vi "Hardware-DI-A-Host.vi"() -> ()   [LabVIEW 2016]
uses:
  <vilib>/Powertrain Controls/Device Drivers/DCM/Rev0/UI/Bank A.ctl
  Shared/Typedefs/DI-Phase-Array-2D.ctl
  <vilib>/Powertrain Controls/Device Drivers/DCM/DI/RT/Phase.ctl
  <vilib>/Powertrain Controls/Device Drivers/DCM/Rev0/FPGA/DI - Drive State.ctl
  <vilib>/Powertrain Controls/Device Drivers/DCM/DI/FPGA/Phase Step.ctl
  <vilib>/Powertrain Controls/Device Drivers/DCM/DI/FPGA/Control.ctl
  <vilib>/Powertrain Controls/Device Drivers/DCM/Rev0/RT/Configuration.ctl
  <vilib>/Powertrain Controls/Device Drivers/DCM/Rev0/FPGA/DI - Bank Configuration.ctl
  Host SubVIs/DI Command Element.ctl
  <vilib>/Powertrain Controls/Device Drivers/DCM/Rev0/FPGA/Digital Channel.ctl
  Shared/Typedefs/DI-Command-Array.ctl
  <vilib>/Powertrain Controls/Device Drivers/DCM/DI/RT/Command.ctl
  <vilib>/Powertrain Controls/Device Drivers/DCM/DI/FPGA/Mode.ctl
  <vilib>/Powertrain Controls/Device Drivers/DCM/DI/RT/Command Sequence.ctl
  <vilib>/Powertrain Controls/Device Drivers/DCM/DI/RT/Angle Control.ctl
  Shared/Typedefs/DI-Phase-Array-1D.ctl
  <vilib>/addons/Software Calibration Management/XControls/SubHost.xctl
  <vilib>/Powertrain Controls/Device Drivers/DCM/Rev0/FPGA/DI - Faults.ctl
  Host SubVIs/Pump Command Element.ctl
  <vilib>/Powertrain Controls/Device Drivers/DCM/Rev0/FPGA/DI - ADC Signals.ctl
  <vilib>/Powertrain Controls/Device Drivers/DCM/DI/FPGA/Capture Event.ctl
  <vilib>/Powertrain Controls/Device Drivers/DCM/Rev0/RT/System State.ctl
  <vilib>/Powertrain Controls/Device Drivers/DCM/Rev0/RT/System ADC.ctl
  <vilib>/Powertrain Controls/Device Drivers/DCM/Rev0/RT/Internal Fault.ctl
  <vilib>/Powertrain Controls/Device Drivers/DCM/Rev0/RT/Run State.ctl
  <vilib>/Powertrain Controls/Device Drivers/DCM/Rev0/UI/Configuration.ctl
  <vilib>/Powertrain Controls/Device Drivers/DCM/Rev0/UI/System Configuration.ctl
  <vilib>/Powertrain Controls/Device Drivers/DCM/Rev0/UI/Injector Configuration.ctl
  <vilib>/Powertrain Controls/Device Drivers/DCM/Rev0/UI/Test Comparators.vi
  <vilib>/Powertrain Controls/Device Drivers/DCM/Rev0/UI/DAC Delay.vi
  <vilib>/Powertrain Controls/Device Drivers/DCM/DI/RT/Phase Convert.vi
  <vilib>/Powertrain Controls/Device Drivers/DCM/DI/RT/Skew.vi
  <vilib>/Powertrain Controls/Device Drivers/DCM/Rev0/UI/Calibrations.vi
  <vilib>/Powertrain Controls/Device Drivers/DCM/Rev0/UI/One Injection Command.vi
  <vilib>/Powertrain Controls/Device Drivers/DCM/DI/FPGA/Simulate Phase Array.vi
  <vilib>/Powertrain Controls/Device Drivers/DCM/Rev0/FPGA/DI - Setpoints.vi
  <vilib>/Powertrain Controls/Device Drivers/DCM/Rev0/UI/Phase State Control.vi
  <vilib>/Powertrain Controls/Device Drivers/DCM/Rev0/UI/Circuit Model Step.vi
  <vilib>/Powertrain Controls/Device Drivers/DCM/Rev0/UI/FET Movie Data.vi
  <vilib>/Powertrain Controls/Device Drivers/DCM/DI/FPGA/DCM - FPGA - DI.lvlib
  <vilib>/Powertrain Controls/Device Drivers/DCM/Rev0/UI/DCM - UI.lvlib
  <vilib>/Powertrain Controls/Device Drivers/DCM/Rev0/FPGA/DCM - FPGA.lvlib
  <vilib>/Powertrain Controls/Device Drivers/DCM/DI/RT/DCM - RT - DI.lvlib
  <vilib>/Powertrain Controls/Device Drivers/DCM/Rev0/RT/DCM - RT.lvclass
  Shared/DSI-Shared.lvlib
panel:
  out "RunState":T1
  out "_BoostSlider":cluster{dbl, dbl, dbl, dbl}(slide)={0.0, 166.94117647058823, 117.76470588235294, 190.23529411764707} scale=0.0..220.0
  out "_Bank A Status":T2 caption="Injector and Pump Simulation Settings" {"Boost Clamp [V]" format="%#_3p"; "Ext HV [V]" format="%#_3p"; "DRVP [V]" format="%#_3p"; "Pump Zener [V]" format="%#_3p"; "DI Zener [V]" format="%#_3p"; "Secondary 3-4 [V]" format="%#_3p"; "Secondary 1-2 [V]" format="%#_3p"; "Primary 3-4 [V]" format="%#_3p"; "Primary 1-2 [V]" format="%#_3p"}
  in  "_DI Bank_Configuration":T3 caption="DI Bank A_Configuration" {"Pump Zener Voltage [V]" min=0 max=240 format="%#_13g"; "DI Zener Voltage [V]" min=0 max=100 format="%#_13g"; "Boost Clamp [V]" min=0 max=220 format="%#_13g"; "Boost Voltage [V]" min=0 max=220 format="%#_13g"}
  in  "DI Scope":T5(xcontrol)
  in  "UserOS":bool
  in  "UserOSTime":sgl caption="[s]" format="%#.3p"
  in  "_Hidden Items":enum32{"DI-A Configurations Items"}(tab)
  out "dt":sgl=13.7
  out "_Bank A?":bool
  in  "_Redraw Slider":bool
  out "SYS|Exec|CalLoading":bool
  in  "_Refresh All":bool
  in  "_Redraw Pump Command":bool
  in  "_Redraw DI Command":bool
  in  "InjCmd":T6=[{"Mode"=enum."Off", "Digital Input"=enum."Unused", "Default Profile Index"=0, "Cal Freq [Hz]"=0.0, "Cal Duration [s]"=0.0, "Cal Increment [s]"=0.0, "Cal Pulses"=0, "TMP Command Sequence"=[{"Duration [s]"=0.0, "Level"=FALSE, "Run/Stop"=FALSE, "Profile Index"=0}, {"Duration [s]"=0.0, "Level"=FALSE, "Run/Stop"=FALSE, "Profile Index"=0}, {"Duration [s]"=0.0, "Level"=FALSE, "Run/Stop"=FALSE, "Profile Index"=0}, {"Duration [s]"=0.0, "Level"=FALSE, "Run/Stop"=FALSE, "Profile Index"=0}, {"Duration [s]"=0.0, "Level"=FALSE, "Run/Stop"=FALSE, "Profile Index"=0}, {"Duration [s]"=0.0, "Level"=FALSE, "Run/Stop"=FALSE, "Profile Index"=0}, {"Duration [s]"=0.0, "Level"=FALSE, "Run/Stop"=FALSE, "Profile Index"=0}, {"Duration [s]"=0.0, "Level"=FALSE, "Run/Stop"=FALSE, "Profile Index"=0}], "EPT TDC Offset [CAD]"=0.0, "EPT Window Start [DBTDC]"=0.0, "EPT Window End [DBTDC]"=0.0, "EPT Angles"=[{"Enable"=FALSE, "Timing [DBTDC]"=0.0, "Duration [s]"=0.0, "Profile Index"=0}, {"Enable"=FALSE, "Timing [DBTDC]"=0.0, "Duration [s]"=0.0, "Profile Index"=0}, {"Enable"=FALSE, "Timing [DBTDC]"=0.0, "Duration [s]"=0.0, "Profile Index"=0}, {"Enable"=FALSE, "Timing [DBTDC]"=0.0, "Duration [s]"=0.0, "Profile Index"=0}], "EPT Skip Fire"=FALSE, "EPT Skip Index"=0, "EPT Precharge Duration [s]"=0.0, "EPT Precharge Profile Index"=0}, {"Mode"=enum."Off", "Digital Input"=enum."Unused", "Default Profile Index"=0, "Cal Freq [Hz]"=0.0, "Cal Duration [s]"=0.0, "Cal Increment [s]"=0.0, "Cal Pulses"=0, "TMP Command Sequence"=[{"Duration [s]"=0.0, "Level"=FALSE, "Run/Stop"=FALSE, "Profile Index"=0}, {"Duration [s]"=0.0, "Level"=FALSE, "Run/Stop"=FALSE, "Profile Index"=0}, {"Duration [s]"=0.0, "Level"=FALSE, "Run/Stop"=FALSE, "Profile Index"=0}, {"Duration [s]"=0.0, "Level"=FALSE, "Run/Stop"=FALSE, "Profile Index"=0}, {"Duration [s]"=0.0, "Level"=FALSE, "Run/Stop"=FALSE, "Profile Index"=0}, {"Duration [s]"=0.0, "Level"=FALSE, "Run/Stop"=FALSE, "Profile Index"=0}, {"Duration [s]"=0.0, "Level"=FALSE, "Run/Stop"=FALSE, "Profile Index"=0}, {"Duration [s]"=0.0, "Level"=FALSE, "Run/Stop"=FALSE, "Profile Index"=0}], "EPT TDC Offset [CAD]"=0.0, "EPT Window Start [DBTDC]"=0.0, "EPT Window End [DBTDC]"=0.0, "EPT Angles"=[{"Enable"=FALSE, "Timing [DBTDC]"=0.0, "Duration [s]"=0.0, "Profile Index"=0}, {"Enable"=FALSE, "Timing [DBTDC]"=0.0, "Duration [s]"=0.0, "Profile Index"=0}, {"Enable"=FALSE, "Timing [DBTDC]"=0.0, "Duration [s]"=0.0, "Profile Index"=0}, {"Enable"=FALSE, "Timing [DBTDC]"=0.0, "Duration [s]"=0.0, "Profile Index"=0}], "EPT Skip Fire"=FALSE, "EPT Skip Index"=0, "EPT Precharge Duration [s]"=0.0, "EPT Precharge Profile Index"=0}, {"Mode"=enum."Off", "Digital Input"=enum."Unused", "Default Profile Index"=0, "Cal Freq [Hz]"=0.0, "Cal Duration [s]"=0.0, "Cal Increment [s]"=0.0, "Cal Pulses"=0, "TMP Command Sequence"=[{"Duration [s]"=0.0, "Level"=FALSE, "Run/Stop"=FALSE, "Profile Index"=0}, {"Duration [s]"=0.0, "Level"=FALSE, "Run/Stop"=FALSE, "Profile Index"=0}, {"Duration [s]"=0.0, "Level"=FALSE, "Run/Stop"=FALSE, "Profile Index"=0}, {"Duration [s]"=0.0, "Level"=FALSE, "Run/Stop"=FALSE, "Profile Index"=0}, {"Duration [s]"=0.0, "Level"=FALSE, "Run/Stop"=FALSE, "Profile Index"=0}, {"Duration [s]"=0.0, "Level"=FALSE, "Run/Stop"=FALSE, "Profile Index"=0}, {"Duration [s]"=0.0, "Level"=FALSE, "Run/Stop"=FALSE, "Profile Index"=0}, {"Duration [s]"=0.0, "Level"=FALSE, "Run/Stop"=FALSE, "Profile Index"=0}], "EPT TDC Offset [CAD]"=0.0, "EPT Window Start [DBTDC]"=0.0, "EPT Window End [DBTDC]"=0.0, "EPT Angles"=[{"Enable"=FALSE, "Timing [DBTDC]"=0.0, "Duration [s]"=0.0, "Profile Index"=0}, {"Enable"=FALSE, "Timing [DBTDC]"=0.0, "Duration [s]"=0.0, "Profile Index"=0}, {"Enable"=FALSE, "Timing [DBTDC]"=0.0, "Duration [s]"=0.0, "Profile Index"=0}, {"Enable"=FALSE, "Timing [DBTDC]"=0.0, "Duration [s]"=0.0, "Profile Index"=0}], "EPT Skip Fire"=FALSE, "EPT Skip Index"=0, "EPT Precharge Duration [s]"=0.0, "EPT Precharge Profile Index"=0}, {"Mode"=enum."Off", "Digital Input"=enum."Unused", "Default Profile Index"=0, "Cal Freq [Hz]"=0.0, "Cal Duration [s]"=0.0, "Cal Increment [s]"=0.0, "Cal Pulses"=0, "TMP Command Sequence"=[{"Duration [s]"=0.0, "Level"=FALSE, "Run/Stop"=FALSE, "Profile Index"=0}, {"Duration [s]"=0.0, "Level"=FALSE, "Run/Stop"=FALSE, "Profile Index"=0}, {"Duration [s]"=0.0, "Level"=FALSE, "Run/Stop"=FALSE, "Profile Index"=0}, {"Duration [s]"=0.0, "Level"=FALSE, "Run/Stop"=FALSE, "Profile Index"=0}, {"Duration [s]"=0.0, "Level"=FALSE, "Run/Stop"=FALSE, "Profile Index"=0}, {"Duration [s]"=0.0, "Level"=FALSE, "Run/Stop"=FALSE, "Profile Index"=0}, {"Duration [s]"=0.0, "Level"=FALSE, "Run/Stop"=FALSE, "Profile Index"=0}, {"Duration [s]"=0.0, "Level"=FALSE, "Run/Stop"=FALSE, "Profile Index"=0}], "EPT TDC Offset [CAD]"=0.0, "EPT Window Start [DBTDC]"=0.0, "EPT Window End [DBTDC]"=0.0, "EPT Angles"=[{"Enable"=FALSE, "Timing [DBTDC]"=0.0, "Duration [s]"=0.0, "Profile Index"=0}, {"Enable"=FALSE, "Timing [DBTDC]"=0.0, "Duration [s]"=0.0, "Profile Index"=0}, {"Enable"=FALSE, "Timing [DBTDC]"=0.0, "Duration [s]"=0.0, "Profile Index"=0}, {"Enable"=FALSE, "Timing [DBTDC]"=0.0, "Duration [s]"=0.0, "Profile Index"=0}], "EPT Skip Fire"=FALSE, "EPT Skip Index"=0, "EPT Precharge Duration [s]"=0.0, "EPT Precharge Profile Index"=0}, {"Mode"=enum."Off", "Digital Input"=enum."Unused", "Default Profile Index"=0, "Cal Freq [Hz]"=0.0, "Cal Duration [s]"=0.0, "Cal Increment [s]"=0.0, "Cal Pulses"=0, "TMP Command Sequence"=[{"Duration [s]"=0.0, "Level"=FALSE, "Run/Stop"=FALSE, "Profile Index"=0}, {"Duration [s]"=0.0, "Level"=FALSE, "Run/Stop"=FALSE, "Profile Index"=0}, {"Duration [s]"=0.0, "Level"=FALSE, "Run/Stop"=FALSE, "Profile Index"=0}, {"Duration [s]"=0.0, "Level"=FALSE, "Run/Stop"=FALSE, "Profile Index"=0}, {"Duration [s]"=0.0, "Level"=FALSE, "Run/Stop"=FALSE, "Profile Index"=0}, {"Duration [s]"=0.0, "Level"=FALSE, "Run/Stop"=FALSE, "Profile Index"=0}, {"Duration [s]"=0.0, "Level"=FALSE, "Run/Stop"=FALSE, "Profile Index"=0}, {"Duration [s]"=0.0, "Level"=FALSE, "Run/Stop"=FALSE, "Profile Index"=0}], "EPT TDC Offset [CAD]"=0.0, "EPT Window Start [DBTDC]"=0.0, "EPT Window End [DBTDC]"=0.0, "EPT Angles"=[{"Enable"=FALSE, "Timing [DBTDC]"=0.0, "Duration [s]"=0.0, "Profile Index"=0}, {"Enable"=FALSE, "Timing [DBTDC]"=0.0, "Duration [s]"=0.0, "Profile Index"=0}, {"Enable"=FALSE, "Timing [DBTDC]"=0.0, "Duration [s]"=0.0, "Profile Index"=0}, {"Enable"=FALSE, "Timing [DBTDC]"=0.0, "Duration [s]"=0.0, "Profile Index"=0}], "EPT Skip Fire"=FALSE, "EPT Skip Index"=0, "EPT Precharge Duration [s]"=0.0, "EPT Precharge Profile Index"=0}, {"Mode"=enum."Off", "Digital Input"=enum."Unused", "Default Profile Index"=0, "Cal Freq [Hz]"=0.0, "Cal Duration [s]"=0.0, "Cal Increment [s]"=0.0, "Cal Pulses"=0, "TMP Command Sequence"=[{"Duration [s]"=0.0, "Level"=FALSE, "Run/Stop"=FALSE, "Profile Index"=0}, {"Duration [s]"=0.0, "Level"=FALSE, "Run/Stop"=FALSE, "Profile Index"=0}, {"Duration [s]"=0.0, "Level"=FALSE, "Run/Stop"=FALSE, "Profile Index"=0}, {"Duration [s]"=0.0, "Level"=FALSE, "Run/Stop"=FALSE, "Profile Index"=0}, {"Duration [s]"=0.0, "Level"=FALSE, "Run/Stop"=FALSE, "Profile Index"=0}, {"Duration [s]"=0.0, "Level"=FALSE, "Run/Stop"=FALSE, "Profile Index"=0}, {"Duration [s]"=0.0, "Level"=FALSE, "Run/Stop"=FALSE, "Profile Index"=0}, {"Duration [s]"=0.0, "Level"=FALSE, "Run/Stop"=FALSE, "Profile Index"=0}], "EPT TDC Offset [CAD]"=0.0, "EPT Window Start [DBTDC]"=0.0, "EPT Window End [DBTDC]"=0.0, "EPT Angles"=[{"Enable"=FALSE, "Timing [DBTDC]"=0.0, "Duration [s]"=0.0, "Profile Index"=0}, {"Enable"=FALSE, "Timing [DBTDC]"=0.0, "Duration [s]"=0.0, "Profile Index"=0}, {"Enable"=FALSE, "Timing [DBTDC]"=0.0, "Duration [s]"=0.0, "Profile Index"=0}, {"Enable"=FALSE, "Timing [DBTDC]"=0.0, "Duration [s]"=0.0, "Profile Index"=0}], "EPT Skip Fire"=FALSE, "EPT Skip Index"=0, "EPT Precharge Duration [s]"=0.0, "EPT Precharge Profile Index"=0}, {"Mode"=enum."Off", "Digital Input"=enum."Unused", "Default Profile Index"=0, "Cal Freq [Hz]"=0.0, "Cal Duration [s]"=0.0, "Cal Increment [s]"=0.0, "Cal Pulses"=0, "TMP Command Sequence"=[{"Duration [s]"=0.0, "Level"=FALSE, "Run/Stop"=FALSE, "Profile Index"=0}, {"Duration [s]"=0.0, "Level"=FALSE, "Run/Stop"=FALSE, "Profile Index"=0}, {"Duration [s]"=0.0, "Level"=FALSE, "Run/Stop"=FALSE, "Profile Index"=0}, {"Duration [s]"=0.0, "Level"=FALSE, "Run/Stop"=FALSE, "Profile Index"=0}, {"Duration [s]"=0.0, "Level"=FALSE, "Run/Stop"=FALSE, "Profile Index"=0}, {"Duration [s]"=0.0, "Level"=FALSE, "Run/Stop"=FALSE, "Profile Index"=0}, {"Duration [s]"=0.0, "Level"=FALSE, "Run/Stop"=FALSE, "Profile Index"=0}, {"Duration [s]"=0.0, "Level"=FALSE, "Run/Stop"=FALSE, "Profile Index"=0}], "EPT TDC Offset [CAD]"=0.0, "EPT Window Start [DBTDC]"=0.0, "EPT Window End [DBTDC]"=0.0, "EPT Angles"=[{"Enable"=FALSE, "Timing [DBTDC]"=0.0, "Duration [s]"=0.0, "Profile Index"=0}, {"Enable"=FALSE, "Timing [DBTDC]"=0.0, "Duration [s]"=0.0, "Profile Index"=0}, {"Enable"=FALSE, "Timing [DBTDC]"=0.0, "Duration [s]"=0.0, "Profile Index"=0}, {"Enable"=FALSE, "Timing [DBTDC]"=0.0, "Duration [s]"=0.0, "Profile Index"=0}], "EPT Skip Fire"=FALSE, "EPT Skip Index"=0, "EPT Precharge Duration [s]"=0.0, "EPT Precharge Profile Index"=0}, {"Mode"=enum."Off", "Digital Input"=enum."Unused", "Default Profile Index"=0, "Cal Freq [Hz]"=0.0, "Cal Duration [s]"=0.0, "Cal Increment [s]"=0.0, "Cal Pulses"=0, "TMP Command Sequence"=[{"Duration [s]"=0.0, "Level"=FALSE, "Run/Stop"=FALSE, "Profile Index"=0}, {"Duration [s]"=0.0, "Level"=FALSE, "Run/Stop"=FALSE, "Profile Index"=0}, {"Duration [s]"=0.0, "Level"=FALSE, "Run/Stop"=FALSE, "Profile Index"=0}, {"Duration [s]"=0.0, "Level"=FALSE, "Run/Stop"=FALSE, "Profile Index"=0}, {"Duration [s]"=0.0, "Level"=FALSE, "Run/Stop"=FALSE, "Profile Index"=0}, {"Duration [s]"=0.0, "Level"=FALSE, "Run/Stop"=FALSE, "Profile Index"=0}, {"Duration [s]"=0.0, "Level"=FALSE, "Run/Stop"=FALSE, "Profile Index"=0}, {"Duration [s]"=0.0, "Level"=FALSE, "Run/Stop"=FALSE, "Profile Index"=0}], "EPT TDC Offset [CAD]"=0.0, "EPT Window Start [DBTDC]"=0.0, "EPT Window End [DBTDC]"=0.0, "EPT Angles"=[{"Enable"=FALSE, "Timing [DBTDC]"=0.0, "Duration [s]"=0.0, "Profile Index"=0}, {"Enable"=FALSE, "Timing [DBTDC]"=0.0, "Duration [s]"=0.0, "Profile Index"=0}, {"Enable"=FALSE, "Timing [DBTDC]"=0.0, "Duration [s]"=0.0, "Profile Index"=0}, {"Enable"=FALSE, "Timing [DBTDC]"=0.0, "Duration [s]"=0.0, "Profile Index"=0}], "EPT Skip Fire"=FALSE, "EPT Skip Index"=0, "EPT Precharge Duration [s]"=0.0, "EPT Precharge Profile Index"=0}] {"EPT Precharge Profile Index" max=15; "EPT Precharge Duration [s]" min=0 format="%#_4p"; "Default Profile Index" max=15; "Cal Increment [s]" format="%#_3p"; "TMP Command Sequence"."Profile Index" max=7; "TMP Command Sequence"."Duration [s]" min=0 max=100 format="%#_3p"; "Cal Pulses" max=511; "EPT Skip Index" max=7; "EPT Angles"."Profile Index" max=7; "EPT Angles"."Duration [s]" min=0 max=100 format="%#_3p"; "Cal Duration [s]" format="%#_3p"; "Cal Freq [Hz]" format="%#_3p"}
  in  "ChanSelect4":u8(ring) items=["I LS A1/A5", "I LS A2/A6", "I LS A3/A7", "I LS A4", "I LS A8/PumpA", "V PZ A1", "V PZ A2", "V PZ A3", "V PZ A4", "V S A1", "V S A2", "V S A3", "V S A4", "V S A5", "V S A6", "V S A7", "V S A8", "V Pump A", "V Secondary A1A2", "V Secondary A3A4", "V Ext HV A", "------------------------ ", "I LS B1/B5", "I LS B2/B6", "I LS B3/B7", "I LS B4", "I LS B8/PumpB", "V PZ B1", "V PZ B2", "V PZ B3", "V PZ B4", "V S B1", "V S B2", "V S B3", "V S B4", "V S B5", "V S B6", "V S B7", "V S B8", "V Pump B", "V Secondary B1B2", "V Secondary B3B4", "V Ext HV B", "-------------------------  ", "AI 1", "AI 2", "AI 3", "AI 4", "AI 5", "AI 6", "AI 7", "AI 8", "AI 9", "AI 10", "AI 11", "AI 12", "-------------------------   ", "V DRVP"]
  in  "ChanSelect3":u8(ring) items=["I LS A1/A5", "I LS A2/A6", "I LS A3/A7", "I LS A4", "I LS A8/PumpA", "V PZ A1", "V PZ A2", "V PZ A3", "V PZ A4", "V S A1", "V S A2", "V S A3", "V S A4", "V S A5", "V S A6", "V S A7", "V S A8", "V Pump A", "V Secondary A1A2", "V Secondary A3A4", "V Ext HV A", "------------------------ ", "I LS B1/B5", "I LS B2/B6", "I LS B3/B7", "I LS B4", "I LS B8/PumpB", "V PZ B1", "V PZ B2", "V PZ B3", "V PZ B4", "V S B1", "V S B2", "V S B3", "V S B4", "V S B5", "V S B6", "V S B7", "V S B8", "V Pump B", "V Secondary B1B2", "V Secondary B3B4", "V Ext HV B", "-------------------------  ", "AI 1", "AI 2", "AI 3", "AI 4", "AI 5", "AI 6", "AI 7", "AI 8", "AI 9", "AI 10", "AI 11", "AI 12", "-------------------------   ", "V DRVP"]
  in  "_Redraw Profiles Usage Tracker":bool
  in  "_Redraw Pump Timing Plot":bool
  in  "InjectEnable":bool
  in  "PSEnable":bool
  in  "Configuration":u8
  in  "BoostV":sgl format="%#_13g"
  in  "ZenerV":sgl format="%#_13g"
  in  "ZenerEnable":bool
  in  "PumpZenerV":sgl format="%#_13g"
  in  "BoostClampV":sgl format="%#_13g"
  in  "_Redraw Phase":bool
  in  "_Redraw Phase Plot":bool
  in  "_Redraw Phase Lists":bool
  in  "_Redraw Pump Phase Plot":bool
  in  "_Redraw Pump Phase List":bool
  in  "FaultClear":u8
  in  "ChanSelect2":u8(ring) items=["I LS A1/A5", "I LS A2/A6", "I LS A3/A7", "I LS A4", "I LS A8/PumpA", "V PZ A1", "V PZ A2", "V PZ A3", "V PZ A4", "V S A1", "V S A2", "V S A3", "V S A4", "V S A5", "V S A6", "V S A7", "V S A8", "V Pump A", "V Secondary A1A2", "V Secondary A3A4", "V Ext HV A", "------------------------ ", "I LS B1/B5", "I LS B2/B6", "I LS B3/B7", "I LS B4", "I LS B8/PumpB", "V PZ B1", "V PZ B2", "V PZ B3", "V PZ B4", "V S B1", "V S B2", "V S B3", "V S B4", "V S B5", "V S B6", "V S B7", "V S B8", "V Pump B", "V Secondary B1B2", "V Secondary B3B4", "V Ext HV B", "-------------------------  ", "AI 1", "AI 2", "AI 3", "AI 4", "AI 5", "AI 6", "AI 7", "AI 8", "AI 9", "AI 10", "AI 11", "AI 12", "-------------------------   ", "V DRVP"]
  in  "ChanSelect1":u8(ring) items=["I LS A1/A5", "I LS A2/A6", "I LS A3/A7", "I LS A4", "I LS A8/PumpA", "V PZ A1", "V PZ A2", "V PZ A3", "V PZ A4", "V S A1", "V S A2", "V S A3", "V S A4", "V S A5", "V S A6", "V S A7", "V S A8", "V Pump A", "V Secondary A1A2", "V Secondary A3A4", "V Ext HV A", "------------------------ ", "I LS B1/B5", "I LS B2/B6", "I LS B3/B7", "I LS B4", "I LS B8/PumpB", "V PZ B1", "V PZ B2", "V PZ B3", "V PZ B4", "V S B1", "V S B2", "V S B3", "V S B4", "V S B5", "V S B6", "V S B7", "V S B8", "V Pump B", "V Secondary B1B2", "V Secondary B3B4", "V Ext HV B", "-------------------------  ", "AI 1", "AI 2", "AI 3", "AI 4", "AI 5", "AI 6", "AI 7", "AI 8", "AI 9", "AI 10", "AI 11", "AI 12", "-------------------------   ", "V DRVP"]
  in  "ScopeEnable":bool
  in  "ScopeEvent":u8(ring) items=["Unused", "Injector A1", "Injector A2", "Injector A3", "Injector A4", "Injector A5", "Injector A6", "Injector A7", "Injector A8/PumpA", "Injector B1", "Injector B2", "Injector B3", "Injector B4", "Injector B5", "Injector B6", "Injector B7", "Injector B8/PumpB", "Diff IO 1", "Diff IO 2", "Diff IO 3", "Diff IO 4", "Diff IO 5", "Diff IO 6", "Diff IO 7", "Diff IO 8", "Aux 1", "Aux 2", "Aux 3", "Aux 4", "Aux 5", "Aux 6", "Aux 7", "Aux 8", "User OS"]
  out "Data":sgl[][](array[numeric])
  out "_Ref Pump Profiles":cluster{"Array":dbl[], "Array":dbl[]}[](array[cluster])
  out "_Ref Inj Profiles":cluster{"Array":dbl[], "Array":dbl[]}[](array[cluster])
  out "_SimuXY":cluster{"Array":dbl[], "Array":dbl[]}[](array[cluster])
  in  "PumpPhase":T12=[{"Drive"=enum."Idle", "Direction"=FALSE, "Phase Step"=enum."Duration", "Duration [s]"=0.0, "Current High [A]"=0.0, "Current Low [A]"=0.0, "Voltage High [V]"=0.0, "Voltage Low [V]"=0.0, "Change"=FALSE, "Current Control"=enum."Closed Loop", "Period [s]"=0.0, "Pulse Width [s]"=0.0, "Profile"=0, "Voltage Control"=FALSE}, {"Drive"=enum."Idle", "Direction"=FALSE, "Phase Step"=enum."Duration", "Duration [s]"=0.0, "Current High [A]"=0.0, "Current Low [A]"=0.0, "Voltage High [V]"=0.0, "Voltage Low [V]"=0.0, "Change"=FALSE, "Current Control"=enum."Closed Loop", "Period [s]"=0.0, "Pulse Width [s]"=0.0, "Profile"=0, "Voltage Control"=FALSE}, {"Drive"=enum."Idle", "Direction"=FALSE, "Phase Step"=enum."Duration", "Duration [s]"=0.0, "Current High [A]"=0.0, "Current Low [A]"=0.0, "Voltage High [V]"=0.0, "Voltage Low [V]"=0.0, "Change"=FALSE, "Current Control"=enum."Closed Loop", "Period [s]"=0.0, "Pulse Width [s]"=0.0, "Profile"=0, "Voltage Control"=FALSE}, {"Drive"=enum."Idle", "Direction"=FALSE, "Phase Step"=enum."Duration", "Duration [s]"=0.0, "Current High [A]"=0.0, "Current Low [A]"=0.0, "Voltage High [V]"=0.0, "Voltage Low [V]"=0.0, "Change"=FALSE, "Current Control"=enum."Closed Loop", "Period [s]"=0.0, "Pulse Width [s]"=0.0, "Profile"=0, "Voltage Control"=FALSE}, {"Drive"=enum."Idle", "Direction"=FALSE, "Phase Step"=enum."Duration", "Duration [s]"=0.0, "Current High [A]"=0.0, "Current Low [A]"=0.0, "Voltage High [V]"=0.0, "Voltage Low [V]"=0.0, "Change"=FALSE, "Current Control"=enum."Closed Loop", "Period [s]"=0.0, "Pulse Width [s]"=0.0, "Profile"=0, "Voltage Control"=FALSE}, {"Drive"=enum."Idle", "Direction"=FALSE, "Phase Step"=enum."Duration", "Duration [s]"=0.0, "Current High [A]"=0.0, "Current Low [A]"=0.0, "Voltage High [V]"=0.0, "Voltage Low [V]"=0.0, "Change"=FALSE, "Current Control"=enum."Closed Loop", "Period [s]"=0.0, "Pulse Width [s]"=0.0, "Profile"=0, "Voltage Control"=FALSE}, {"Drive"=enum."Idle", "Direction"=FALSE, "Phase Step"=enum."Duration", "Duration [s]"=0.0, "Current High [A]"=0.0, "Current Low [A]"=0.0, "Voltage High [V]"=0.0, "Voltage Low [V]"=0.0, "Change"=FALSE, "Current Control"=enum."Closed Loop", "Period [s]"=0.0, "Pulse Width [s]"=0.0, "Profile"=0, "Voltage Control"=FALSE}, {"Drive"=enum."Idle", "Direction"=FALSE, "Phase Step"=enum."Duration", "Duration [s]"=0.0, "Current High [A]"=0.0, "Current Low [A]"=0.0, "Voltage High [V]"=0.0, "Voltage Low [V]"=0.0, "Change"=FALSE, "Current Control"=enum."Closed Loop", "Period [s]"=0.0, "Pulse Width [s]"=0.0, "Profile"=0, "Voltage Control"=FALSE}, {"Drive"=enum."Idle", "Direction"=FALSE, "Phase Step"=enum."Duration", "Duration [s]"=0.0, "Current High [A]"=0.0, "Current Low [A]"=0.0, "Voltage High [V]"=0.0, "Voltage Low [V]"=0.0, "Change"=FALSE, "Current Control"=enum."Closed Loop", "Period [s]"=0.0, "Pulse Width [s]"=0.0, "Profile"=0, "Voltage Control"=FALSE}, {"Drive"=enum."Idle", "Direction"=FALSE, "Phase Step"=enum."Duration", "Duration [s]"=0.0, "Current High [A]"=0.0, "Current Low [A]"=0.0, "Voltage High [V]"=0.0, "Voltage Low [V]"=0.0, "Change"=FALSE, "Current Control"=enum."Closed Loop", "Period [s]"=0.0, "Pulse Width [s]"=0.0, "Profile"=0, "Voltage Control"=FALSE}, {"Drive"=enum."Idle", "Direction"=FALSE, "Phase Step"=enum."Duration", "Duration [s]"=0.0, "Current High [A]"=0.0, "Current Low [A]"=0.0, "Voltage High [V]"=0.0, "Voltage Low [V]"=0.0, "Change"=FALSE, "Current Control"=enum."Closed Loop", "Period [s]"=0.0, "Pulse Width [s]"=0.0, "Profile"=0, "Voltage Control"=FALSE}, {"Drive"=enum."Idle", "Direction"=FALSE, "Phase Step"=enum."Duration", "Duration [s]"=0.0, "Current High [A]"=0.0, "Current Low [A]"=0.0, "Voltage High [V]"=0.0, "Voltage Low [V]"=0.0, "Change"=FALSE, "Current Control"=enum."Closed Loop", "Period [s]"=0.0, "Pulse Width [s]"=0.0, "Profile"=0, "Voltage Control"=FALSE}, {"Drive"=enum."Idle", "Direction"=FALSE, "Phase Step"=enum."Duration", "Duration [s]"=0.0, "Current High [A]"=0.0, "Current Low [A]"=0.0, "Voltage High [V]"=0.0, "Voltage Low [V]"=0.0, "Change"=FALSE, "Current Control"=enum."Closed Loop", "Period [s]"=0.0, "Pulse Width [s]"=0.0, "Profile"=0, "Voltage Control"=FALSE}, {"Drive"=enum."Idle", "Direction"=FALSE, "Phase Step"=enum."Duration", "Duration [s]"=0.0, "Current High [A]"=0.0, "Current Low [A]"=0.0, "Voltage High [V]"=0.0, "Voltage Low [V]"=0.0, "Change"=FALSE, "Current Control"=enum."Closed Loop", "Period [s]"=0.0, "Pulse Width [s]"=0.0, "Profile"=0, "Voltage Control"=FALSE}, {"Drive"=enum."Idle", "Direction"=FALSE, "Phase Step"=enum."Duration", "Duration [s]"=0.0, "Current High [A]"=0.0, "Current Low [A]"=0.0, "Voltage High [V]"=0.0, "Voltage Low [V]"=0.0, "Change"=FALSE, "Current Control"=enum."Closed Loop", "Period [s]"=0.0, "Pulse Width [s]"=0.0, "Profile"=0, "Voltage Control"=FALSE}, {"Drive"=enum."Idle", "Direction"=FALSE, "Phase Step"=enum."Duration", "Duration [s]"=0.0, "Current High [A]"=0.0, "Current Low [A]"=0.0, "Voltage High [V]"=0.0, "Voltage Low [V]"=0.0, "Change"=FALSE, "Current Control"=enum."Closed Loop", "Period [s]"=0.0, "Pulse Width [s]"=0.0, "Profile"=0, "Voltage Control"=FALSE}] caption="Pump A Phase Arrays" {"Profile" max=15; "Period [s]" min=4e-06 max=0.000102 format="%#_3p"; "Pulse Width [s]" min=0 max=0.000102 format="%#_3p"; "Voltage Low [V]" min=-220 max=220 format="%#_3p"; "Voltage High [V]" min=-220 max=220 format="%#_3p"; "Current Low [A]" min=-40 max=40 format="%#_3p"; "Current High [A]" min=-40 max=40 format="%#_3p"; "Duration [s]" min=0 max=1.67772 format="%#_3p"}
  in  "_Redraw Timing Plot":bool
  in  "_Redraw Injection List":bool
  in  "InjAdaptMode":u32
  in  "InjPhasePlotColors":sgl[](array[numeric])
  in  "RefInjTimeAxisMultiplier":sgl
  in  "RefInjTimeAxisOffset":sgl
  in  "RefInjCurrentMultiplier":sgl
  in  "RefInjCurrentOffset":sgl
  in  "RefInjVoltageMultiplier":sgl
  in  "RefInjVoltageOffset":sgl
  in  "RefPumpTimeAxisMultiplier":sgl
  in  "RefPumpTimeAxisOffset":sgl
  in  "RefPumpCurrentMultiplier":sgl
  in  "RefPumpCurrentOffset":sgl
  in  "RefPumpVoltageMultiplier":sgl
  in  "RefPumpVoltageOffset":sgl
  in  "InjPhasePlotLineWidths":sgl[](array[numeric])
  in  "InjPhasePlotLineTypes":sgl[](array[numeric])
  in  "InjCmdPlotColors":sgl[](array[numeric])
  in  "InjCmdPlotLineWidths":sgl[](array[numeric])
  in  "InjCmdPlotLineTypes":sgl[](array[numeric])
  in  "PumpPhasePlotColors":sgl[](array[numeric])
  in  "PumpPhasePlotLineWidths":sgl[](array[numeric])
  in  "PumpPhasePlotLineTypes":sgl[](array[numeric])
  in  "PumpCmdPlotColors":sgl[](array[numeric])
  in  "PumpCmdPlotLineWidths":sgl[](array[numeric])
  in  "PumpCmdPlotLineTypes":sgl[](array[numeric])
  in  "PumpCapacitance":sgl=5e-06 format="%#_6p"
  in  "PumpInductance":sgl=0.0001 format="%#_6p"
  in  "PumpResistance":sgl=1.0 format="%#_6p"
  in  "SimSpeed":sgl=5e-06 format="%#_6p"
  in  "SimRotations":u8
  in  "InjCapacitance":sgl=5e-06 format="%#_6p"
  in  "InjInductance":sgl=0.0001 format="%#_6p"
  in  "InjResistance":sgl=1.0 format="%#_6p"
  in  "SimBatt":sgl=13.7 min=6 max=32
  in  "_Redraw Pump Phase":bool
  in  "InjPhase":T17=[[{"Drive"=enum."Idle", "Direction"=FALSE, "Phase Step"=enum."Duration", "Duration [s]"=0.0, "Current High [A]"=0.0, "Current Low [A]"=0.0, "Voltage High [V]"=0.0, "Voltage Low [V]"=0.0, "Change"=FALSE, "Current Control"=enum."Closed Loop", "Period [s]"=0.0, "Pulse Width [s]"=0.0, "Profile"=0, "Voltage Control"=FALSE}, {"Drive"=enum."Idle", "Direction"=FALSE, "Phase Step"=enum."Duration", "Duration [s]"=0.0, "Current High [A]"=0.0, "Current Low [A]"=0.0, "Voltage High [V]"=0.0, "Voltage Low [V]"=0.0, "Change"=FALSE, "Current Control"=enum."Closed Loop", "Period [s]"=0.0, "Pulse Width [s]"=0.0, "Profile"=0, "Voltage Control"=FALSE}, {"Drive"=enum."Idle", "Direction"=FALSE, "Phase Step"=enum."Duration", "Duration [s]"=0.0, "Current High [A]"=0.0, "Current Low [A]"=0.0, "Voltage High [V]"=0.0, "Voltage Low [V]"=0.0, "Change"=FALSE, "Current Control"=enum."Closed Loop", "Period [s]"=0.0, "Pulse Width [s]"=0.0, "Profile"=0, "Voltage Control"=FALSE}, {"Drive"=enum."Idle", "Direction"=FALSE, "Phase Step"=enum."Duration", "Duration [s]"=0.0, "Current High [A]"=0.0, "Current Low [A]"=0.0, "Voltage High [V]"=0.0, "Voltage Low [V]"=0.0, "Change"=FALSE, "Current Control"=enum."Closed Loop", "Period [s]"=0.0, "Pulse Width [s]"=0.0, "Profile"=0, "Voltage Control"=FALSE}, {"Drive"=enum."Idle", "Direction"=FALSE, "Phase Step"=enum."Duration", "Duration [s]"=0.0, "Current High [A]"=0.0, "Current Low [A]"=0.0, "Voltage High [V]"=0.0, "Voltage Low [V]"=0.0, "Change"=FALSE, "Current Control"=enum."Closed Loop", "Period [s]"=0.0, "Pulse Width [s]"=0.0, "Profile"=0, "Voltage Control"=FALSE}, {"Drive"=enum."Idle", "Direction"=FALSE, "Phase Step"=enum."Duration", "Duration [s]"=0.0, "Current High [A]"=0.0, "Current Low [A]"=0.0, "Voltage High [V]"=0.0, "Voltage Low [V]"=0.0, "Change"=FALSE, "Current Control"=enum."Closed Loop", "Period [s]"=0.0, "Pulse Width [s]"=0.0, "Profile"=0, "Voltage Control"=FALSE}, {"Drive"=enum."Idle", "Direction"=FALSE, "Phase Step"=enum."Duration", "Duration [s]"=0.0, "Current High [A]"=0.0, "Current Low [A]"=0.0, "Voltage High [V]"=0.0, "Voltage Low [V]"=0.0, "Change"=FALSE, "Current Control"=enum."Closed Loop", "Period [s]"=0.0, "Pulse Width [s]"=0.0, "Profile"=0, "Voltage Control"=FALSE}, {"Drive"=enum."Idle", "Direction"=FALSE, "Phase Step"=enum."Duration", "Duration [s]"=0.0, "Current High [A]"=0.0, "Current Low [A]"=0.0, "Voltage High [V]"=0.0, "Voltage Low [V]"=0.0, "Change"=FALSE, "Current Control"=enum."Closed Loop", "Period [s]"=0.0, "Pulse Width [s]"=0.0, "Profile"=0, "Voltage Control"=FALSE}, {"Drive"=enum."Idle", "Direction"=FALSE, "Phase Step"=enum."Duration", "Duration [s]"=0.0, "Current High [A]"=0.0, "Current Low [A]"=0.0, "Voltage High [V]"=0.0, "Voltage Low [V]"=0.0, "Change"=FALSE, "Current Control"=enum."Closed Loop", "Period [s]"=0.0, "Pulse Width [s]"=0.0, "Profile"=0, "Voltage Control"=FALSE}, {"Drive"=enum."Idle", "Direction"=FALSE, "Phase Step"=enum."Duration", "Duration [s]"=0.0, "Current High [A]"=0.0, "Current Low [A]"=0.0, "Voltage High [V]"=0.0, "Voltage Low [V]"=0.0, "Change"=FALSE, "Current Control"=enum."Closed Loop", "Period [s]"=0.0, "Pulse Width [s]"=0.0, "Profile"=0, "Voltage Control"=FALSE}, {"Drive"=enum."Idle", "Direction"=FALSE, "Phase Step"=enum."Duration", "Duration [s]"=0.0, "Current High [A]"=0.0, "Current Low [A]"=0.0, "Voltage High [V]"=0.0, "Voltage Low [V]"=0.0, "Change"=FALSE, "Current Control"=enum."Closed Loop", "Period [s]"=0.0, "Pulse Width [s]"=0.0, "Profile"=0, "Voltage Control"=FALSE}, {"Drive"=enum."Idle", "Direction"=FALSE, "Phase Step"=enum."Duration", "Duration [s]"=0.0, "Current High [A]"=0.0, "Current Low [A]"=0.0, "Voltage High [V]"=0.0, "Voltage Low [V]"=0.0, "Change"=FALSE, "Current Control"=enum."Closed Loop", "Period [s]"=0.0, "Pulse Width [s]"=0.0, "Profile"=0, "Voltage Control"=FALSE}, {"Drive"=enum."Idle", "Direction"=FALSE, "Phase Step"=enum."Duration", "Duration [s]"=0.0, "Current High [A]"=0.0, "Current Low [A]"=0.0, "Voltage High [V]"=0.0, "Voltage Low [V]"=0.0, "Change"=FALSE, "Current Control"=enum."Closed Loop", "Period [s]"=0.0, "Pulse Width [s]"=0.0, "Profile"=0, "Voltage Control"=FALSE}, {"Drive"=enum."Idle", "Direction"=FALSE, "Phase Step"=enum."Duration", "Duration [s]"=0.0, "Current High [A]"=0.0, "Current Low [A]"=0.0, "Voltage High [V]"=0.0, "Voltage Low [V]"=0.0, "Change"=FALSE, "Current Control"=enum."Closed Loop", "Period [s]"=0.0, "Pulse Width [s]"=0.0, "Profile"=0, "Voltage Control"=FALSE}, {"Drive"=enum."Idle", "Direction"=FALSE, "Phase Step"=enum."Duration", "Duration [s]"=0.0, "Current High [A]"=0.0, "Current Low [A]"=0.0, "Voltage High [V]"=0.0, "Voltage Low [V]"=0.0, "Change"=FALSE, "Current Control"=enum."Closed Loop", "Period [s]"=0.0, "Pulse Width [s]"=0.0, "Profile"=0, "Voltage Control"=FALSE}, {"Drive"=enum."Idle", "Direction"=FALSE, "Phase Step"=enum."Duration", "Duration [s]"=0.0, "Current High [A]"=0.0, "Current Low [A]"=0.0, "Voltage High [V]"=0.0, "Voltage Low [V]"=0.0, "Change"=FALSE, "Current Control"=enum."Closed Loop", "Period [s]"=0.0, "Pulse Width [s]"=0.0, "Profile"=0, "Voltage Control"=FALSE}], [{"Drive"=enum."Idle", "Direction"=FALSE, "Phase Step"=enum."Duration", "Duration [s]"=0.0, "Current High [A]"=0.0, "Current Low [A]"=0.0, "Voltage High [V]"=0.0, "Voltage Low [V]"=0.0, "Change"=FALSE, "Current Control"=enum."Closed Loop", "Period [s]"=0.0, "Pulse Width [s]"=0.0, "Profile"=0, "Voltage Control"=FALSE}, {"Drive"=enum."Idle", "Direction"=FALSE, "Phase Step"=enum."Duration", "Duration [s]"=0.0, "Current High [A]"=0.0, "Current Low [A]"=0.0, "Voltage High [V]"=0.0, "Voltage Low [V]"=0.0, "Change"=FALSE, "Current Control"=enum."Closed Loop", "Period [s]"=0.0, "Pulse Width [s]"=0.0, "Profile"=0, "Voltage Control"=FALSE}, {"Drive"=enum."Idle", "Direction"=FALSE, "Phase Step"=enum."Duration", "Duration [s]"=0.0, "Current High [A]"=0.0, "Current Low [A]"=0.0, "Voltage High [V]"=0.0, "Voltage Low [V]"=0.0, "Change"=FALSE, "Current Control"=enum."Closed Loop", "Period [s]"=0.0, "Pulse Width [s]"=0.0, "Profile"=0, "Voltage Control"=FALSE}, {"Drive"=enum."Idle", "Direction"=FALSE, "Phase Step"=enum."Duration", "Duration [s]"=0.0, "Current High [A]"=0.0, "Current Low [A]"=0.0, "Voltage High [V]"=0.0, "Voltage Low [V]"=0.0, "Change"=FALSE, "Current Control"=enum."Closed Loop", "Period [s]"=0.0, "Pulse Width [s]"=0.0, "Profile"=0, "Voltage Control"=FALSE}, {"Drive"=enum."Idle", "Direction"=FALSE, "Phase Step"=enum."Duration", "Duration [s]"=0.0, "Current High [A]"=0.0, "Current Low [A]"=0.0, "Voltage High [V]"=0.0, "Voltage Low [V]"=0.0, "Change"=FALSE, "Current Control"=enum."Closed Loop", "Period [s]"=0.0, "Pulse Width [s]"=0.0, "Profile"=0, "Voltage Control"=FALSE}, {"Drive"=enum."Idle", "Direction"=FALSE, "Phase Step"=enum."Duration", "Duration [s]"=0.0, "Current High [A]"=0.0, "Current Low [A]"=0.0, "Voltage High [V]"=0.0, "Voltage Low [V]"=0.0, "Change"=FALSE, "Current Control"=enum."Closed Loop", "Period [s]"=0.0, "Pulse Width [s]"=0.0, "Profile"=0, "Voltage Control"=FALSE}, {"Drive"=enum."Idle", "Direction"=FALSE, "Phase Step"=enum."Duration", "Duration [s]"=0.0, "Current High [A]"=0.0, "Current Low [A]"=0.0, "Voltage High [V]"=0.0, "Voltage Low [V]"=0.0, "Change"=FALSE, "Current Control"=enum."Closed Loop", "Period [s]"=0.0, "Pulse Width [s]"=0.0, "Profile"=0, "Voltage Control"=FALSE}, {"Drive"=enum."Idle", "Direction"=FALSE, "Phase Step"=enum."Duration", "Duration [s]"=0.0, "Current High [A]"=0.0, "Current Low [A]"=0.0, "Voltage High [V]"=0.0, "Voltage Low [V]"=0.0, "Change"=FALSE, "Current Control"=enum."Closed Loop", "Period [s]"=0.0, "Pulse Width [s]"=0.0, "Profile"=0, "Voltage Control"=FALSE}, {"Drive"=enum."Idle", "Direction"=FALSE, "Phase Step"=enum."Duration", "Duration [s]"=0.0, "Current High [A]"=0.0, "Current Low [A]"=0.0, "Voltage High [V]"=0.0, "Voltage Low [V]"=0.0, "Change"=FALSE, "Current Control"=enum."Closed Loop", "Period [s]"=0.0, "Pulse Width [s]"=0.0, "Profile"=0, "Voltage Control"=FALSE}, {"Drive"=enum."Idle", "Direction"=FALSE, "Phase Step"=enum."Duration", "Duration [s]"=0.0, "Current High [A]"=0.0, "Current Low [A]"=0.0, "Voltage High [V]"=0.0, "Voltage Low [V]"=0.0, "Change"=FALSE, "Current Control"=enum."Closed Loop", "Period [s]"=0.0, "Pulse Width [s]"=0.0, "Profile"=0, "Voltage Control"=FALSE}, {"Drive"=enum."Idle", "Direction"=FALSE, "Phase Step"=enum."Duration", "Duration [s]"=0.0, "Current High [A]"=0.0, "Current Low [A]"=0.0, "Voltage High [V]"=0.0, "Voltage Low [V]"=0.0, "Change"=FALSE, "Current Control"=enum."Closed Loop", "Period [s]"=0.0, "Pulse Width [s]"=0.0, "Profile"=0, "Voltage Control"=FALSE}, {"Drive"=enum."Idle", "Direction"=FALSE, "Phase Step"=enum."Duration", "Duration [s]"=0.0, "Current High [A]"=0.0, "Current Low [A]"=0.0, "Voltage High [V]"=0.0, "Voltage Low [V]"=0.0, "Change"=FALSE, "Current Control"=enum."Closed Loop", "Period [s]"=0.0, "Pulse Width [s]"=0.0, "Profile"=0, "Voltage Control"=FALSE}, {"Drive"=enum."Idle", "Direction"=FALSE, "Phase Step"=enum."Duration", "Duration [s]"=0.0, "Current High [A]"=0.0, "Current Low [A]"=0.0, "Voltage High [V]"=0.0, "Voltage Low [V]"=0.0, "Change"=FALSE, "Current Control"=enum."Closed Loop", "Period [s]"=0.0, "Pulse Width [s]"=0.0, "Profile"=0, "Voltage Control"=FALSE}, {"Drive"=enum."Idle", "Direction"=FALSE, "Phase Step"=enum."Duration", "Duration [s]"=0.0, "Current High [A]"=0.0, "Current Low [A]"=0.0, "Voltage High [V]"=0.0, "Voltage Low [V]"=0.0, "Change"=FALSE, "Current Control"=enum."Closed Loop", "Period [s]"=0.0, "Pulse Width [s]"=0.0, "Profile"=0, "Voltage Control"=FALSE}, {"Drive"=enum."Idle", "Direction"=FALSE, "Phase Step"=enum."Duration", "Duration [s]"=0.0, "Current High [A]"=0.0, "Current Low [A]"=0.0, "Voltage High [V]"=0.0, "Voltage Low [V]"=0.0, "Change"=FALSE, "Current Control"=enum."Closed Loop", "Period [s]"=0.0, "Pulse Width [s]"=0.0, "Profile"=0, "Voltage Control"=FALSE}, {"Drive"=enum."Idle", "Direction"=FALSE, "Phase Step"=enum."Duration", "Duration [s]"=0.0, "Current High [A]"=0.0, "Current Low [A]"=0.0, "Voltage High [V]"=0.0, "Voltage Low [V]"=0.0, "Change"=FALSE, "Current Control"=enum."Closed Loop", "Period [s]"=0.0, "Pulse Width [s]"=0.0, "Profile"=0, "Voltage Control"=FALSE}], [{"Drive"=enum."Idle", "Direction"=FALSE, "Phase Step"=enum."Duration", "Duration [s]"=0.0, "Current High [A]"=0.0, "Current Low [A]"=0.0, "Voltage High [V]"=0.0, "Voltage Low [V]"=0.0, "Change"=FALSE, "Current Control"=enum."Closed Loop", "Period [s]"=0.0, "Pulse Width [s]"=0.0, "Profile"=0, "Voltage Control"=FALSE}, {"Drive"=enum."Idle", "Direction"=FALSE, "Phase Step"=enum."Duration", "Duration [s]"=0.0, "Current High [A]"=0.0, "Current Low [A]"=0.0, "Voltage High [V]"=0.0, "Voltage Low [V]"=0.0, "Change"=FALSE, "Current Control"=enum."Closed Loop", "Period [s]"=0.0, "Pulse Width [s]"=0.0, "Profile"=0, "Voltage Control"=FALSE}, {"Drive"=enum."Idle", "Direction"=FALSE, "Phase Step"=enum."Duration", "Duration [s]"=0.0, "Current High [A]"=0.0, "Current Low [A]"=0.0, "Voltage High [V]"=0.0, "Voltage Low [V]"=0.0, "Change"=FALSE, "Current Control"=enum."Closed Loop", "Period [s]"=0.0, "Pulse Width [s]"=0.0, "Profile"=0, "Voltage Control"=FALSE}, {"Drive"=enum."Idle", "Direction"=FALSE, "Phase Step"=enum."Duration", "Duration [s]"=0.0, "Current High [A]"=0.0, "Current Low [A]"=0.0, "Voltage High [V]"=0.0, "Voltage Low [V]"=0.0, "Change"=FALSE, "Current Control"=enum."Closed Loop", "Period [s]"=0.0, "Pulse Width [s]"=0.0, "Profile"=0, "Voltage Control"=FALSE}, {"Drive"=enum."Idle", "Direction"=FALSE, "Phase Step"=enum."Duration", "Duration [s]"=0.0, "Current High [A]"=0.0, "Current Low [A]"=0.0, "Voltage High [V]"=0.0, "Voltage Low [V]"=0.0, "Change"=FALSE, "Current Control"=enum."Closed Loop", "Period [s]"=0.0, "Pulse Width [s]"=0.0, "Profile"=0, "Voltage Control"=FALSE}, {"Drive"=enum."Idle", "Direction"=FALSE, "Phase Step"=enum."Duration", "Duration [s]"=0.0, "Current High [A]"=0.0, "Current Low [A]"=0.0, "Voltage High [V]"=0.0, "Voltage Low [V]"=0.0, "Change"=FALSE, "Current Control"=enum."Closed Loop", "Period [s]"=0.0, "Pulse Width [s]"=0.0, "Profile"=0, "Voltage Control"=FALSE}, {"Drive"=enum."Idle", "Direction"=FALSE, "Phase Step"=enum."Duration", "Duration [s]"=0.0, "Current High [A]"=0.0, "Current Low [A]"=0.0, "Voltage High [V]"=0.0, "Voltage Low [V]"=0.0, "Change"=FALSE, "Current Control"=enum."Closed Loop", "Period [s]"=0.0, "Pulse Width [s]"=0.0, "Profile"=0, "Voltage Control"=FALSE}, {"Drive"=enum."Idle", "Direction"=FALSE, "Phase Step"=enum."Duration", "Duration [s]"=0.0, "Current High [A]"=0.0, "Current Low [A]"=0.0, "Voltage High [V]"=0.0, "Voltage Low [V]"=0.0, "Change"=FALSE, "Current Control"=enum."Closed Loop", "Period [s]"=0.0, "Pulse Width [s]"=0.0, "Profile"=0, "Voltage Control"=FALSE}, {"Drive"=enum."Idle", "Direction"=FALSE, "Phase Step"=enum."Duration", "Duration [s]"=0.0, "Current High [A]"=0.0, "Current Low [A]"=0.0, "Voltage High [V]"=0.0, "Voltage Low [V]"=0.0, "Change"=FALSE, "Current Control"=enum."Closed Loop", "Period [s]"=0.0, "Pulse Width [s]"=0.0, "Profile"=0, "Voltage Control"=FALSE}, {"Drive"=enum."Idle", "Direction"=FALSE, "Phase Step"=enum."Duration", "Duration [s]"=0.0, "Current High [A]"=0.0, "Current Low [A]"=0.0, "Voltage High [V]"=0.0, "Voltage Low [V]"=0.0, "Change"=FALSE, "Current Control"=enum."Closed Loop", "Period [s]"=0.0, "Pulse Width [s]"=0.0, "Profile"=0, "Voltage Control"=FALSE}, {"Drive"=enum."Idle", "Direction"=FALSE, "Phase Step"=enum."Duration", "Duration [s]"=0.0, "Current High [A]"=0.0, "Current Low [A]"=0.0, "Voltage High [V]"=0.0, "Voltage Low [V]"=0.0, "Change"=FALSE, "Current Control"=enum."Closed Loop", "Period [s]"=0.0, "Pulse Width [s]"=0.0, "Profile"=0, "Voltage Control"=FALSE}, {"Drive"=enum."Idle", "Direction"=FALSE, "Phase Step"=enum."Duration", "Duration [s]"=0.0, "Current High [A]"=0.0, "Current Low [A]"=0.0, "Voltage High [V]"=0.0, "Voltage Low [V]"=0.0, "Change"=FALSE, "Current Control"=enum."Closed Loop", "Period [s]"=0.0, "Pulse Width [s]"=0.0, "Profile"=0, "Voltage Control"=FALSE}, {"Drive"=enum."Idle", "Direction"=FALSE, "Phase Step"=enum."Duration", "Duration [s]"=0.0, "Current High [A]"=0.0, "Current Low [A]"=0.0, "Voltage High [V]"=0.0, "Voltage Low [V]"=0.0, "Change"=FALSE, "Current Control"=enum."Closed Loop", "Period [s]"=0.0, "Pulse Width [s]"=0.0, "Profile"=0, "Voltage Control"=FALSE}, {"Drive"=enum."Idle", "Direction"=FALSE, "Phase Step"=enum."Duration", "Duration [s]"=0.0, "Current High [A]"=0.0, "Current Low [A]"=0.0, "Voltage High [V]"=0.0, "Voltage Low [V]"=0.0, "Change"=FALSE, "Current Control"=enum."Closed Loop", "Period [s]"=0.0, "Pulse Width [s]"=0.0, "Profile"=0, "Voltage Control"=FALSE}, {"Drive"=enum."Idle", "Direction"=FALSE, "Phase Step"=enum."Duration", "Duration [s]"=0.0, "Current High [A]"=0.0, "Current Low [A]"=0.0, "Voltage High [V]"=0.0, "Voltage Low [V]"=0.0, "Change"=FALSE, "Current Control"=enum."Closed Loop", "Period [s]"=0.0, "Pulse Width [s]"=0.0, "Profile"=0, "Voltage Control"=FALSE}, {"Drive"=enum."Idle", "Direction"=FALSE, "Phase Step"=enum."Duration", "Duration [s]"=0.0, "Current High [A]"=0.0, "Current Low [A]"=0.0, "Voltage High [V]"=0.0, "Voltage Low [V]"=0.0, "Change"=FALSE, "Current Control"=enum."Closed Loop", "Period [s]"=0.0, "Pulse Width [s]"=0.0, "Profile"=0, "Voltage Control"=FALSE}], [{"Drive"=enum."Idle", "Direction"=FALSE, "Phase Step"=enum."Duration", "Duration [s]"=0.0, "Current High [A]"=0.0, "Current Low [A]"=0.0, "Voltage High [V]"=0.0, "Voltage Low [V]"=0.0, "Change"=FALSE, "Current Control"=enum."Closed Loop", "Period [s]"=0.0, "Pulse Width [s]"=0.0, "Profile"=0, "Voltage Control"=FALSE}, {"Drive"=enum."Idle", "Direction"=FALSE, "Phase Step"=enum."Duration", "Duration [s]"=0.0, "Current High [A]"=0.0, "Current Low [A]"=0.0, "Voltage High [V]"=0.0, "Voltage Low [V]"=0.0, "Change"=FALSE, "Current Control"=enum."Closed Loop", "Period [s]"=0.0, "Pulse Width [s]"=0.0, "Profile"=0, "Voltage Control"=FALSE}, {"Drive"=enum."Idle", "Direction"=FALSE, "Phase Step"=enum."Duration", "Duration [s]"=0.0, "Current High [A]"=0.0, "Current Low [A]"=0.0, "Voltage High [V]"=0.0, "Voltage Low [V]"=0.0, "Change"=FALSE, "Current Control"=enum."Closed Loop", "Period [s]"=0.0, "Pulse Width [s]"=0.0, "Profile"=0, "Voltage Control"=FALSE}, {"Drive"=enum."Idle", "Direction"=FALSE, "Phase Step"=enum."Duration", "Duration [s]"=0.0, "Current High [A]"=0.0, "Current Low [A]"=0.0, "Voltage High [V]"=0.0, "Voltage Low [V]"=0.0, "Change"=FALSE, "Current Control"=enum."Closed Loop", "Period [s]"=0.0, "Pulse Width [s]"=0.0, "Profile"=0, "Voltage Control"=FALSE}, {"Drive"=enum."Idle", "Direction"=FALSE, "Phase Step"=enum."Duration", "Duration [s]"=0.0, "Current High [A]"=0.0, "Current Low [A]"=0.0, "Voltage High [V]"=0.0, "Voltage Low [V]"=0.0, "Change"=FALSE, "Current Control"=enum."Closed Loop", "Period [s]"=0.0, "Pulse Width [s]"=0.0, "Profile"=0, "Voltage Control"=FALSE}, {"Drive"=enum."Idle", "Direction"=FALSE, "Phase Step"=enum."Duration", "Duration [s]"=0.0, "Current High [A]"=0.0, "Current Low [A]"=0.0, "Voltage High [V]"=0.0, "Voltage Low [V]"=0.0, "Change"=FALSE, "Current Control"=enum."Closed Loop", "Period [s]"=0.0, "Pulse Width [s]"=0.0, "Profile"=0, "Voltage Control"=FALSE}, {"Drive"=enum."Idle", "Direction"=FALSE, "Phase Step"=enum."Duration", "Duration [s]"=0.0, "Current High [A]"=0.0, "Current Low [A]"=0.0, "Voltage High [V]"=0.0, "Voltage Low [V]"=0.0, "Change"=FALSE, "Current Control"=enum."Closed Loop", "Period [s]"=0.0, "Pulse Width [s]"=0.0, "Profile"=0, "Voltage Control"=FALSE}, {"Drive"=enum."Idle", "Direction"=FALSE, "Phase Step"=enum."Duration", "Duration [s]"=0.0, "Current High [A]"=0.0, "Current Low [A]"=0.0, "Voltage High [V]"=0.0, "Voltage Low [V]"=0.0, "Change"=FALSE, "Current Control"=enum."Closed Loop", "Period [s]"=0.0, "Pulse Width [s]"=0.0, "Profile"=0, "Voltage Control"=FALSE}, {"Drive"=enum."Idle", "Direction"=FALSE, "Phase Step"=enum."Duration", "Duration [s]"=0.0, "Current High [A]"=0.0, "Current Low [A]"=0.0, "Voltage High [V]"=0.0, "Voltage Low [V]"=0.0, "Change"=FALSE, "Current Control"=enum."Closed Loop", "Period [s]"=0.0, "Pulse Width [s]"=0.0, "Profile"=0, "Voltage Control"=FALSE}, {"Drive"=enum."Idle", "Direction"=FALSE, "Phase Step"=enum."Duration", "Duration [s]"=0.0, "Current High [A]"=0.0, "Current Low [A]"=0.0, "Voltage High [V]"=0.0, "Voltage Low [V]"=0.0, "Change"=FALSE, "Current Control"=enum."Closed Loop", "Period [s]"=0.0, "Pulse Width [s]"=0.0, "Profile"=0, "Voltage Control"=FALSE}, {"Drive"=enum."Idle", "Direction"=FALSE, "Phase Step"=enum."Duration", "Duration [s]"=0.0, "Current High [A]"=0.0, "Current Low [A]"=0.0, "Voltage High [V]"=0.0, "Voltage Low [V]"=0.0, "Change"=FALSE, "Current Control"=enum."Closed Loop", "Period [s]"=0.0, "Pulse Width [s]"=0.0, "Profile"=0, "Voltage Control"=FALSE}, {"Drive"=enum."Idle", "Direction"=FALSE, "Phase Step"=enum."Duration", "Duration [s]"=0.0, "Current High [A]"=0.0, "Current Low [A]"=0.0, "Voltage High [V]"=0.0, "Voltage Low [V]"=0.0, "Change"=FALSE, "Current Control"=enum."Closed Loop", "Period [s]"=0.0, "Pulse Width [s]"=0.0, "Profile"=0, "Voltage Control"=FALSE}, {"Drive"=enum."Idle", "Direction"=FALSE, "Phase Step"=enum."Duration", "Duration [s]"=0.0, "Current High [A]"=0.0, "Current Low [A]"=0.0, "Voltage High [V]"=0.0, "Voltage Low [V]"=0.0, "Change"=FALSE, "Current Control"=enum."Closed Loop", "Period [s]"=0.0, "Pulse Width [s]"=0.0, "Profile"=0, "Voltage Control"=FALSE}, {"Drive"=enum."Idle", "Direction"=FALSE, "Phase Step"=enum."Duration", "Duration [s]"=0.0, "Current High [A]"=0.0, "Current Low [A]"=0.0, "Voltage High [V]"=0.0, "Voltage Low [V]"=0.0, "Change"=FALSE, "Current Control"=enum."Closed Loop", "Period [s]"=0.0, "Pulse Width [s]"=0.0, "Profile"=0, "Voltage Control"=FALSE}, {"Drive"=enum."Idle", "Direction"=FALSE, "Phase Step"=enum."Duration", "Duration [s]"=0.0, "Current High [A]"=0.0, "Current Low [A]"=0.0, "Voltage High [V]"=0.0, "Voltage Low [V]"=0.0, "Change"=FALSE, "Current Control"=enum."Closed Loop", "Period [s]"=0.0, "Pulse Width [s]"=0.0, "Profile"=0, "Voltage Control"=FALSE}, {"Drive"=enum."Idle", "Direction"=FALSE, "Phase Step"=enum."Duration", "Duration [s]"=0.0, "Current High [A]"=0.0, "Current Low [A]"=0.0, "Voltage High [V]"=0.0, "Voltage Low [V]"=0.0, "Change"=FALSE, "Current Control"=enum."Closed Loop", "Period [s]"=0.0, "Pulse Width [s]"=0.0, "Profile"=0, "Voltage Control"=FALSE}], [{"Drive"=enum."Idle", "Direction"=FALSE, "Phase Step"=enum."Duration", "Duration [s]"=0.0, "Current High [A]"=0.0, "Current Low [A]"=0.0, "Voltage High [V]"=0.0, "Voltage Low [V]"=0.0, "Change"=FALSE, "Current Control"=enum."Closed Loop", "Period [s]"=0.0, "Pulse Width [s]"=0.0, "Profile"=0, "Voltage Control"=FALSE}, {"Drive"=enum."Idle", "Direction"=FALSE, "Phase Step"=enum."Duration", "Duration [s]"=0.0, "Current High [A]"=0.0, "Current Low [A]"=0.0, "Voltage High [V]"=0.0, "Voltage Low [V]"=0.0, "Change"=FALSE, "Current Control"=enum."Closed Loop", "Period [s]"=0.0, "Pulse Width [s]"=0.0, "Profile"=0, "Voltage Control"=FALSE}, {"Drive"=enum."Idle", "Direction"=FALSE, "Phase Step"=enum."Duration", "Duration [s]"=0.0, "Current High [A]"=0.0, "Current Low [A]"=0.0, "Voltage High [V]"=0.0, "Voltage Low [V]"=0.0, "Change"=FALSE, "Current Control"=enum."Closed Loop", "Period [s]"=0.0, "Pulse Width [s]"=0.0, "Profile"=0, "Voltage Control"=FALSE}, {"Drive"=enum."Idle", "Direction"=FALSE, "Phase Step"=enum."Duration", "Duration [s]"=0.0, "Current High [A]"=0.0, "Current Low [A]"=0.0, "Voltage High [V]"=0.0, "Voltage Low [V]"=0.0, "Change"=FALSE, "Current Control"=enum."Closed Loop", "Period [s]"=0.0, "Pulse Width [s]"=0.0, "Profile"=0, "Voltage Control"=FALSE}, {"Drive"=enum."Idle", "Direction"=FALSE, "Phase Step"=enum."Duration", "Duration [s]"=0.0, "Current High [A]"=0.0, "Current Low [A]"=0.0, "Voltage High [V]"=0.0, "Voltage Low [V]"=0.0, "Change"=FALSE, "Current Control"=enum."Closed Loop", "Period [s]"=0.0, "Pulse Width [s]"=0.0, "Profile"=0, "Voltage Control"=FALSE}, {"Drive"=enum."Idle", "Direction"=FALSE, "Phase Step"=enum."Duration", "Duration [s]"=0.0, "Current High [A]"=0.0, "Current Low [A]"=0.0, "Voltage High [V]"=0.0, "Voltage Low [V]"=0.0, "Change"=FALSE, "Current Control"=enum."Closed Loop", "Period [s]"=0.0, "Pulse Width [s]"=0.0, "Profile"=0, "Voltage Control"=FALSE}, {"Drive"=enum."Idle", "Direction"=FALSE, "Phase Step"=enum."Duration", "Duration [s]"=0.0, "Current High [A]"=0.0, "Current Low [A]"=0.0, "Voltage High [V]"=0.0, "Voltage Low [V]"=0.0, "Change"=FALSE, "Current Control"=enum."Closed Loop", "Period [s]"=0.0, "Pulse Width [s]"=0.0, "Profile"=0, "Voltage Control"=FALSE}, {"Drive"=enum."Idle", "Direction"=FALSE, "Phase Step"=enum."Duration", "Duration [s]"=0.0, "Current High [A]"=0.0, "Current Low [A]"=0.0, "Voltage High [V]"=0.0, "Voltage Low [V]"=0.0, "Change"=FALSE, "Current Control"=enum."Closed Loop", "Period [s]"=0.0, "Pulse Width [s]"=0.0, "Profile"=0, "Voltage Control"=FALSE}, {"Drive"=enum."Idle", "Direction"=FALSE, "Phase Step"=enum."Duration", "Duration [s]"=0.0, "Current High [A]"=0.0, "Current Low [A]"=0.0, "Voltage High [V]"=0.0, "Voltage Low [V]"=0.0, "Change"=FALSE, "Current Control"=enum."Closed Loop", "Period [s]"=0.0, "Pulse Width [s]"=0.0, "Profile"=0, "Voltage Control"=FALSE}, {"Drive"=enum."Idle", "Direction"=FALSE, "Phase Step"=enum."Duration", "Duration [s]"=0.0, "Current High [A]"=0.0, "Current Low [A]"=0.0, "Voltage High [V]"=0.0, "Voltage Low [V]"=0.0, "Change"=FALSE, "Current Control"=enum."Closed Loop", "Period [s]"=0.0, "Pulse Width [s]"=0.0, "Profile"=0, "Voltage Control"=FALSE}, {"Drive"=enum."Idle", "Direction"=FALSE, "Phase Step"=enum."Duration", "Duration [s]"=0.0, "Current High [A]"=0.0, "Current Low [A]"=0.0, "Voltage High [V]"=0.0, "Voltage Low [V]"=0.0, "Change"=FALSE, "Current Control"=enum."Closed Loop", "Period [s]"=0.0, "Pulse Width [s]"=0.0, "Profile"=0, "Voltage Control"=FALSE}, {"Drive"=enum."Idle", "Direction"=FALSE, "Phase Step"=enum."Duration", "Duration [s]"=0.0, "Current High [A]"=0.0, "Current Low [A]"=0.0, "Voltage High [V]"=0.0, "Voltage Low [V]"=0.0, "Change"=FALSE, "Current Control"=enum."Closed Loop", "Period [s]"=0.0, "Pulse Width [s]"=0.0, "Profile"=0, "Voltage Control"=FALSE}, {"Drive"=enum."Idle", "Direction"=FALSE, "Phase Step"=enum."Duration", "Duration [s]"=0.0, "Current High [A]"=0.0, "Current Low [A]"=0.0, "Voltage High [V]"=0.0, "Voltage Low [V]"=0.0, "Change"=FALSE, "Current Control"=enum."Closed Loop", "Period [s]"=0.0, "Pulse Width [s]"=0.0, "Profile"=0, "Voltage Control"=FALSE}, {"Drive"=enum."Idle", "Direction"=FALSE, "Phase Step"=enum."Duration", "Duration [s]"=0.0, "Current High [A]"=0.0, "Current Low [A]"=0.0, "Voltage High [V]"=0.0, "Voltage Low [V]"=0.0, "Change"=FALSE, "Current Control"=enum."Closed Loop", "Period [s]"=0.0, "Pulse Width [s]"=0.0, "Profile"=0, "Voltage Control"=FALSE}, {"Drive"=enum."Idle", "Direction"=FALSE, "Phase Step"=enum."Duration", "Duration [s]"=0.0, "Current High [A]"=0.0, "Current Low [A]"=0.0, "Voltage High [V]"=0.0, "Voltage Low [V]"=0.0, "Change"=FALSE, "Current Control"=enum."Closed Loop", "Period [s]"=0.0, "Pulse Width [s]"=0.0, "Profile"=0, "Voltage Control"=FALSE}, {"Drive"=enum."Idle", "Direction"=FALSE, "Phase Step"=enum."Duration", "Duration [s]"=0.0, "Current High [A]"=0.0, "Current Low [A]"=0.0, "Voltage High [V]"=0.0, "Voltage Low [V]"=0.0, "Change"=FALSE, "Current Control"=enum."Closed Loop", "Period [s]"=0.0, "Pulse Width [s]"=0.0, "Profile"=0, "Voltage Control"=FALSE}], [{"Drive"=enum."Idle", "Direction"=FALSE, "Phase Step"=enum."Duration", "Duration [s]"=0.0, "Current High [A]"=0.0, "Current Low [A]"=0.0, "Voltage High [V]"=0.0, "Voltage Low [V]"=0.0, "Change"=FALSE, "Current Control"=enum."Closed Loop", "Period [s]"=0.0, "Pulse Width [s]"=0.0, "Profile"=0, "Voltage Control"=FALSE}, {"Drive"=enum."Idle", "Direction"=FALSE, "Phase Step"=enum."Duration", "Duration [s]"=0.0, "Current High [A]"=0.0, "Current Low [A]"=0.0, "Voltage High [V]"=0.0, "Voltage Low [V]"=0.0, "Change"=FALSE, "Current Control"=enum."Closed Loop", "Period [s]"=0.0, "Pulse Width [s]"=0.0, "Profile"=0, "Voltage Control"=FALSE}, {"Drive"=enum."Idle", "Direction"=FALSE, "Phase Step"=enum."Duration", "Duration [s]"=0.0, "Current High [A]"=0.0, "Current Low [A]"=0.0, "Voltage High [V]"=0.0, "Voltage Low [V]"=0.0, "Change"=FALSE, "Current Control"=enum."Closed Loop", "Period [s]"=0.0, "Pulse Width [s]"=0.0, "Profile"=0, "Voltage Control"=FALSE}, {"Drive"=enum."Idle", "Direction"=FALSE, "Phase Step"=enum."Duration", "Duration [s]"=0.0, "Current High [A]"=0.0, "Current Low [A]"=0.0, "Voltage High [V]"=0.0, "Voltage Low [V]"=0.0, "Change"=FALSE, "Current Control"=enum."Closed Loop", "Period [s]"=0.0, "Pulse Width [s]"=0.0, "Profile"=0, "Voltage Control"=FALSE}, {"Drive"=enum."Idle", "Direction"=FALSE, "Phase Step"=enum."Duration", "Duration [s]"=0.0, "Current High [A]"=0.0, "Current Low [A]"=0.0, "Voltage High [V]"=0.0, "Voltage Low [V]"=0.0, "Change"=FALSE, "Current Control"=enum."Closed Loop", "Period [s]"=0.0, "Pulse Width [s]"=0.0, "Profile"=0, "Voltage Control"=FALSE}, {"Drive"=enum."Idle", "Direction"=FALSE, "Phase Step"=enum."Duration", "Duration [s]"=0.0, "Current High [A]"=0.0, "Current Low [A]"=0.0, "Voltage High [V]"=0.0, "Voltage Low [V]"=0.0, "Change"=FALSE, "Current Control"=enum."Closed Loop", "Period [s]"=0.0, "Pulse Width [s]"=0.0, "Profile"=0, "Voltage Control"=FALSE}, {"Drive"=enum."Idle", "Direction"=FALSE, "Phase Step"=enum."Duration", "Duration [s]"=0.0, "Current High [A]"=0.0, "Current Low [A]"=0.0, "Voltage High [V]"=0.0, "Voltage Low [V]"=0.0, "Change"=FALSE, "Current Control"=enum."Closed Loop", "Period [s]"=0.0, "Pulse Width [s]"=0.0, "Profile"=0, "Voltage Control"=FALSE}, {"Drive"=enum."Idle", "Direction"=FALSE, "Phase Step"=enum."Duration", "Duration [s]"=0.0, "Current High [A]"=0.0, "Current Low [A]"=0.0, "Voltage High [V]"=0.0, "Voltage Low [V]"=0.0, "Change"=FALSE, "Current Control"=enum."Closed Loop", "Period [s]"=0.0, "Pulse Width [s]"=0.0, "Profile"=0, "Voltage Control"=FALSE}, {"Drive"=enum."Idle", "Direction"=FALSE, "Phase Step"=enum."Duration", "Duration [s]"=0.0, "Current High [A]"=0.0, "Current Low [A]"=0.0, "Voltage High [V]"=0.0, "Voltage Low [V]"=0.0, "Change"=FALSE, "Current Control"=enum."Closed Loop", "Period [s]"=0.0, "Pulse Width [s]"=0.0, "Profile"=0, "Voltage Control"=FALSE}, {"Drive"=enum."Idle", "Direction"=FALSE, "Phase Step"=enum."Duration", "Duration [s]"=0.0, "Current High [A]"=0.0, "Current Low [A]"=0.0, "Voltage High [V]"=0.0, "Voltage Low [V]"=0.0, "Change"=FALSE, "Current Control"=enum."Closed Loop", "Period [s]"=0.0, "Pulse Width [s]"=0.0, "Profile"=0, "Voltage Control"=FALSE}, {"Drive"=enum."Idle", "Direction"=FALSE, "Phase Step"=enum."Duration", "Duration [s]"=0.0, "Current High [A]"=0.0, "Current Low [A]"=0.0, "Voltage High [V]"=0.0, "Voltage Low [V]"=0.0, "Change"=FALSE, "Current Control"=enum."Closed Loop", "Period [s]"=0.0, "Pulse Width [s]"=0.0, "Profile"=0, "Voltage Control"=FALSE}, {"Drive"=enum."Idle", "Direction"=FALSE, "Phase Step"=enum."Duration", "Duration [s]"=0.0, "Current High [A]"=0.0, "Current Low [A]"=0.0, "Voltage High [V]"=0.0, "Voltage Low [V]"=0.0, "Change"=FALSE, "Current Control"=enum."Closed Loop", "Period [s]"=0.0, "Pulse Width [s]"=0.0, "Profile"=0, "Voltage Control"=FALSE}, {"Drive"=enum."Idle", "Direction"=FALSE, "Phase Step"=enum."Duration", "Duration [s]"=0.0, "Current High [A]"=0.0, "Current Low [A]"=0.0, "Voltage High [V]"=0.0, "Voltage Low [V]"=0.0, "Change"=FALSE, "Current Control"=enum."Closed Loop", "Period [s]"=0.0, "Pulse Width [s]"=0.0, "Profile"=0, "Voltage Control"=FALSE}, {"Drive"=enum."Idle", "Direction"=FALSE, "Phase Step"=enum."Duration", "Duration [s]"=0.0, "Current High [A]"=0.0, "Current Low [A]"=0.0, "Voltage High [V]"=0.0, "Voltage Low [V]"=0.0, "Change"=FALSE, "Current Control"=enum."Closed Loop", "Period [s]"=0.0, "Pulse Width [s]"=0.0, "Profile"=0, "Voltage Control"=FALSE}, {"Drive"=enum."Idle", "Direction"=FALSE, "Phase Step"=enum."Duration", "Duration [s]"=0.0, "Current High [A]"=0.0, "Current Low [A]"=0.0, "Voltage High [V]"=0.0, "Voltage Low [V]"=0.0, "Change"=FALSE, "Current Control"=enum."Closed Loop", "Period [s]"=0.0, "Pulse Width [s]"=0.0, "Profile"=0, "Voltage Control"=FALSE}, {"Drive"=enum."Idle", "Direction"=FALSE, "Phase Step"=enum."Duration", "Duration [s]"=0.0, "Current High [A]"=0.0, "Current Low [A]"=0.0, "Voltage High [V]"=0.0, "Voltage Low [V]"=0.0, "Change"=FALSE, "Current Control"=enum."Closed Loop", "Period [s]"=0.0, "Pulse Width [s]"=0.0, "Profile"=0, "Voltage Control"=FALSE}], [{"Drive"=enum."Idle", "Direction"=FALSE, "Phase Step"=enum."Duration", "Duration [s]"=0.0, "Current High [A]"=0.0, "Current Low [A]"=0.0, "Voltage High [V]"=0.0, "Voltage Low [V]"=0.0, "Change"=FALSE, "Current Control"=enum."Closed Loop", "Period [s]"=0.0, "Pulse Width [s]"=0.0, "Profile"=0, "Voltage Control"=FALSE}, {"Drive"=enum."Idle", "Direction"=FALSE, "Phase Step"=enum."Duration", "Duration [s]"=0.0, "Current High [A]"=0.0, "Current Low [A]"=0.0, "Voltage High [V]"=0.0, "Voltage Low [V]"=0.0, "Change"=FALSE, "Current Control"=enum."Closed Loop", "Period [s]"=0.0, "Pulse Width [s]"=0.0, "Profile"=0, "Voltage Control"=FALSE}, {"Drive"=enum."Idle", "Direction"=FALSE, "Phase Step"=enum."Duration", "Duration [s]"=0.0, "Current High [A]"=0.0, "Current Low [A]"=0.0, "Voltage High [V]"=0.0, "Voltage Low [V]"=0.0, "Change"=FALSE, "Current Control"=enum."Closed Loop", "Period [s]"=0.0, "Pulse Width [s]"=0.0, "Profile"=0, "Voltage Control"=FALSE}, {"Drive"=enum."Idle", "Direction"=FALSE, "Phase Step"=enum."Duration", "Duration [s]"=0.0, "Current High [A]"=0.0, "Current Low [A]"=0.0, "Voltage High [V]"=0.0, "Voltage Low [V]"=0.0, "Change"=FALSE, "Current Control"=enum."Closed Loop", "Period [s]"=0.0, "Pulse Width [s]"=0.0, "Profile"=0, "Voltage Control"=FALSE}, {"Drive"=enum."Idle", "Direction"=FALSE, "Phase Step"=enum."Duration", "Duration [s]"=0.0, "Current High [A]"=0.0, "Current Low [A]"=0.0, "Voltage High [V]"=0.0, "Voltage Low [V]"=0.0, "Change"=FALSE, "Current Control"=enum."Closed Loop", "Period [s]"=0.0, "Pulse Width [s]"=0.0, "Profile"=0, "Voltage Control"=FALSE}, {"Drive"=enum."Idle", "Direction"=FALSE, "Phase Step"=enum."Duration", "Duration [s]"=0.0, "Current High [A]"=0.0, "Current Low [A]"=0.0, "Voltage High [V]"=0.0, "Voltage Low [V]"=0.0, "Change"=FALSE, "Current Control"=enum."Closed Loop", "Period [s]"=0.0, "Pulse Width [s]"=0.0, "Profile"=0, "Voltage Control"=FALSE}, {"Drive"=enum."Idle", "Direction"=FALSE, "Phase Step"=enum."Duration", "Duration [s]"=0.0, "Current High [A]"=0.0, "Current Low [A]"=0.0, "Voltage High [V]"=0.0, "Voltage Low [V]"=0.0, "Change"=FALSE, "Current Control"=enum."Closed Loop", "Period [s]"=0.0, "Pulse Width [s]"=0.0, "Profile"=0, "Voltage Control"=FALSE}, {"Drive"=enum."Idle", "Direction"=FALSE, "Phase Step"=enum."Duration", "Duration [s]"=0.0, "Current High [A]"=0.0, "Current Low [A]"=0.0, "Voltage High [V]"=0.0, "Voltage Low [V]"=0.0, "Change"=FALSE, "Current Control"=enum."Closed Loop", "Period [s]"=0.0, "Pulse Width [s]"=0.0, "Profile"=0, "Voltage Control"=FALSE}, {"Drive"=enum."Idle", "Direction"=FALSE, "Phase Step"=enum."Duration", "Duration [s]"=0.0, "Current High [A]"=0.0, "Current Low [A]"=0.0, "Voltage High [V]"=0.0, "Voltage Low [V]"=0.0, "Change"=FALSE, "Current Control"=enum."Closed Loop", "Period [s]"=0.0, "Pulse Width [s]"=0.0, "Profile"=0, "Voltage Control"=FALSE}, {"Drive"=enum."Idle", "Direction"=FALSE, "Phase Step"=enum."Duration", "Duration [s]"=0.0, "Current High [A]"=0.0, "Current Low [A]"=0.0, "Voltage High [V]"=0.0, "Voltage Low [V]"=0.0, "Change"=FALSE, "Current Control"=enum."Closed Loop", "Period [s]"=0.0, "Pulse Width [s]"=0.0, "Profile"=0, "Voltage Control"=FALSE}, {"Drive"=enum."Idle", "Direction"=FALSE, "Phase Step"=enum."Duration", "Duration [s]"=0.0, "Current High [A]"=0.0, "Current Low [A]"=0.0, "Voltage High [V]"=0.0, "Voltage Low [V]"=0.0, "Change"=FALSE, "Current Control"=enum."Closed Loop", "Period [s]"=0.0, "Pulse Width [s]"=0.0, "Profile"=0, "Voltage Control"=FALSE}, {"Drive"=enum."Idle", "Direction"=FALSE, "Phase Step"=enum."Duration", "Duration [s]"=0.0, "Current High [A]"=0.0, "Current Low [A]"=0.0, "Voltage High [V]"=0.0, "Voltage Low [V]"=0.0, "Change"=FALSE, "Current Control"=enum."Closed Loop", "Period [s]"=0.0, "Pulse Width [s]"=0.0, "Profile"=0, "Voltage Control"=FALSE}, {"Drive"=enum."Idle", "Direction"=FALSE, "Phase Step"=enum."Duration", "Duration [s]"=0.0, "Current High [A]"=0.0, "Current Low [A]"=0.0, "Voltage High [V]"=0.0, "Voltage Low [V]"=0.0, "Change"=FALSE, "Current Control"=enum."Closed Loop", "Period [s]"=0.0, "Pulse Width [s]"=0.0, "Profile"=0, "Voltage Control"=FALSE}, {"Drive"=enum."Idle", "Direction"=FALSE, "Phase Step"=enum."Duration", "Duration [s]"=0.0, "Current High [A]"=0.0, "Current Low [A]"=0.0, "Voltage High [V]"=0.0, "Voltage Low [V]"=0.0, "Change"=FALSE, "Current Control"=enum."Closed Loop", "Period [s]"=0.0, "Pulse Width [s]"=0.0, "Profile"=0, "Voltage Control"=FALSE}, {"Drive"=enum."Idle", "Direction"=FALSE, "Phase Step"=enum."Duration", "Duration [s]"=0.0, "Current High [A]"=0.0, "Current Low [A]"=0.0, "Voltage High [V]"=0.0, "Voltage Low [V]"=0.0, "Change"=FALSE, "Current Control"=enum."Closed Loop", "Period [s]"=0.0, "Pulse Width [s]"=0.0, "Profile"=0, "Voltage Control"=FALSE}, {"Drive"=enum."Idle", "Direction"=FALSE, "Phase Step"=enum."Duration", "Duration [s]"=0.0, "Current High [A]"=0.0, "Current Low [A]"=0.0, "Voltage High [V]"=0.0, "Voltage Low [V]"=0.0, "Change"=FALSE, "Current Control"=enum."Closed Loop", "Period [s]"=0.0, "Pulse Width [s]"=0.0, "Profile"=0, "Voltage Control"=FALSE}], [{"Drive"=enum."Idle", "Direction"=FALSE, "Phase Step"=enum."Duration", "Duration [s]"=0.0, "Current High [A]"=0.0, "Current Low [A]"=0.0, "Voltage High [V]"=0.0, "Voltage Low [V]"=0.0, "Change"=FALSE, "Current Control"=enum."Closed Loop", "Period [s]"=0.0, "Pulse Width [s]"=0.0, "Profile"=0, "Voltage Control"=FALSE}, {"Drive"=enum."Idle", "Direction"=FALSE, "Phase Step"=enum."Duration", "Duration [s]"=0.0, "Current High [A]"=0.0, "Current Low [A]"=0.0, "Voltage High [V]"=0.0, "Voltage Low [V]"=0.0, "Change"=FALSE, "Current Control"=enum."Closed Loop", "Period [s]"=0.0, "Pulse Width [s]"=0.0, "Profile"=0, "Voltage Control"=FALSE}, {"Drive"=enum."Idle", "Direction"=FALSE, "Phase Step"=enum."Duration", "Duration [s]"=0.0, "Current High [A]"=0.0, "Current Low [A]"=0.0, "Voltage High [V]"=0.0, "Voltage Low [V]"=0.0, "Change"=FALSE, "Current Control"=enum."Closed Loop", "Period [s]"=0.0, "Pulse Width [s]"=0.0, "Profile"=0, "Voltage Control"=FALSE}, {"Drive"=enum."Idle", "Direction"=FALSE, "Phase Step"=enum."Duration", "Duration [s]"=0.0, "Current High [A]"=0.0, "Current Low [A]"=0.0, "Voltage High [V]"=0.0, "Voltage Low [V]"=0.0, "Change"=FALSE, "Current Control"=enum."Closed Loop", "Period [s]"=0.0, "Pulse Width [s]"=0.0, "Profile"=0, "Voltage Control"=FALSE}, {"Drive"=enum."Idle", "Direction"=FALSE, "Phase Step"=enum."Duration", "Duration [s]"=0.0, "Current High [A]"=0.0, "Current Low [A]"=0.0, "Voltage High [V]"=0.0, "Voltage Low [V]"=0.0, "Change"=FALSE, "Current Control"=enum."Closed Loop", "Period [s]"=0.0, "Pulse Width [s]"=0.0, "Profile"=0, "Voltage Control"=FALSE}, {"Drive"=enum."Idle", "Direction"=FALSE, "Phase Step"=enum."Duration", "Duration [s]"=0.0, "Current High [A]"=0.0, "Current Low [A]"=0.0, "Voltage High [V]"=0.0, "Voltage Low [V]"=0.0, "Change"=FALSE, "Current Control"=enum."Closed Loop", "Period [s]"=0.0, "Pulse Width [s]"=0.0, "Profile"=0, "Voltage Control"=FALSE}, {"Drive"=enum."Idle", "Direction"=FALSE, "Phase Step"=enum."Duration", "Duration [s]"=0.0, "Current High [A]"=0.0, "Current Low [A]"=0.0, "Voltage High [V]"=0.0, "Voltage Low [V]"=0.0, "Change"=FALSE, "Current Control"=enum."Closed Loop", "Period [s]"=0.0, "Pulse Width [s]"=0.0, "Profile"=0, "Voltage Control"=FALSE}, {"Drive"=enum."Idle", "Direction"=FALSE, "Phase Step"=enum."Duration", "Duration [s]"=0.0, "Current High [A]"=0.0, "Current Low [A]"=0.0, "Voltage High [V]"=0.0, "Voltage Low [V]"=0.0, "Change"=FALSE, "Current Control"=enum."Closed Loop", "Period [s]"=0.0, "Pulse Width [s]"=0.0, "Profile"=0, "Voltage Control"=FALSE}, {"Drive"=enum."Idle", "Direction"=FALSE, "Phase Step"=enum."Duration", "Duration [s]"=0.0, "Current High [A]"=0.0, "Current Low [A]"=0.0, "Voltage High [V]"=0.0, "Voltage Low [V]"=0.0, "Change"=FALSE, "Current Control"=enum."Closed Loop", "Period [s]"=0.0, "Pulse Width [s]"=0.0, "Profile"=0, "Voltage Control"=FALSE}, {"Drive"=enum."Idle", "Direction"=FALSE, "Phase Step"=enum."Duration", "Duration [s]"=0.0, "Current High [A]"=0.0, "Current Low [A]"=0.0, "Voltage High [V]"=0.0, "Voltage Low [V]"=0.0, "Change"=FALSE, "Current Control"=enum."Closed Loop", "Period [s]"=0.0, "Pulse Width [s]"=0.0, "Profile"=0, "Voltage Control"=FALSE}, {"Drive"=enum."Idle", "Direction"=FALSE, "Phase Step"=enum."Duration", "Duration [s]"=0.0, "Current High [A]"=0.0, "Current Low [A]"=0.0, "Voltage High [V]"=0.0, "Voltage Low [V]"=0.0, "Change"=FALSE, "Current Control"=enum."Closed Loop", "Period [s]"=0.0, "Pulse Width [s]"=0.0, "Profile"=0, "Voltage Control"=FALSE}, {"Drive"=enum."Idle", "Direction"=FALSE, "Phase Step"=enum."Duration", "Duration [s]"=0.0, "Current High [A]"=0.0, "Current Low [A]"=0.0, "Voltage High [V]"=0.0, "Voltage Low [V]"=0.0, "Change"=FALSE, "Current Control"=enum."Closed Loop", "Period [s]"=0.0, "Pulse Width [s]"=0.0, "Profile"=0, "Voltage Control"=FALSE}, {"Drive"=enum."Idle", "Direction"=FALSE, "Phase Step"=enum."Duration", "Duration [s]"=0.0, "Current High [A]"=0.0, "Current Low [A]"=0.0, "Voltage High [V]"=0.0, "Voltage Low [V]"=0.0, "Change"=FALSE, "Current Control"=enum."Closed Loop", "Period [s]"=0.0, "Pulse Width [s]"=0.0, "Profile"=0, "Voltage Control"=FALSE}, {"Drive"=enum."Idle", "Direction"=FALSE, "Phase Step"=enum."Duration", "Duration [s]"=0.0, "Current High [A]"=0.0, "Current Low [A]"=0.0, "Voltage High [V]"=0.0, "Voltage Low [V]"=0.0, "Change"=FALSE, "Current Control"=enum."Closed Loop", "Period [s]"=0.0, "Pulse Width [s]"=0.0, "Profile"=0, "Voltage Control"=FALSE}, {"Drive"=enum."Idle", "Direction"=FALSE, "Phase Step"=enum."Duration", "Duration [s]"=0.0, "Current High [A]"=0.0, "Current Low [A]"=0.0, "Voltage High [V]"=0.0, "Voltage Low [V]"=0.0, "Change"=FALSE, "Current Control"=enum."Closed Loop", "Period [s]"=0.0, "Pulse Width [s]"=0.0, "Profile"=0, "Voltage Control"=FALSE}, {"Drive"=enum."Idle", "Direction"=FALSE, "Phase Step"=enum."Duration", "Duration [s]"=0.0, "Current High [A]"=0.0, "Current Low [A]"=0.0, "Voltage High [V]"=0.0, "Voltage Low [V]"=0.0, "Change"=FALSE, "Current Control"=enum."Closed Loop", "Period [s]"=0.0, "Pulse Width [s]"=0.0, "Profile"=0, "Voltage Control"=FALSE}], [{"Drive"=enum."Idle", "Direction"=FALSE, "Phase Step"=enum."Duration", "Duration [s]"=0.0, "Current High [A]"=0.0, "Current Low [A]"=0.0, "Voltage High [V]"=0.0, "Voltage Low [V]"=0.0, "Change"=FALSE, "Current Control"=enum."Closed Loop", "Period [s]"=0.0, "Pulse Width [s]"=0.0, "Profile"=0, "Voltage Control"=FALSE}, {"Drive"=enum."Idle", "Direction"=FALSE, "Phase Step"=enum."Duration", "Duration [s]"=0.0, "Current High [A]"=0.0, "Current Low [A]"=0.0, "Voltage High [V]"=0.0, "Voltage Low [V]"=0.0, "Change"=FALSE, "Current Control"=enum."Closed Loop", "Period [s]"=0.0, "Pulse Width [s]"=0.0, "Profile"=0, "Voltage Control"=FALSE}, {"Drive"=enum."Idle", "Direction"=FALSE, "Phase Step"=enum."Duration", "Duration [s]"=0.0, "Current High [A]"=0.0, "Current Low [A]"=0.0, "Voltage High [V]"=0.0, "Voltage Low [V]"=0.0, "Change"=FALSE, "Current Control"=enum."Closed Loop", "Period [s]"=0.0, "Pulse Width [s]"=0.0, "Profile"=0, "Voltage Control"=FALSE}, {"Drive"=enum."Idle", "Direction"=FALSE, "Phase Step"=enum."Duration", "Duration [s]"=0.0, "Current High [A]"=0.0, "Current Low [A]"=0.0, "Voltage High [V]"=0.0, "Voltage Low [V]"=0.0, "Change"=FALSE, "Current Control"=enum."Closed Loop", "Period [s]"=0.0, "Pulse Width [s]"=0.0, "Profile"=0, "Voltage Control"=FALSE}, {"Drive"=enum."Idle", "Direction"=FALSE, "Phase Step"=enum."Duration", "Duration [s]"=0.0, "Current High [A]"=0.0, "Current Low [A]"=0.0, "Voltage High [V]"=0.0, "Voltage Low [V]"=0.0, "Change"=FALSE, "Current Control"=enum."Closed Loop", "Period [s]"=0.0, "Pulse Width [s]"=0.0, "Profile"=0, "Voltage Control"=FALSE}, {"Drive"=enum."Idle", "Direction"=FALSE, "Phase Step"=enum."Duration", "Duration [s]"=0.0, "Current High [A]"=0.0, "Current Low [A]"=0.0, "Voltage High [V]"=0.0, "Voltage Low [V]"=0.0, "Change"=FALSE, "Current Control"=enum."Closed Loop", "Period [s]"=0.0, "Pulse Width [s]"=0.0, "Profile"=0, "Voltage Control"=FALSE}, {"Drive"=enum."Idle", "Direction"=FALSE, "Phase Step"=enum."Duration", "Duration [s]"=0.0, "Current High [A]"=0.0, "Current Low [A]"=0.0, "Voltage High [V]"=0.0, "Voltage Low [V]"=0.0, "Change"=FALSE, "Current Control"=enum."Closed Loop", "Period [s]"=0.0, "Pulse Width [s]"=0.0, "Profile"=0, "Voltage Control"=FALSE}, {"Drive"=enum."Idle", "Direction"=FALSE, "Phase Step"=enum."Duration", "Duration [s]"=0.0, "Current High [A]"=0.0, "Current Low [A]"=0.0, "Voltage High [V]"=0.0, "Voltage Low [V]"=0.0, "Change"=FALSE, "Current Control"=enum."Closed Loop", "Period [s]"=0.0, "Pulse Width [s]"=0.0, "Profile"=0, "Voltage Control"=FALSE}, {"Drive"=enum."Idle", "Direction"=FALSE, "Phase Step"=enum."Duration", "Duration [s]"=0.0, "Current High [A]"=0.0, "Current Low [A]"=0.0, "Voltage High [V]"=0.0, "Voltage Low [V]"=0.0, "Change"=FALSE, "Current Control"=enum."Closed Loop", "Period [s]"=0.0, "Pulse Width [s]"=0.0, "Profile"=0, "Voltage Control"=FALSE}, {"Drive"=enum."Idle", "Direction"=FALSE, "Phase Step"=enum."Duration", "Duration [s]"=0.0, "Current High [A]"=0.0, "Current Low [A]"=0.0, "Voltage High [V]"=0.0, "Voltage Low [V]"=0.0, "Change"=FALSE, "Current Control"=enum."Closed Loop", "Period [s]"=0.0, "Pulse Width [s]"=0.0, "Profile"=0, "Voltage Control"=FALSE}, {"Drive"=enum."Idle", "Direction"=FALSE, "Phase Step"=enum."Duration", "Duration [s]"=0.0, "Current High [A]"=0.0, "Current Low [A]"=0.0, "Voltage High [V]"=0.0, "Voltage Low [V]"=0.0, "Change"=FALSE, "Current Control"=enum."Closed Loop", "Period [s]"=0.0, "Pulse Width [s]"=0.0, "Profile"=0, "Voltage Control"=FALSE}, {"Drive"=enum."Idle", "Direction"=FALSE, "Phase Step"=enum."Duration", "Duration [s]"=0.0, "Current High [A]"=0.0, "Current Low [A]"=0.0, "Voltage High [V]"=0.0, "Voltage Low [V]"=0.0, "Change"=FALSE, "Current Control"=enum."Closed Loop", "Period [s]"=0.0, "Pulse Width [s]"=0.0, "Profile"=0, "Voltage Control"=FALSE}, {"Drive"=enum."Idle", "Direction"=FALSE, "Phase Step"=enum."Duration", "Duration [s]"=0.0, "Current High [A]"=0.0, "Current Low [A]"=0.0, "Voltage High [V]"=0.0, "Voltage Low [V]"=0.0, "Change"=FALSE, "Current Control"=enum."Closed Loop", "Period [s]"=0.0, "Pulse Width [s]"=0.0, "Profile"=0, "Voltage Control"=FALSE}, {"Drive"=enum."Idle", "Direction"=FALSE, "Phase Step"=enum."Duration", "Duration [s]"=0.0, "Current High [A]"=0.0, "Current Low [A]"=0.0, "Voltage High [V]"=0.0, "Voltage Low [V]"=0.0, "Change"=FALSE, "Current Control"=enum."Closed Loop", "Period [s]"=0.0, "Pulse Width [s]"=0.0, "Profile"=0, "Voltage Control"=FALSE}, {"Drive"=enum."Idle", "Direction"=FALSE, "Phase Step"=enum."Duration", "Duration [s]"=0.0, "Current High [A]"=0.0, "Current Low [A]"=0.0, "Voltage High [V]"=0.0, "Voltage Low [V]"=0.0, "Change"=FALSE, "Current Control"=enum."Closed Loop", "Period [s]"=0.0, "Pulse Width [s]"=0.0, "Profile"=0, "Voltage Control"=FALSE}, {"Drive"=enum."Idle", "Direction"=FALSE, "Phase Step"=enum."Duration", "Duration [s]"=0.0, "Current High [A]"=0.0, "Current Low [A]"=0.0, "Voltage High [V]"=0.0, "Voltage Low [V]"=0.0, "Change"=FALSE, "Current Control"=enum."Closed Loop", "Period [s]"=0.0, "Pulse Width [s]"=0.0, "Profile"=0, "Voltage Control"=FALSE}], [{"Drive"=enum."Idle", "Direction"=FALSE, "Phase Step"=enum."Duration", "Duration [s]"=0.0, "Current High [A]"=0.0, "Current Low [A]"=0.0, "Voltage High [V]"=0.0, "Voltage Low [V]"=0.0, "Change"=FALSE, "Current Control"=enum."Closed Loop", "Period [s]"=0.0, "Pulse Width [s]"=0.0, "Profile"=0, "Voltage Control"=FALSE}, {"Drive"=enum."Idle", "Direction"=FALSE, "Phase Step"=enum."Duration", "Duration [s]"=0.0, "Current High [A]"=0.0, "Current Low [A]"=0.0, "Voltage High [V]"=0.0, "Voltage Low [V]"=0.0, "Change"=FALSE, "Current Control"=enum."Closed Loop", "Period [s]"=0.0, "Pulse Width [s]"=0.0, "Profile"=0, "Voltage Control"=FALSE}, {"Drive"=enum."Idle", "Direction"=FALSE, "Phase Step"=enum."Duration", "Duration [s]"=0.0, "Current High [A]"=0.0, "Current Low [A]"=0.0, "Voltage High [V]"=0.0, "Voltage Low [V]"=0.0, "Change"=FALSE, "Current Control"=enum."Closed Loop", "Period [s]"=0.0, "Pulse Width [s]"=0.0, "Profile"=0, "Voltage Control"=FALSE}, {"Drive"=enum."Idle", "Direction"=FALSE, "Phase Step"=enum."Duration", "Duration [s]"=0.0, "Current High [A]"=0.0, "Current Low [A]"=0.0, "Voltage High [V]"=0.0, "Voltage Low [V]"=0.0, "Change"=FALSE, "Current Control"=enum."Closed Loop", "Period [s]"=0.0, "Pulse Width [s]"=0.0, "Profile"=0, "Voltage Control"=FALSE}, {"Drive"=enum."Idle", "Direction"=FALSE, "Phase Step"=enum."Duration", "Duration [s]"=0.0, "Current High [A]"=0.0, "Current Low [A]"=0.0, "Voltage High [V]"=0.0, "Voltage Low [V]"=0.0, "Change"=FALSE, "Current Control"=enum."Closed Loop", "Period [s]"=0.0, "Pulse Width [s]"=0.0, "Profile"=0, "Voltage Control"=FALSE}, {"Drive"=enum."Idle", "Direction"=FALSE, "Phase Step"=enum."Duration", "Duration [s]"=0.0, "Current High [A]"=0.0, "Current Low [A]"=0.0, "Voltage High [V]"=0.0, "Voltage Low [V]"=0.0, "Change"=FALSE, "Current Control"=enum."Closed Loop", "Period [s]"=0.0, "Pulse Width [s]"=0.0, "Profile"=0, "Voltage Control"=FALSE}, {"Drive"=enum."Idle", "Direction"=FALSE, "Phase Step"=enum."Duration", "Duration [s]"=0.0, "Current High [A]"=0.0, "Current Low [A]"=0.0, "Voltage High [V]"=0.0, "Voltage Low [V]"=0.0, "Change"=FALSE, "Current Control"=enum."Closed Loop", "Period [s]"=0.0, "Pulse Width [s]"=0.0, "Profile"=0, "Voltage Control"=FALSE}, {"Drive"=enum."Idle", "Direction"=FALSE, "Phase Step"=enum."Duration", "Duration [s]"=0.0, "Current High [A]"=0.0, "Current Low [A]"=0.0, "Voltage High [V]"=0.0, "Voltage Low [V]"=0.0, "Change"=FALSE, "Current Control"=enum."Closed Loop", "Period [s]"=0.0, "Pulse Width [s]"=0.0, "Profile"=0, "Voltage Control"=FALSE}, {"Drive"=enum."Idle", "Direction"=FALSE, "Phase Step"=enum."Duration", "Duration [s]"=0.0, "Current High [A]"=0.0, "Current Low [A]"=0.0, "Voltage High [V]"=0.0, "Voltage Low [V]"=0.0, "Change"=FALSE, "Current Control"=enum."Closed Loop", "Period [s]"=0.0, "Pulse Width [s]"=0.0, "Profile"=0, "Voltage Control"=FALSE}, {"Drive"=enum."Idle", "Direction"=FALSE, "Phase Step"=enum."Duration", "Duration [s]"=0.0, "Current High [A]"=0.0, "Current Low [A]"=0.0, "Voltage High [V]"=0.0, "Voltage Low [V]"=0.0, "Change"=FALSE, "Current Control"=enum."Closed Loop", "Period [s]"=0.0, "Pulse Width [s]"=0.0, "Profile"=0, "Voltage Control"=FALSE}, {"Drive"=enum."Idle", "Direction"=FALSE, "Phase Step"=enum."Duration", "Duration [s]"=0.0, "Current High [A]"=0.0, "Current Low [A]"=0.0, "Voltage High [V]"=0.0, "Voltage Low [V]"=0.0, "Change"=FALSE, "Current Control"=enum."Closed Loop", "Period [s]"=0.0, "Pulse Width [s]"=0.0, "Profile"=0, "Voltage Control"=FALSE}, {"Drive"=enum."Idle", "Direction"=FALSE, "Phase Step"=enum."Duration", "Duration [s]"=0.0, "Current High [A]"=0.0, "Current Low [A]"=0.0, "Voltage High [V]"=0.0, "Voltage Low [V]"=0.0, "Change"=FALSE, "Current Control"=enum."Closed Loop", "Period [s]"=0.0, "Pulse Width [s]"=0.0, "Profile"=0, "Voltage Control"=FALSE}, {"Drive"=enum."Idle", "Direction"=FALSE, "Phase Step"=enum."Duration", "Duration [s]"=0.0, "Current High [A]"=0.0, "Current Low [A]"=0.0, "Voltage High [V]"=0.0, "Voltage Low [V]"=0.0, "Change"=FALSE, "Current Control"=enum."Closed Loop", "Period [s]"=0.0, "Pulse Width [s]"=0.0, "Profile"=0, "Voltage Control"=FALSE}, {"Drive"=enum."Idle", "Direction"=FALSE, "Phase Step"=enum."Duration", "Duration [s]"=0.0, "Current High [A]"=0.0, "Current Low [A]"=0.0, "Voltage High [V]"=0.0, "Voltage Low [V]"=0.0, "Change"=FALSE, "Current Control"=enum."Closed Loop", "Period [s]"=0.0, "Pulse Width [s]"=0.0, "Profile"=0, "Voltage Control"=FALSE}, {"Drive"=enum."Idle", "Direction"=FALSE, "Phase Step"=enum."Duration", "Duration [s]"=0.0, "Current High [A]"=0.0, "Current Low [A]"=0.0, "Voltage High [V]"=0.0, "Voltage Low [V]"=0.0, "Change"=FALSE, "Current Control"=enum."Closed Loop", "Period [s]"=0.0, "Pulse Width [s]"=0.0, "Profile"=0, "Voltage Control"=FALSE}, {"Drive"=enum."Idle", "Direction"=FALSE, "Phase Step"=enum."Duration", "Duration [s]"=0.0, "Current High [A]"=0.0, "Current Low [A]"=0.0, "Voltage High [V]"=0.0, "Voltage Low [V]"=0.0, "Change"=FALSE, "Current Control"=enum."Closed Loop", "Period [s]"=0.0, "Pulse Width [s]"=0.0, "Profile"=0, "Voltage Control"=FALSE}], [{"Drive"=enum."Idle", "Direction"=FALSE, "Phase Step"=enum."Duration", "Duration [s]"=0.0, "Current High [A]"=0.0, "Current Low [A]"=0.0, "Voltage High [V]"=0.0, "Voltage Low [V]"=0.0, "Change"=FALSE, "Current Control"=enum."Closed Loop", "Period [s]"=0.0, "Pulse Width [s]"=0.0, "Profile"=0, "Voltage Control"=FALSE}, {"Drive"=enum."Idle", "Direction"=FALSE, "Phase Step"=enum."Duration", "Duration [s]"=0.0, "Current High [A]"=0.0, "Current Low [A]"=0.0, "Voltage High [V]"=0.0, "Voltage Low [V]"=0.0, "Change"=FALSE, "Current Control"=enum."Closed Loop", "Period [s]"=0.0, "Pulse Width [s]"=0.0, "Profile"=0, "Voltage Control"=FALSE}, {"Drive"=enum."Idle", "Direction"=FALSE, "Phase Step"=enum."Duration", "Duration [s]"=0.0, "Current High [A]"=0.0, "Current Low [A]"=0.0, "Voltage High [V]"=0.0, "Voltage Low [V]"=0.0, "Change"=FALSE, "Current Control"=enum."Closed Loop", "Period [s]"=0.0, "Pulse Width [s]"=0.0, "Profile"=0, "Voltage Control"=FALSE}, {"Drive"=enum."Idle", "Direction"=FALSE, "Phase Step"=enum."Duration", "Duration [s]"=0.0, "Current High [A]"=0.0, "Current Low [A]"=0.0, "Voltage High [V]"=0.0, "Voltage Low [V]"=0.0, "Change"=FALSE, "Current Control"=enum."Closed Loop", "Period [s]"=0.0, "Pulse Width [s]"=0.0, "Profile"=0, "Voltage Control"=FALSE}, {"Drive"=enum."Idle", "Direction"=FALSE, "Phase Step"=enum."Duration", "Duration [s]"=0.0, "Current High [A]"=0.0, "Current Low [A]"=0.0, "Voltage High [V]"=0.0, "Voltage Low [V]"=0.0, "Change"=FALSE, "Current Control"=enum."Closed Loop", "Period [s]"=0.0, "Pulse Width [s]"=0.0, "Profile"=0, "Voltage Control"=FALSE}, {"Drive"=enum."Idle", "Direction"=FALSE, "Phase Step"=enum."Duration", "Duration [s]"=0.0, "Current High [A]"=0.0, "Current Low [A]"=0.0, "Voltage High [V]"=0.0, "Voltage Low [V]"=0.0, "Change"=FALSE, "Current Control"=enum."Closed Loop", "Period [s]"=0.0, "Pulse Width [s]"=0.0, "Profile"=0, "Voltage Control"=FALSE}, {"Drive"=enum."Idle", "Direction"=FALSE, "Phase Step"=enum."Duration", "Duration [s]"=0.0, "Current High [A]"=0.0, "Current Low [A]"=0.0, "Voltage High [V]"=0.0, "Voltage Low [V]"=0.0, "Change"=FALSE, "Current Control"=enum."Closed Loop", "Period [s]"=0.0, "Pulse Width [s]"=0.0, "Profile"=0, "Voltage Control"=FALSE}, {"Drive"=enum."Idle", "Direction"=FALSE, "Phase Step"=enum."Duration", "Duration [s]"=0.0, "Current High [A]"=0.0, "Current Low [A]"=0.0, "Voltage High [V]"=0.0, "Voltage Low [V]"=0.0, "Change"=FALSE, "Current Control"=enum."Closed Loop", "Period [s]"=0.0, "Pulse Width [s]"=0.0, "Profile"=0, "Voltage Control"=FALSE}, {"Drive"=enum."Idle", "Direction"=FALSE, "Phase Step"=enum."Duration", "Duration [s]"=0.0, "Current High [A]"=0.0, "Current Low [A]"=0.0, "Voltage High [V]"=0.0, "Voltage Low [V]"=0.0, "Change"=FALSE, "Current Control"=enum."Closed Loop", "Period [s]"=0.0, "Pulse Width [s]"=0.0, "Profile"=0, "Voltage Control"=FALSE}, {"Drive"=enum."Idle", "Direction"=FALSE, "Phase Step"=enum."Duration", "Duration [s]"=0.0, "Current High [A]"=0.0, "Current Low [A]"=0.0, "Voltage High [V]"=0.0, "Voltage Low [V]"=0.0, "Change"=FALSE, "Current Control"=enum."Closed Loop", "Period [s]"=0.0, "Pulse Width [s]"=0.0, "Profile"=0, "Voltage Control"=FALSE}, {"Drive"=enum."Idle", "Direction"=FALSE, "Phase Step"=enum."Duration", "Duration [s]"=0.0, "Current High [A]"=0.0, "Current Low [A]"=0.0, "Voltage High [V]"=0.0, "Voltage Low [V]"=0.0, "Change"=FALSE, "Current Control"=enum."Closed Loop", "Period [s]"=0.0, "Pulse Width [s]"=0.0, "Profile"=0, "Voltage Control"=FALSE}, {"Drive"=enum."Idle", "Direction"=FALSE, "Phase Step"=enum."Duration", "Duration [s]"=0.0, "Current High [A]"=0.0, "Current Low [A]"=0.0, "Voltage High [V]"=0.0, "Voltage Low [V]"=0.0, "Change"=FALSE, "Current Control"=enum."Closed Loop", "Period [s]"=0.0, "Pulse Width [s]"=0.0, "Profile"=0, "Voltage Control"=FALSE}, {"Drive"=enum."Idle", "Direction"=FALSE, "Phase Step"=enum."Duration", "Duration [s]"=0.0, "Current High [A]"=0.0, "Current Low [A]"=0.0, "Voltage High [V]"=0.0, "Voltage Low [V]"=0.0, "Change"=FALSE, "Current Control"=enum."Closed Loop", "Period [s]"=0.0, "Pulse Width [s]"=0.0, "Profile"=0, "Voltage Control"=FALSE}, {"Drive"=enum."Idle", "Direction"=FALSE, "Phase Step"=enum."Duration", "Duration [s]"=0.0, "Current High [A]"=0.0, "Current Low [A]"=0.0, "Voltage High [V]"=0.0, "Voltage Low [V]"=0.0, "Change"=FALSE, "Current Control"=enum."Closed Loop", "Period [s]"=0.0, "Pulse Width [s]"=0.0, "Profile"=0, "Voltage Control"=FALSE}, {"Drive"=enum."Idle", "Direction"=FALSE, "Phase Step"=enum."Duration", "Duration [s]"=0.0, "Current High [A]"=0.0, "Current Low [A]"=0.0, "Voltage High [V]"=0.0, "Voltage Low [V]"=0.0, "Change"=FALSE, "Current Control"=enum."Closed Loop", "Period [s]"=0.0, "Pulse Width [s]"=0.0, "Profile"=0, "Voltage Control"=FALSE}, {"Drive"=enum."Idle", "Direction"=FALSE, "Phase Step"=enum."Duration", "Duration [s]"=0.0, "Current High [A]"=0.0, "Current Low [A]"=0.0, "Voltage High [V]"=0.0, "Voltage Low [V]"=0.0, "Change"=FALSE, "Current Control"=enum."Closed Loop", "Period [s]"=0.0, "Pulse Width [s]"=0.0, "Profile"=0, "Voltage Control"=FALSE}], [{"Drive"=enum."Idle", "Direction"=FALSE, "Phase Step"=enum."Duration", "Duration [s]"=0.0, "Current High [A]"=0.0, "Current Low [A]"=0.0, "Voltage High [V]"=0.0, "Voltage Low [V]"=0.0, "Change"=FALSE, "Current Control"=enum."Closed Loop", "Period [s]"=0.0, "Pulse Width [s]"=0.0, "Profile"=0, "Voltage Control"=FALSE}, {"Drive"=enum."Idle", "Direction"=FALSE, "Phase Step"=enum."Duration", "Duration [s]"=0.0, "Current High [A]"=0.0, "Current Low [A]"=0.0, "Voltage High [V]"=0.0, "Voltage Low [V]"=0.0, "Change"=FALSE, "Current Control"=enum."Closed Loop", "Period [s]"=0.0, "Pulse Width [s]"=0.0, "Profile"=0, "Voltage Control"=FALSE}, {"Drive"=enum."Idle", "Direction"=FALSE, "Phase Step"=enum."Duration", "Duration [s]"=0.0, "Current High [A]"=0.0, "Current Low [A]"=0.0, "Voltage High [V]"=0.0, "Voltage Low [V]"=0.0, "Change"=FALSE, "Current Control"=enum."Closed Loop", "Period [s]"=0.0, "Pulse Width [s]"=0.0, "Profile"=0, "Voltage Control"=FALSE}, {"Drive"=enum."Idle", "Direction"=FALSE, "Phase Step"=enum."Duration", "Duration [s]"=0.0, "Current High [A]"=0.0, "Current Low [A]"=0.0, "Voltage High [V]"=0.0, "Voltage Low [V]"=0.0, "Change"=FALSE, "Current Control"=enum."Closed Loop", "Period [s]"=0.0, "Pulse Width [s]"=0.0, "Profile"=0, "Voltage Control"=FALSE}, {"Drive"=enum."Idle", "Direction"=FALSE, "Phase Step"=enum."Duration", "Duration [s]"=0.0, "Current High [A]"=0.0, "Current Low [A]"=0.0, "Voltage High [V]"=0.0, "Voltage Low [V]"=0.0, "Change"=FALSE, "Current Control"=enum."Closed Loop", "Period [s]"=0.0, "Pulse Width [s]"=0.0, "Profile"=0, "Voltage Control"=FALSE}, {"Drive"=enum."Idle", "Direction"=FALSE, "Phase Step"=enum."Duration", "Duration [s]"=0.0, "Current High [A]"=0.0, "Current Low [A]"=0.0, "Voltage High [V]"=0.0, "Voltage Low [V]"=0.0, "Change"=FALSE, "Current Control"=enum."Closed Loop", "Period [s]"=0.0, "Pulse Width [s]"=0.0, "Profile"=0, "Voltage Control"=FALSE}, {"Drive"=enum."Idle", "Direction"=FALSE, "Phase Step"=enum."Duration", "Duration [s]"=0.0, "Current High [A]"=0.0, "Current Low [A]"=0.0, "Voltage High [V]"=0.0, "Voltage Low [V]"=0.0, "Change"=FALSE, "Current Control"=enum."Closed Loop", "Period [s]"=0.0, "Pulse Width [s]"=0.0, "Profile"=0, "Voltage Control"=FALSE}, {"Drive"=enum."Idle", "Direction"=FALSE, "Phase Step"=enum."Duration", "Duration [s]"=0.0, "Current High [A]"=0.0, "Current Low [A]"=0.0, "Voltage High [V]"=0.0, "Voltage Low [V]"=0.0, "Change"=FALSE, "Current Control"=enum."Closed Loop", "Period [s]"=0.0, "Pulse Width [s]"=0.0, "Profile"=0, "Voltage Control"=FALSE}, {"Drive"=enum."Idle", "Direction"=FALSE, "Phase Step"=enum."Duration", "Duration [s]"=0.0, "Current High [A]"=0.0, "Current Low [A]"=0.0, "Voltage High [V]"=0.0, "Voltage Low [V]"=0.0, "Change"=FALSE, "Current Control"=enum."Closed Loop", "Period [s]"=0.0, "Pulse Width [s]"=0.0, "Profile"=0, "Voltage Control"=FALSE}, {"Drive"=enum."Idle", "Direction"=FALSE, "Phase Step"=enum."Duration", "Duration [s]"=0.0, "Current High [A]"=0.0, "Current Low [A]"=0.0, "Voltage High [V]"=0.0, "Voltage Low [V]"=0.0, "Change"=FALSE, "Current Control"=enum."Closed Loop", "Period [s]"=0.0, "Pulse Width [s]"=0.0, "Profile"=0, "Voltage Control"=FALSE}, {"Drive"=enum."Idle", "Direction"=FALSE, "Phase Step"=enum."Duration", "Duration [s]"=0.0, "Current High [A]"=0.0, "Current Low [A]"=0.0, "Voltage High [V]"=0.0, "Voltage Low [V]"=0.0, "Change"=FALSE, "Current Control"=enum."Closed Loop", "Period [s]"=0.0, "Pulse Width [s]"=0.0, "Profile"=0, "Voltage Control"=FALSE}, {"Drive"=enum."Idle", "Direction"=FALSE, "Phase Step"=enum."Duration", "Duration [s]"=0.0, "Current High [A]"=0.0, "Current Low [A]"=0.0, "Voltage High [V]"=0.0, "Voltage Low [V]"=0.0, "Change"=FALSE, "Current Control"=enum."Closed Loop", "Period [s]"=0.0, "Pulse Width [s]"=0.0, "Profile"=0, "Voltage Control"=FALSE}, {"Drive"=enum."Idle", "Direction"=FALSE, "Phase Step"=enum."Duration", "Duration [s]"=0.0, "Current High [A]"=0.0, "Current Low [A]"=0.0, "Voltage High [V]"=0.0, "Voltage Low [V]"=0.0, "Change"=FALSE, "Current Control"=enum."Closed Loop", "Period [s]"=0.0, "Pulse Width [s]"=0.0, "Profile"=0, "Voltage Control"=FALSE}, {"Drive"=enum."Idle", "Direction"=FALSE, "Phase Step"=enum."Duration", "Duration [s]"=0.0, "Current High [A]"=0.0, "Current Low [A]"=0.0, "Voltage High [V]"=0.0, "Voltage Low [V]"=0.0, "Change"=FALSE, "Current Control"=enum."Closed Loop", "Period [s]"=0.0, "Pulse Width [s]"=0.0, "Profile"=0, "Voltage Control"=FALSE}, {"Drive"=enum."Idle", "Direction"=FALSE, "Phase Step"=enum."Duration", "Duration [s]"=0.0, "Current High [A]"=0.0, "Current Low [A]"=0.0, "Voltage High [V]"=0.0, "Voltage Low [V]"=0.0, "Change"=FALSE, "Current Control"=enum."Closed Loop", "Period [s]"=0.0, "Pulse Width [s]"=0.0, "Profile"=0, "Voltage Control"=FALSE}, {"Drive"=enum."Idle", "Direction"=FALSE, "Phase Step"=enum."Duration", "Duration [s]"=0.0, "Current High [A]"=0.0, "Current Low [A]"=0.0, "Voltage High [V]"=0.0, "Voltage Low [V]"=0.0, "Change"=FALSE, "Current Control"=enum."Closed Loop", "Period [s]"=0.0, "Pulse Width [s]"=0.0, "Profile"=0, "Voltage Control"=FALSE}], [{"Drive"=enum."Idle", "Direction"=FALSE, "Phase Step"=enum."Duration", "Duration [s]"=0.0, "Current High [A]"=0.0, "Current Low [A]"=0.0, "Voltage High [V]"=0.0, "Voltage Low [V]"=0.0, "Change"=FALSE, "Current Control"=enum."Closed Loop", "Period [s]"=0.0, "Pulse Width [s]"=0.0, "Profile"=0, "Voltage Control"=FALSE}, {"Drive"=enum."Idle", "Direction"=FALSE, "Phase Step"=enum."Duration", "Duration [s]"=0.0, "Current High [A]"=0.0, "Current Low [A]"=0.0, "Voltage High [V]"=0.0, "Voltage Low [V]"=0.0, "Change"=FALSE, "Current Control"=enum."Closed Loop", "Period [s]"=0.0, "Pulse Width [s]"=0.0, "Profile"=0, "Voltage Control"=FALSE}, {"Drive"=enum."Idle", "Direction"=FALSE, "Phase Step"=enum."Duration", "Duration [s]"=0.0, "Current High [A]"=0.0, "Current Low [A]"=0.0, "Voltage High [V]"=0.0, "Voltage Low [V]"=0.0, "Change"=FALSE, "Current Control"=enum."Closed Loop", "Period [s]"=0.0, "Pulse Width [s]"=0.0, "Profile"=0, "Voltage Control"=FALSE}, {"Drive"=enum."Idle", "Direction"=FALSE, "Phase Step"=enum."Duration", "Duration [s]"=0.0, "Current High [A]"=0.0, "Current Low [A]"=0.0, "Voltage High [V]"=0.0, "Voltage Low [V]"=0.0, "Change"=FALSE, "Current Control"=enum."Closed Loop", "Period [s]"=0.0, "Pulse Width [s]"=0.0, "Profile"=0, "Voltage Control"=FALSE}, {"Drive"=enum."Idle", "Direction"=FALSE, "Phase Step"=enum."Duration", "Duration [s]"=0.0, "Current High [A]"=0.0, "Current Low [A]"=0.0, "Voltage High [V]"=0.0, "Voltage Low [V]"=0.0, "Change"=FALSE, "Current Control"=enum."Closed Loop", "Period [s]"=0.0, "Pulse Width [s]"=0.0, "Profile"=0, "Voltage Control"=FALSE}, {"Drive"=enum."Idle", "Direction"=FALSE, "Phase Step"=enum."Duration", "Duration [s]"=0.0, "Current High [A]"=0.0, "Current Low [A]"=0.0, "Voltage High [V]"=0.0, "Voltage Low [V]"=0.0, "Change"=FALSE, "Current Control"=enum."Closed Loop", "Period [s]"=0.0, "Pulse Width [s]"=0.0, "Profile"=0, "Voltage Control"=FALSE}, {"Drive"=enum."Idle", "Direction"=FALSE, "Phase Step"=enum."Duration", "Duration [s]"=0.0, "Current High [A]"=0.0, "Current Low [A]"=0.0, "Voltage High [V]"=0.0, "Voltage Low [V]"=0.0, "Change"=FALSE, "Current Control"=enum."Closed Loop", "Period [s]"=0.0, "Pulse Width [s]"=0.0, "Profile"=0, "Voltage Control"=FALSE}, {"Drive"=enum."Idle", "Direction"=FALSE, "Phase Step"=enum."Duration", "Duration [s]"=0.0, "Current High [A]"=0.0, "Current Low [A]"=0.0, "Voltage High [V]"=0.0, "Voltage Low [V]"=0.0, "Change"=FALSE, "Current Control"=enum."Closed Loop", "Period [s]"=0.0, "Pulse Width [s]"=0.0, "Profile"=0, "Voltage Control"=FALSE}, {"Drive"=enum."Idle", "Direction"=FALSE, "Phase Step"=enum."Duration", "Duration [s]"=0.0, "Current High [A]"=0.0, "Current Low [A]"=0.0, "Voltage High [V]"=0.0, "Voltage Low [V]"=0.0, "Change"=FALSE, "Current Control"=enum."Closed Loop", "Period [s]"=0.0, "Pulse Width [s]"=0.0, "Profile"=0, "Voltage Control"=FALSE}, {"Drive"=enum."Idle", "Direction"=FALSE, "Phase Step"=enum."Duration", "Duration [s]"=0.0, "Current High [A]"=0.0, "Current Low [A]"=0.0, "Voltage High [V]"=0.0, "Voltage Low [V]"=0.0, "Change"=FALSE, "Current Control"=enum."Closed Loop", "Period [s]"=0.0, "Pulse Width [s]"=0.0, "Profile"=0, "Voltage Control"=FALSE}, {"Drive"=enum."Idle", "Direction"=FALSE, "Phase Step"=enum."Duration", "Duration [s]"=0.0, "Current High [A]"=0.0, "Current Low [A]"=0.0, "Voltage High [V]"=0.0, "Voltage Low [V]"=0.0, "Change"=FALSE, "Current Control"=enum."Closed Loop", "Period [s]"=0.0, "Pulse Width [s]"=0.0, "Profile"=0, "Voltage Control"=FALSE}, {"Drive"=enum."Idle", "Direction"=FALSE, "Phase Step"=enum."Duration", "Duration [s]"=0.0, "Current High [A]"=0.0, "Current Low [A]"=0.0, "Voltage High [V]"=0.0, "Voltage Low [V]"=0.0, "Change"=FALSE, "Current Control"=enum."Closed Loop", "Period [s]"=0.0, "Pulse Width [s]"=0.0, "Profile"=0, "Voltage Control"=FALSE}, {"Drive"=enum."Idle", "Direction"=FALSE, "Phase Step"=enum."Duration", "Duration [s]"=0.0, "Current High [A]"=0.0, "Current Low [A]"=0.0, "Voltage High [V]"=0.0, "Voltage Low [V]"=0.0, "Change"=FALSE, "Current Control"=enum."Closed Loop", "Period [s]"=0.0, "Pulse Width [s]"=0.0, "Profile"=0, "Voltage Control"=FALSE}, {"Drive"=enum."Idle", "Direction"=FALSE, "Phase Step"=enum."Duration", "Duration [s]"=0.0, "Current High [A]"=0.0, "Current Low [A]"=0.0, "Voltage High [V]"=0.0, "Voltage Low [V]"=0.0, "Change"=FALSE, "Current Control"=enum."Closed Loop", "Period [s]"=0.0, "Pulse Width [s]"=0.0, "Profile"=0, "Voltage Control"=FALSE}, {"Drive"=enum."Idle", "Direction"=FALSE, "Phase Step"=enum."Duration", "Duration [s]"=0.0, "Current High [A]"=0.0, "Current Low [A]"=0.0, "Voltage High [V]"=0.0, "Voltage Low [V]"=0.0, "Change"=FALSE, "Current Control"=enum."Closed Loop", "Period [s]"=0.0, "Pulse Width [s]"=0.0, "Profile"=0, "Voltage Control"=FALSE}, {"Drive"=enum."Idle", "Direction"=FALSE, "Phase Step"=enum."Duration", "Duration [s]"=0.0, "Current High [A]"=0.0, "Current Low [A]"=0.0, "Voltage High [V]"=0.0, "Voltage Low [V]"=0.0, "Change"=FALSE, "Current Control"=enum."Closed Loop", "Period [s]"=0.0, "Pulse Width [s]"=0.0, "Profile"=0, "Voltage Control"=FALSE}], [{"Drive"=enum."Idle", "Direction"=FALSE, "Phase Step"=enum."Duration", "Duration [s]"=0.0, "Current High [A]"=0.0, "Current Low [A]"=0.0, "Voltage High [V]"=0.0, "Voltage Low [V]"=0.0, "Change"=FALSE, "Current Control"=enum."Closed Loop", "Period [s]"=0.0, "Pulse Width [s]"=0.0, "Profile"=0, "Voltage Control"=FALSE}, {"Drive"=enum."Idle", "Direction"=FALSE, "Phase Step"=enum."Duration", "Duration [s]"=0.0, "Current High [A]"=0.0, "Current Low [A]"=0.0, "Voltage High [V]"=0.0, "Voltage Low [V]"=0.0, "Change"=FALSE, "Current Control"=enum."Closed Loop", "Period [s]"=0.0, "Pulse Width [s]"=0.0, "Profile"=0, "Voltage Control"=FALSE}, {"Drive"=enum."Idle", "Direction"=FALSE, "Phase Step"=enum."Duration", "Duration [s]"=0.0, "Current High [A]"=0.0, "Current Low [A]"=0.0, "Voltage High [V]"=0.0, "Voltage Low [V]"=0.0, "Change"=FALSE, "Current Control"=enum."Closed Loop", "Period [s]"=0.0, "Pulse Width [s]"=0.0, "Profile"=0, "Voltage Control"=FALSE}, {"Drive"=enum."Idle", "Direction"=FALSE, "Phase Step"=enum."Duration", "Duration [s]"=0.0, "Current High [A]"=0.0, "Current Low [A]"=0.0, "Voltage High [V]"=0.0, "Voltage Low [V]"=0.0, "Change"=FALSE, "Current Control"=enum."Closed Loop", "Period [s]"=0.0, "Pulse Width [s]"=0.0, "Profile"=0, "Voltage Control"=FALSE}, {"Drive"=enum."Idle", "Direction"=FALSE, "Phase Step"=enum."Duration", "Duration [s]"=0.0, "Current High [A]"=0.0, "Current Low [A]"=0.0, "Voltage High [V]"=0.0, "Voltage Low [V]"=0.0, "Change"=FALSE, "Current Control"=enum."Closed Loop", "Period [s]"=0.0, "Pulse Width [s]"=0.0, "Profile"=0, "Voltage Control"=FALSE}, {"Drive"=enum."Idle", "Direction"=FALSE, "Phase Step"=enum."Duration", "Duration [s]"=0.0, "Current High [A]"=0.0, "Current Low [A]"=0.0, "Voltage High [V]"=0.0, "Voltage Low [V]"=0.0, "Change"=FALSE, "Current Control"=enum."Closed Loop", "Period [s]"=0.0, "Pulse Width [s]"=0.0, "Profile"=0, "Voltage Control"=FALSE}, {"Drive"=enum."Idle", "Direction"=FALSE, "Phase Step"=enum."Duration", "Duration [s]"=0.0, "Current High [A]"=0.0, "Current Low [A]"=0.0, "Voltage High [V]"=0.0, "Voltage Low [V]"=0.0, "Change"=FALSE, "Current Control"=enum."Closed Loop", "Period [s]"=0.0, "Pulse Width [s]"=0.0, "Profile"=0, "Voltage Control"=FALSE}, {"Drive"=enum."Idle", "Direction"=FALSE, "Phase Step"=enum."Duration", "Duration [s]"=0.0, "Current High [A]"=0.0, "Current Low [A]"=0.0, "Voltage High [V]"=0.0, "Voltage Low [V]"=0.0, "Change"=FALSE, "Current Control"=enum."Closed Loop", "Period [s]"=0.0, "Pulse Width [s]"=0.0, "Profile"=0, "Voltage Control"=FALSE}, {"Drive"=enum."Idle", "Direction"=FALSE, "Phase Step"=enum."Duration", "Duration [s]"=0.0, "Current High [A]"=0.0, "Current Low [A]"=0.0, "Voltage High [V]"=0.0, "Voltage Low [V]"=0.0, "Change"=FALSE, "Current Control"=enum."Closed Loop", "Period [s]"=0.0, "Pulse Width [s]"=0.0, "Profile"=0, "Voltage Control"=FALSE}, {"Drive"=enum."Idle", "Direction"=FALSE, "Phase Step"=enum."Duration", "Duration [s]"=0.0, "Current High [A]"=0.0, "Current Low [A]"=0.0, "Voltage High [V]"=0.0, "Voltage Low [V]"=0.0, "Change"=FALSE, "Current Control"=enum."Closed Loop", "Period [s]"=0.0, "Pulse Width [s]"=0.0, "Profile"=0, "Voltage Control"=FALSE}, {"Drive"=enum."Idle", "Direction"=FALSE, "Phase Step"=enum."Duration", "Duration [s]"=0.0, "Current High [A]"=0.0, "Current Low [A]"=0.0, "Voltage High [V]"=0.0, "Voltage Low [V]"=0.0, "Change"=FALSE, "Current Control"=enum."Closed Loop", "Period [s]"=0.0, "Pulse Width [s]"=0.0, "Profile"=0, "Voltage Control"=FALSE}, {"Drive"=enum."Idle", "Direction"=FALSE, "Phase Step"=enum."Duration", "Duration [s]"=0.0, "Current High [A]"=0.0, "Current Low [A]"=0.0, "Voltage High [V]"=0.0, "Voltage Low [V]"=0.0, "Change"=FALSE, "Current Control"=enum."Closed Loop", "Period [s]"=0.0, "Pulse Width [s]"=0.0, "Profile"=0, "Voltage Control"=FALSE}, {"Drive"=enum."Idle", "Direction"=FALSE, "Phase Step"=enum."Duration", "Duration [s]"=0.0, "Current High [A]"=0.0, "Current Low [A]"=0.0, "Voltage High [V]"=0.0, "Voltage Low [V]"=0.0, "Change"=FALSE, "Current Control"=enum."Closed Loop", "Period [s]"=0.0, "Pulse Width [s]"=0.0, "Profile"=0, "Voltage Control"=FALSE}, {"Drive"=enum."Idle", "Direction"=FALSE, "Phase Step"=enum."Duration", "Duration [s]"=0.0, "Current High [A]"=0.0, "Current Low [A]"=0.0, "Voltage High [V]"=0.0, "Voltage Low [V]"=0.0, "Change"=FALSE, "Current Control"=enum."Closed Loop", "Period [s]"=0.0, "Pulse Width [s]"=0.0, "Profile"=0, "Voltage Control"=FALSE}, {"Drive"=enum."Idle", "Direction"=FALSE, "Phase Step"=enum."Duration", "Duration [s]"=0.0, "Current High [A]"=0.0, "Current Low [A]"=0.0, "Voltage High [V]"=0.0, "Voltage Low [V]"=0.0, "Change"=FALSE, "Current Control"=enum."Closed Loop", "Period [s]"=0.0, "Pulse Width [s]"=0.0, "Profile"=0, "Voltage Control"=FALSE}, {"Drive"=enum."Idle", "Direction"=FALSE, "Phase Step"=enum."Duration", "Duration [s]"=0.0, "Current High [A]"=0.0, "Current Low [A]"=0.0, "Voltage High [V]"=0.0, "Voltage Low [V]"=0.0, "Change"=FALSE, "Current Control"=enum."Closed Loop", "Period [s]"=0.0, "Pulse Width [s]"=0.0, "Profile"=0, "Voltage Control"=FALSE}], [{"Drive"=enum."Idle", "Direction"=FALSE, "Phase Step"=enum."Duration", "Duration [s]"=0.0, "Current High [A]"=0.0, "Current Low [A]"=0.0, "Voltage High [V]"=0.0, "Voltage Low [V]"=0.0, "Change"=FALSE, "Current Control"=enum."Closed Loop", "Period [s]"=0.0, "Pulse Width [s]"=0.0, "Profile"=0, "Voltage Control"=FALSE}, {"Drive"=enum."Idle", "Direction"=FALSE, "Phase Step"=enum."Duration", "Duration [s]"=0.0, "Current High [A]"=0.0, "Current Low [A]"=0.0, "Voltage High [V]"=0.0, "Voltage Low [V]"=0.0, "Change"=FALSE, "Current Control"=enum."Closed Loop", "Period [s]"=0.0, "Pulse Width [s]"=0.0, "Profile"=0, "Voltage Control"=FALSE}, {"Drive"=enum."Idle", "Direction"=FALSE, "Phase Step"=enum."Duration", "Duration [s]"=0.0, "Current High [A]"=0.0, "Current Low [A]"=0.0, "Voltage High [V]"=0.0, "Voltage Low [V]"=0.0, "Change"=FALSE, "Current Control"=enum."Closed Loop", "Period [s]"=0.0, "Pulse Width [s]"=0.0, "Profile"=0, "Voltage Control"=FALSE}, {"Drive"=enum."Idle", "Direction"=FALSE, "Phase Step"=enum."Duration", "Duration [s]"=0.0, "Current High [A]"=0.0, "Current Low [A]"=0.0, "Voltage High [V]"=0.0, "Voltage Low [V]"=0.0, "Change"=FALSE, "Current Control"=enum."Closed Loop", "Period [s]"=0.0, "Pulse Width [s]"=0.0, "Profile"=0, "Voltage Control"=FALSE}, {"Drive"=enum."Idle", "Direction"=FALSE, "Phase Step"=enum."Duration", "Duration [s]"=0.0, "Current High [A]"=0.0, "Current Low [A]"=0.0, "Voltage High [V]"=0.0, "Voltage Low [V]"=0.0, "Change"=FALSE, "Current Control"=enum."Closed Loop", "Period [s]"=0.0, "Pulse Width [s]"=0.0, "Profile"=0, "Voltage Control"=FALSE}, {"Drive"=enum."Idle", "Direction"=FALSE, "Phase Step"=enum."Duration", "Duration [s]"=0.0, "Current High [A]"=0.0, "Current Low [A]"=0.0, "Voltage High [V]"=0.0, "Voltage Low [V]"=0.0, "Change"=FALSE, "Current Control"=enum."Closed Loop", "Period [s]"=0.0, "Pulse Width [s]"=0.0, "Profile"=0, "Voltage Control"=FALSE}, {"Drive"=enum."Idle", "Direction"=FALSE, "Phase Step"=enum."Duration", "Duration [s]"=0.0, "Current High [A]"=0.0, "Current Low [A]"=0.0, "Voltage High [V]"=0.0, "Voltage Low [V]"=0.0, "Change"=FALSE, "Current Control"=enum."Closed Loop", "Period [s]"=0.0, "Pulse Width [s]"=0.0, "Profile"=0, "Voltage Control"=FALSE}, {"Drive"=enum."Idle", "Direction"=FALSE, "Phase Step"=enum."Duration", "Duration [s]"=0.0, "Current High [A]"=0.0, "Current Low [A]"=0.0, "Voltage High [V]"=0.0, "Voltage Low [V]"=0.0, "Change"=FALSE, "Current Control"=enum."Closed Loop", "Period [s]"=0.0, "Pulse Width [s]"=0.0, "Profile"=0, "Voltage Control"=FALSE}, {"Drive"=enum."Idle", "Direction"=FALSE, "Phase Step"=enum."Duration", "Duration [s]"=0.0, "Current High [A]"=0.0, "Current Low [A]"=0.0, "Voltage High [V]"=0.0, "Voltage Low [V]"=0.0, "Change"=FALSE, "Current Control"=enum."Closed Loop", "Period [s]"=0.0, "Pulse Width [s]"=0.0, "Profile"=0, "Voltage Control"=FALSE}, {"Drive"=enum."Idle", "Direction"=FALSE, "Phase Step"=enum."Duration", "Duration [s]"=0.0, "Current High [A]"=0.0, "Current Low [A]"=0.0, "Voltage High [V]"=0.0, "Voltage Low [V]"=0.0, "Change"=FALSE, "Current Control"=enum."Closed Loop", "Period [s]"=0.0, "Pulse Width [s]"=0.0, "Profile"=0, "Voltage Control"=FALSE}, {"Drive"=enum."Idle", "Direction"=FALSE, "Phase Step"=enum."Duration", "Duration [s]"=0.0, "Current High [A]"=0.0, "Current Low [A]"=0.0, "Voltage High [V]"=0.0, "Voltage Low [V]"=0.0, "Change"=FALSE, "Current Control"=enum."Closed Loop", "Period [s]"=0.0, "Pulse Width [s]"=0.0, "Profile"=0, "Voltage Control"=FALSE}, {"Drive"=enum."Idle", "Direction"=FALSE, "Phase Step"=enum."Duration", "Duration [s]"=0.0, "Current High [A]"=0.0, "Current Low [A]"=0.0, "Voltage High [V]"=0.0, "Voltage Low [V]"=0.0, "Change"=FALSE, "Current Control"=enum."Closed Loop", "Period [s]"=0.0, "Pulse Width [s]"=0.0, "Profile"=0, "Voltage Control"=FALSE}, {"Drive"=enum."Idle", "Direction"=FALSE, "Phase Step"=enum."Duration", "Duration [s]"=0.0, "Current High [A]"=0.0, "Current Low [A]"=0.0, "Voltage High [V]"=0.0, "Voltage Low [V]"=0.0, "Change"=FALSE, "Current Control"=enum."Closed Loop", "Period [s]"=0.0, "Pulse Width [s]"=0.0, "Profile"=0, "Voltage Control"=FALSE}, {"Drive"=enum."Idle", "Direction"=FALSE, "Phase Step"=enum."Duration", "Duration [s]"=0.0, "Current High [A]"=0.0, "Current Low [A]"=0.0, "Voltage High [V]"=0.0, "Voltage Low [V]"=0.0, "Change"=FALSE, "Current Control"=enum."Closed Loop", "Period [s]"=0.0, "Pulse Width [s]"=0.0, "Profile"=0, "Voltage Control"=FALSE}, {"Drive"=enum."Idle", "Direction"=FALSE, "Phase Step"=enum."Duration", "Duration [s]"=0.0, "Current High [A]"=0.0, "Current Low [A]"=0.0, "Voltage High [V]"=0.0, "Voltage Low [V]"=0.0, "Change"=FALSE, "Current Control"=enum."Closed Loop", "Period [s]"=0.0, "Pulse Width [s]"=0.0, "Profile"=0, "Voltage Control"=FALSE}, {"Drive"=enum."Idle", "Direction"=FALSE, "Phase Step"=enum."Duration", "Duration [s]"=0.0, "Current High [A]"=0.0, "Current Low [A]"=0.0, "Voltage High [V]"=0.0, "Voltage Low [V]"=0.0, "Change"=FALSE, "Current Control"=enum."Closed Loop", "Period [s]"=0.0, "Pulse Width [s]"=0.0, "Profile"=0, "Voltage Control"=FALSE}], [{"Drive"=enum."Idle", "Direction"=FALSE, "Phase Step"=enum."Duration", "Duration [s]"=0.0, "Current High [A]"=0.0, "Current Low [A]"=0.0, "Voltage High [V]"=0.0, "Voltage Low [V]"=0.0, "Change"=FALSE, "Current Control"=enum."Closed Loop", "Period [s]"=0.0, "Pulse Width [s]"=0.0, "Profile"=0, "Voltage Control"=FALSE}, {"Drive"=enum."Idle", "Direction"=FALSE, "Phase Step"=enum."Duration", "Duration [s]"=0.0, "Current High [A]"=0.0, "Current Low [A]"=0.0, "Voltage High [V]"=0.0, "Voltage Low [V]"=0.0, "Change"=FALSE, "Current Control"=enum."Closed Loop", "Period [s]"=0.0, "Pulse Width [s]"=0.0, "Profile"=0, "Voltage Control"=FALSE}, {"Drive"=enum."Idle", "Direction"=FALSE, "Phase Step"=enum."Duration", "Duration [s]"=0.0, "Current High [A]"=0.0, "Current Low [A]"=0.0, "Voltage High [V]"=0.0, "Voltage Low [V]"=0.0, "Change"=FALSE, "Current Control"=enum."Closed Loop", "Period [s]"=0.0, "Pulse Width [s]"=0.0, "Profile"=0, "Voltage Control"=FALSE}, {"Drive"=enum."Idle", "Direction"=FALSE, "Phase Step"=enum."Duration", "Duration [s]"=0.0, "Current High [A]"=0.0, "Current Low [A]"=0.0, "Voltage High [V]"=0.0, "Voltage Low [V]"=0.0, "Change"=FALSE, "Current Control"=enum."Closed Loop", "Period [s]"=0.0, "Pulse Width [s]"=0.0, "Profile"=0, "Voltage Control"=FALSE}, {"Drive"=enum."Idle", "Direction"=FALSE, "Phase Step"=enum."Duration", "Duration [s]"=0.0, "Current High [A]"=0.0, "Current Low [A]"=0.0, "Voltage High [V]"=0.0, "Voltage Low [V]"=0.0, "Change"=FALSE, "Current Control"=enum."Closed Loop", "Period [s]"=0.0, "Pulse Width [s]"=0.0, "Profile"=0, "Voltage Control"=FALSE}, {"Drive"=enum."Idle", "Direction"=FALSE, "Phase Step"=enum."Duration", "Duration [s]"=0.0, "Current High [A]"=0.0, "Current Low [A]"=0.0, "Voltage High [V]"=0.0, "Voltage Low [V]"=0.0, "Change"=FALSE, "Current Control"=enum."Closed Loop", "Period [s]"=0.0, "Pulse Width [s]"=0.0, "Profile"=0, "Voltage Control"=FALSE}, {"Drive"=enum."Idle", "Direction"=FALSE, "Phase Step"=enum."Duration", "Duration [s]"=0.0, "Current High [A]"=0.0, "Current Low [A]"=0.0, "Voltage High [V]"=0.0, "Voltage Low [V]"=0.0, "Change"=FALSE, "Current Control"=enum."Closed Loop", "Period [s]"=0.0, "Pulse Width [s]"=0.0, "Profile"=0, "Voltage Control"=FALSE}, {"Drive"=enum."Idle", "Direction"=FALSE, "Phase Step"=enum."Duration", "Duration [s]"=0.0, "Current High [A]"=0.0, "Current Low [A]"=0.0, "Voltage High [V]"=0.0, "Voltage Low [V]"=0.0, "Change"=FALSE, "Current Control"=enum."Closed Loop", "Period [s]"=0.0, "Pulse Width [s]"=0.0, "Profile"=0, "Voltage Control"=FALSE}, {"Drive"=enum."Idle", "Direction"=FALSE, "Phase Step"=enum."Duration", "Duration [s]"=0.0, "Current High [A]"=0.0, "Current Low [A]"=0.0, "Voltage High [V]"=0.0, "Voltage Low [V]"=0.0, "Change"=FALSE, "Current Control"=enum."Closed Loop", "Period [s]"=0.0, "Pulse Width [s]"=0.0, "Profile"=0, "Voltage Control"=FALSE}, {"Drive"=enum."Idle", "Direction"=FALSE, "Phase Step"=enum."Duration", "Duration [s]"=0.0, "Current High [A]"=0.0, "Current Low [A]"=0.0, "Voltage High [V]"=0.0, "Voltage Low [V]"=0.0, "Change"=FALSE, "Current Control"=enum."Closed Loop", "Period [s]"=0.0, "Pulse Width [s]"=0.0, "Profile"=0, "Voltage Control"=FALSE}, {"Drive"=enum."Idle", "Direction"=FALSE, "Phase Step"=enum."Duration", "Duration [s]"=0.0, "Current High [A]"=0.0, "Current Low [A]"=0.0, "Voltage High [V]"=0.0, "Voltage Low [V]"=0.0, "Change"=FALSE, "Current Control"=enum."Closed Loop", "Period [s]"=0.0, "Pulse Width [s]"=0.0, "Profile"=0, "Voltage Control"=FALSE}, {"Drive"=enum."Idle", "Direction"=FALSE, "Phase Step"=enum."Duration", "Duration [s]"=0.0, "Current High [A]"=0.0, "Current Low [A]"=0.0, "Voltage High [V]"=0.0, "Voltage Low [V]"=0.0, "Change"=FALSE, "Current Control"=enum."Closed Loop", "Period [s]"=0.0, "Pulse Width [s]"=0.0, "Profile"=0, "Voltage Control"=FALSE}, {"Drive"=enum."Idle", "Direction"=FALSE, "Phase Step"=enum."Duration", "Duration [s]"=0.0, "Current High [A]"=0.0, "Current Low [A]"=0.0, "Voltage High [V]"=0.0, "Voltage Low [V]"=0.0, "Change"=FALSE, "Current Control"=enum."Closed Loop", "Period [s]"=0.0, "Pulse Width [s]"=0.0, "Profile"=0, "Voltage Control"=FALSE}, {"Drive"=enum."Idle", "Direction"=FALSE, "Phase Step"=enum."Duration", "Duration [s]"=0.0, "Current High [A]"=0.0, "Current Low [A]"=0.0, "Voltage High [V]"=0.0, "Voltage Low [V]"=0.0, "Change"=FALSE, "Current Control"=enum."Closed Loop", "Period [s]"=0.0, "Pulse Width [s]"=0.0, "Profile"=0, "Voltage Control"=FALSE}, {"Drive"=enum."Idle", "Direction"=FALSE, "Phase Step"=enum."Duration", "Duration [s]"=0.0, "Current High [A]"=0.0, "Current Low [A]"=0.0, "Voltage High [V]"=0.0, "Voltage Low [V]"=0.0, "Change"=FALSE, "Current Control"=enum."Closed Loop", "Period [s]"=0.0, "Pulse Width [s]"=0.0, "Profile"=0, "Voltage Control"=FALSE}, {"Drive"=enum."Idle", "Direction"=FALSE, "Phase Step"=enum."Duration", "Duration [s]"=0.0, "Current High [A]"=0.0, "Current Low [A]"=0.0, "Voltage High [V]"=0.0, "Voltage Low [V]"=0.0, "Change"=FALSE, "Current Control"=enum."Closed Loop", "Period [s]"=0.0, "Pulse Width [s]"=0.0, "Profile"=0, "Voltage Control"=FALSE}]] {"Profile" max=15; "Period [s]" min=4e-06 max=0.000102 format="%#_3p"; "Pulse Width [s]" min=0 max=0.000102 format="%#_3p"; "Voltage Low [V]" min=-220 max=220 format="%#_3p"; "Voltage High [V]" min=-220 max=220 format="%#_3p"; "Current Low [A]" min=-40 max=40 format="%#_3p"; "Current High [A]" min=-40 max=40 format="%#_3p"; "Duration [s]" min=0 max=1.67772 format="%#_3p"}
  in  "_DI Scope Event":T18
  out "State":T19 {"System ADC"."Fan [V]" format="%#_3p"; "System ADC"."Primary B1B2 [V]" format="%#_3p"; "System ADC"."Primary B3B4 [V]" format="%#_3p"; "System ADC"."Primary A3A4 [V]" format="%#_3p"; "System ADC"."Primary A1A2 [V]" format="%#_3p"; "System ADC"."MPRD [V]" format="%#_3p"; "System ADC"."Ext HV B [V]" format="%#_3p"; "System ADC"."Ext HV A [V]" format="%#_3p"; "System ADC"."Pump Zener B [V]" format="%#_3p"; "System ADC"."Pump Zener A [V]" format="%#_3p"; "System ADC"."DI Zener B [V]" format="%#_3p"; "System ADC"."DI Zener A [V]" format="%#_3p"; "System ADC"."Key [V]" format="%#_3p"; "System ADC"."DRVP [V]" format="%#_3p"; "System ADC"."Battery [V]" format="%#_3p"; "System ADC"."FET Driver [V]" format="%#_3p"; "System ADC"."Secondary B1B2 [V]" format="%#_3p"; "System ADC"."Secondary B3B4 [V]" format="%#_3p"; "System ADC"."Secondary A3A4 [V]" format="%#_3p"; "System ADC"."Secondary A1A2 [V]" format="%#_3p"; "System ADC"."Primary Range [V]" format="%#_3p"; "System ADC"."Temp Boost B [C]" format="%#_3p"; "System ADC"."Temp Primary A [C]" format="%#_3p"; "System ADC"."Temp Secondary A [C]" format="%#_3p"; "System ADC"."Temp Fan Intake [C]" format="%#_3p"; "System ADC"."Temp CPU [C]" format="%#_3p"; "System ADC"."Temp DI Zener B [C]" format="%#_3p"; "System ADC"."Temp DI B [C]" format="%#_3p"; "System ADC"."Temp DI Zener A [C]" format="%#_3p"; "System ADC"."Temp DI A [C]" format="%#_3p"; "System ADC"."Temp HH 7-12 [C]" format="%#_3p"; "System ADC"."Temp HH 1-6 [C]" format="%#_3p"; "System ADC"."AI 12 [V]" format="%#_3p"; "System ADC"."AI 11 [V]" format="%#_3p"; "System ADC"."AI 10 [V]" format="%#_3p"; "System ADC"."AI 9 [V]" format="%#_3p"; "System ADC"."AI 8 [V]" format="%#_3p"; "System ADC"."AI 7 [V]" format="%#_3p"; "System ADC"."AI 6 [V]" format="%#_3p"; "System ADC"."AI 5 [V]" format="%#_3p"; "System ADC"."AI 4 [V]" format="%#_3p"; "System ADC"."AI 3 [V]" format="%#_3p"; "System ADC"."AI 2 [V]" format="%#_3p"; "System ADC"."AI 1 [V]" format="%#_3p"}
  in  "PumpZenerEnable":bool
  in  "_DI ADC Select":T22
  in  "_Tab Control":T23(tab)
  in  "DI-A Inj Ref Setup":T5(xcontrol)
  in  "_MovePhaseArrayListUp":bool
  in  "_MovePhaseArrayListDown":bool
  in  "_Remove Phase":bool
  in  "_Insert Phase":bool
  in  "Phase Array":i32(listbox)
  in  "PhaseArraysList":i32(listbox)
  out "_Phase Plot":cluster{"Array":dbl[], "Array":dbl[]}[](graph)
  in  "SimInjDuration":sgl=0.001 caption="Simulation Duration [s]" format="%#.3p"
  in  "_Phase":T13 caption="Phase" {"Profile" max=15; "Period [s]" min=4e-06 max=0.000102 format="%#_3p"; "Pulse Width [s]" min=0 max=0.000102 format="%#_3p"; "Voltage Low [V]" min=-220 max=220 format="%#_3p"; "Voltage High [V]" min=-220 max=220 format="%#_3p"; "Current Low [A]" min=-40 max=40 format="%#_3p"; "Current High [A]" min=-40 max=40 format="%#_3p"; "Duration [s]" min=0 max=1.67772 format="%#_3p"}
  in  "_Ref Inj FilePath":path caption="Reference Inj Profile File Path"
  in  "_Save Profile":bool
  in  "_Apply Profile":bool
  in  "DI-A Sim Settings":T5(xcontrol) caption="DI Scope"
  out "_Pump Phase Plot":cluster{"Array":dbl[], "Array":dbl[]}[](graph)
  in  "DI-A Pump Ref Setup":T5(xcontrol)
  in  "_Ref Pump Current Profile FilePath":path caption="Reference Pump Profile File Path"
  in  "_Remove Pump Phase":bool
  in  "_Insert Pump Phase":bool
  in  "PumpPhase Array":i32(listbox)
  in  "_Pump Phase":T13 caption="Pump Phase" {"Profile" max=15; "Period [s]" min=4e-06 max=0.000102 format="%#_3p"; "Pulse Width [s]" min=0 max=0.000102 format="%#_3p"; "Voltage Low [V]" min=-220 max=220 format="%#_3p"; "Voltage High [V]" min=-220 max=220 format="%#_3p"; "Current Low [A]" min=-40 max=40 format="%#_3p"; "Current High [A]" min=-40 max=40 format="%#_3p"; "Duration [s]" min=0 max=1.67772 format="%#_3p"}
  in  "SimPumpDuration":sgl=0.001 caption="Simulation Duration [s]" format="%#.3p"
  in  "DI-A Sim Settings":T5(xcontrol) caption="DI Scope"
  in  "ProfilesAdapt":bool
  out "_Profiles usage tracker":i32(listbox) caption="Profiles usage tracker [Profile, Phase]"
  in  "Profiles":sgl[][](array[numeric]) caption="[]" min=0 max=0.0001 format="%#_6p"
  in  "_InjAdaptMode":bool
  in  "_DI_CopyToAllChannelConf":bool
  in  "_ChannelConfigurationList":i32(listbox)
  in  "_InjCmd Element":T24={"Mode"=enum."Off", "Digital Input"=enum."Unused", "Default Profile Index"=0, "Cal Freq [Hz]"=0.0, "Cal Duration [s]"=0.0, "Cal Increment [s]"=0.0, "Cal Pulses"=0, "TMP Command Sequence"=[{"Duration [s]"=0.0, "CmdLevel"=FALSE, "Continue"=FALSE, "Profile Select"=0}, {"Duration [s]"=0.0, "CmdLevel"=FALSE, "Continue"=FALSE, "Profile Select"=0}, {"Duration [s]"=0.0, "CmdLevel"=FALSE, "Continue"=FALSE, "Profile Select"=0}, {"Duration [s]"=0.0, "CmdLevel"=FALSE, "Continue"=FALSE, "Profile Select"=0}, {"Duration [s]"=0.0, "CmdLevel"=FALSE, "Continue"=FALSE, "Profile Select"=0}, {"Duration [s]"=0.0, "CmdLevel"=FALSE, "Continue"=FALSE, "Profile Select"=0}, {"Duration [s]"=0.0, "CmdLevel"=FALSE, "Continue"=FALSE, "Profile Select"=0}, {"Duration [s]"=0.0, "CmdLevel"=FALSE, "Continue"=FALSE, "Profile Select"=0}], "EPT TDC Offset [CAD]"=0.0, "EPT Window Start [DBTDC]"=0.0, "EPT Window End [DBTDC]"=0.0, "EPT Angles"=[{"Enable"=FALSE, "Timing [CAD]"=0.0, "Duration [s]"=0.0, "Profile Select"=0}, {"Enable"=FALSE, "Timing [CAD]"=0.0, "Duration [s]"=0.0, "Profile Select"=0}, {"Enable"=FALSE, "Timing [CAD]"=0.0, "Duration [s]"=0.0, "Profile Select"=0}, {"Enable"=FALSE, "Timing [CAD]"=0.0, "Duration [s]"=0.0, "Profile Select"=0}, {"Enable"=FALSE, "Timing [CAD]"=0.0, "Duration [s]"=0.0, "Profile Select"=0}, {"Enable"=FALSE, "Timing [CAD]"=0.0, "Duration [s]"=0.0, "Profile Select"=0}, {"Enable"=FALSE, "Timing [CAD]"=0.0, "Duration [s]"=0.0, "Profile Select"=0}, {"Enable"=FALSE, "Timing [CAD]"=0.0, "Duration [s]"=0.0, "Profile Select"=0}], "EPT Skip Fire"=FALSE, "Skip Fire Index"=0, "EPT Precharge Duration [s]"=0.0, "EPT Precharge Profile Index"=0} {"EPT Precharge Profile Index" max=15; "EPT Precharge Duration [s]" min=0 format="%#_4p"; "EPT Angles"."Profile Select" max=15; "EPT Angles"."Duration [s]" min=0 max=1.677722 format="%#_4p"; "EPT Angles"."Timing [CAD]" min=-720 max=720 format="%#_3p"; "TMP Command Sequence"."Profile Select" max=15; "TMP Command Sequence"."Duration [s]" min=0 max=1.677722 format="%#_3p"; "Default Profile Index" max=15; "EPT Window End [DBTDC]" min=-720 max=720; "Skip Fire Index" max=15; "EPT Window Start [DBTDC]" min=-720 max=720; "EPT TDC Offset [CAD]" min=-720 max=720; "Cal Increment [s]" min=0 format="%#_4p"; "Cal Pulses" max=500; "Cal Duration [s]" min=0 max=1.677722 format="%#_4p"; "Cal Freq [Hz]" min=0 format="%#_4p"}
  in  "_Plot Selector (T=TMP, F=EPT)":bool
  out "_Timing Plot":cluster{sgl[], sgl[]}[](graph)
  in  "_Bank Wiring Diagram":T25
  in  "PumpCmd":T26={"Mode"=enum."Off", "Digital Input"=enum."Unused", "Default Profile Index"=0, "Cal Freq [Hz]"=0.0, "Cal Duration [s]"=0.0, "Cal Increment [s]"=0.0, "Cal Pulses"=0, "TMP Command Sequence"=[{"Duration [s]"=0.0, "CmdLevel"=FALSE, "Continue"=FALSE, "Profile Select"=0}, {"Duration [s]"=0.0, "CmdLevel"=FALSE, "Continue"=FALSE, "Profile Select"=0}, {"Duration [s]"=0.0, "CmdLevel"=FALSE, "Continue"=FALSE, "Profile Select"=0}, {"Duration [s]"=0.0, "CmdLevel"=FALSE, "Continue"=FALSE, "Profile Select"=0}, {"Duration [s]"=0.0, "CmdLevel"=FALSE, "Continue"=FALSE, "Profile Select"=0}, {"Duration [s]"=0.0, "CmdLevel"=FALSE, "Continue"=FALSE, "Profile Select"=0}, {"Duration [s]"=0.0, "CmdLevel"=FALSE, "Continue"=FALSE, "Profile Select"=0}, {"Duration [s]"=0.0, "CmdLevel"=FALSE, "Continue"=FALSE, "Profile Select"=0}], "EPT TDC Offset [CAD]"=0.0, "EPT Window Start [DBTDC]"=0.0, "EPT Window End [DBTDC]"=0.0, "EPT Angles"=[{"Enable"=FALSE, "Timing [CAD]"=0.0, "Duration [s]"=0.0, "Profile Select"=0}, {"Enable"=FALSE, "Timing [CAD]"=0.0, "Duration [s]"=0.0, "Profile Select"=0}, {"Enable"=FALSE, "Timing [CAD]"=0.0, "Duration [s]"=0.0, "Profile Select"=0}, {"Enable"=FALSE, "Timing [CAD]"=0.0, "Duration [s]"=0.0, "Profile Select"=0}, {"Enable"=FALSE, "Timing [CAD]"=0.0, "Duration [s]"=0.0, "Profile Select"=0}, {"Enable"=FALSE, "Timing [CAD]"=0.0, "Duration [s]"=0.0, "Profile Select"=0}, {"Enable"=FALSE, "Timing [CAD]"=0.0, "Duration [s]"=0.0, "Profile Select"=0}, {"Enable"=FALSE, "Timing [CAD]"=0.0, "Duration [s]"=0.0, "Profile Select"=0}], "EPT Skip Fire"=FALSE, "Skip Fire Index"=0, "EPT Precharge Duration [s]"=0.0, "EPT Precharge Profile Index"=0} {"EPT Precharge Profile Index" max=15; "EPT Precharge Duration [s]" min=0 format="%#_4p"; "EPT Angles"."Profile Select" max=15; "EPT Angles"."Duration [s]" min=0 max=1.677722 format="%#_4p"; "EPT Angles"."Timing [CAD]" min=-720 max=720 format="%#_3p"; "TMP Command Sequence"."Profile Select" max=15; "TMP Command Sequence"."Duration [s]" min=0 max=1.677722 format="%#_3p"; "Default Profile Index" max=15; "EPT Window End [DBTDC]" min=-720 max=720; "Skip Fire Index" max=15; "EPT Window Start [DBTDC]" min=-720 max=720; "EPT TDC Offset [CAD]" min=-720 max=720; "Cal Increment [s]" min=0 format="%#_4p"; "Cal Pulses" max=500; "Cal Duration [s]" min=0 max=1.677722 format="%#_4p"; "Cal Freq [Hz]" min=0 format="%#_4p"}
  in  "PumpAdaptMode":bool
  in  "_Pump A Plot Selector (T=TMP, F=EPT)":bool
  out "_Pump Timing Plot":cluster{sgl[], sgl[]}[](graph)
  out "_Temp Boost Secondary":sgl(slide)=100.0 caption="[C]" max=100 scale=0.0..80.0 scale format="%#_2f"
  out "_Temp DI":sgl(slide)=21.08 caption="[C]" scale=0.0..80.0 scale format="%#.4f"
  out "_Temp Boost Primary":sgl(slide)=100.0 caption="[C]" max=100 scale=0.0..80.0 scale format="%#_2f"
  out "_Temp DI Zener":sgl(slide)=21.08 caption="[C]" scale=0.0..80.0 scale format="%#.0f"
  in  "_DI-A Fault Clear":T27 caption="Bank A DI Fault Clear"
  out "Faults":T28[](array[typedef]) caption="DI Faults"
  # "DI Bank A Status"
  # "DI Bank A Configuration"
  # "Voltage [DV]"
  # "Voltage [V]"
  # "Sim Injection Duration [s]"
  # "Sim Pump Duration [s]"
  # "Injector Channel Command Configuration"
  # "Enable"
  # "Timing [DBTDC]"
  # "Duration [s]"
  # "Profile Index"
  # "Duration [s]"
  # "Level"
  # "Pause/Continue"
  # "Profile Index"
  # "Pump Channel Command Configuration"
  # "Enable"
  # "Timing [DBTDC]"
  # "Duration [s]"
  # "Profile Index"
  # "Duration [s]"
  # "Level"
  # "Pause/Continue"
  # "Profile Index"
  # "Temp DI"
  # "Temp DI Zener"
  # "Temp Primary"
  # "Temp Secondary"
  # "Bank A DI Fault Clear"
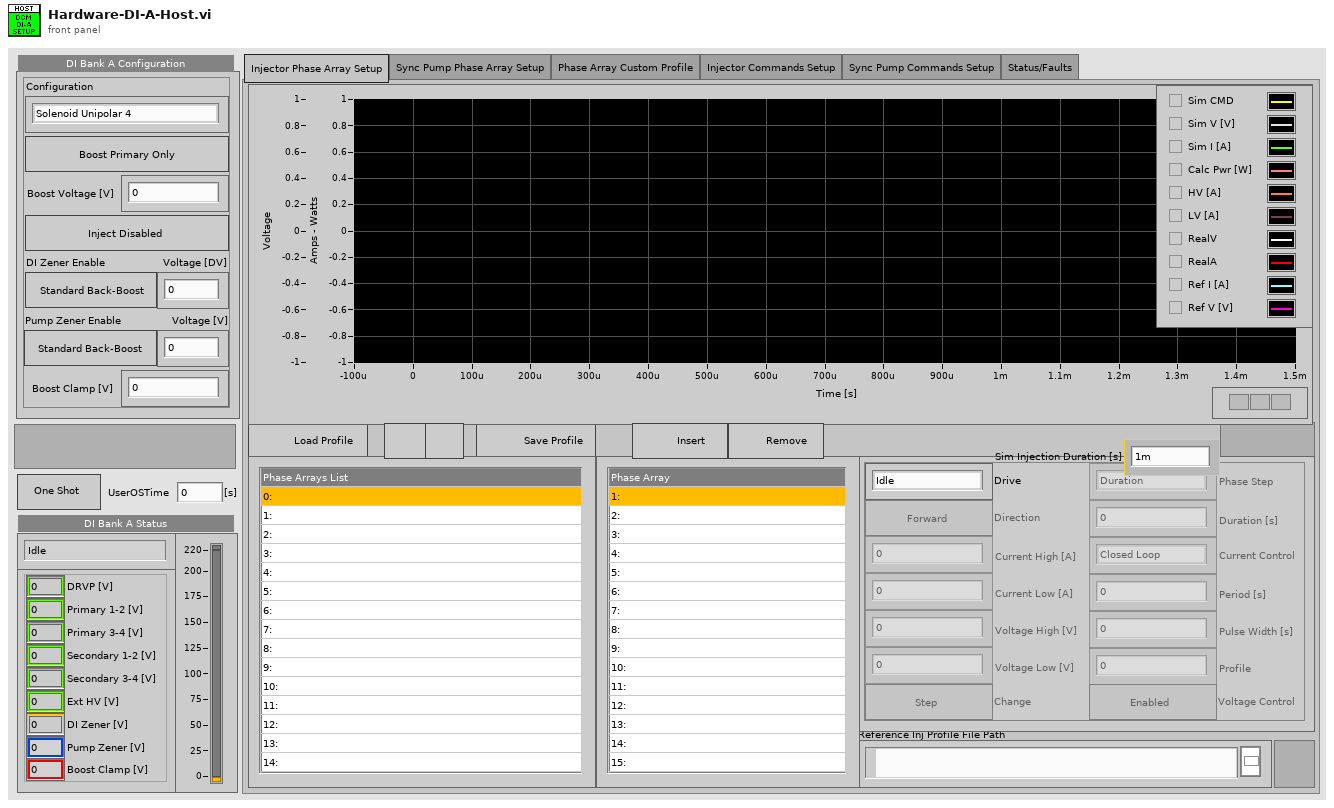
[diagram p1: front panel]
types:
  T1 = typedef "DCM - RT.lvclass/Run State.ctl" = enum8{"Idle", "Warmup", "Ready To Inject", "Cool Down"}
  T2 = cluster{"DRVP [V]":sgl, "Primary 1-2 [V]":sgl, "Primary 3-4 [V]":sgl, "Secondary 1-2 [V]":sgl, "Secondary 3-4 [V]":sgl, "Ext HV [V]":sgl, "DI Zener [V]":sgl, "Pump Zener [V]":sgl, "Boost Clamp [V]":sgl}
  T3 = typedef "DCM - RT.lvclass/Configuration.ctl" = cluster{"Configuration":T4, "Power Supply Enable":bool, "Boost Voltage [V]":sgl, "Inject Enable":bool, "DI Zener Enable":bool, "DI Zener Voltage [V]":sgl, "Pump Zener Enable":bool, "Pump Zener Voltage [V]":sgl, "Boost Clamp [V]":sgl}
  T4 = typedef "DCM - FPGA.lvlib/DI - Bank Configuration.ctl" = enum8{"Solenoid Unipolar 4", "Solenoid Unipolar 7 (Muxed)", "Solenoid Unipolar 8 (Muxed)", "Solenoid Bipolar 2", "Solenoid Bipolar 3 (Muxed)", "Piezo Unipolar 2", "Piezo Unipolar 3 (Muxed)", "Piezo Unipolar 4 (Muxed)", "Piezo Bipolar 2", "Piezo Bipolar 3 (Muxed)"}
  T5 = cluster{"Name":string, "Host VI":path, "Pairing File":path, "Display Name":string}
  T6 = typedef "DSI-Shared.lvlib/DI-Command-Array.ctl" = T7[]
  T7 = typedef "DCM - RT - DI.lvlib/Command.ctl" = cluster{"Mode":T8, "Digital Input":T9, "Default Profile Index":u8, "Cal Freq [Hz]":sgl, "Cal Duration [s]":sgl, "Cal Increment [s]":sgl, "Cal Pulses":u16, "TMP Command Sequence":T10[], "EPT TDC Offset [CAD]":sgl, "EPT Window Start [DBTDC]":sgl, "EPT Window End [DBTDC]":sgl, "EPT Angles":T11[], "EPT Skip Fire":bool, "EPT Skip Index":u8, "EPT Precharge Duration [s]":sgl, "EPT Precharge Profile Index":u8}
  T8 = typedef "DCM - FPGA - DI.lvlib/Mode.ctl" = enum8{"Off", "Direct", "Calibration", "Triggered Multi-Pulse", "Engine Position Tracking"}
  T9 = typedef "DCM - FPGA.lvlib/Digital Channel.ctl" = enum8{"Unused", "User OS", "Diff IO 1", "Diff IO 2", "Diff IO 3", "Diff IO 4", "Diff IO 5", "Diff IO 6", "Diff IO 7", "Diff IO 8", "Aux 1", "Aux 2", "Aux 3", "Aux 4", "Aux 5", "Aux 6", "Aux 7", "Aux 8", "Aux 9", "Aux 10", "Aux 11", "Aux 12", "Aux 13", "Aux 14", "Aux 15", "Aux 16"}
  T10 = typedef "DCM - RT - DI.lvlib/Command Sequence.ctl" = cluster{"Duration [s]":sgl, "Level":bool, "Run/Stop":bool, "Profile Index":u8}
  T11 = typedef "DCM - RT - DI.lvlib/Angle Control.ctl" = cluster{"Enable":bool, "Timing [DBTDC]":sgl, "Duration [s]":sgl, "Profile Index":u8}
  T12 = typedef "DSI-Shared.lvlib/DI-Phase-Array-1D.ctl" = T13[]
  T13 = typedef "DCM - RT - DI.lvlib/Phase.ctl" = cluster{"Drive":T14, "Direction":bool, "Phase Step":T15, "Duration [s]":sgl, "Current High [A]":sgl, "Current Low [A]":sgl, "Voltage High [V]":sgl, "Voltage Low [V]":sgl, "Change":bool, "Current Control":T16, "Period [s]":sgl, "Pulse Width [s]":sgl, "Profile":u8, "Voltage Control":bool}
  T14 = typedef "DCM - FPGA.lvlib/DI - Drive State.ctl" = enum8{"Idle", "HV Current Control", "LV Current Control", "Back Boost", "Piezo Charge", "Piezo Discharge"}
  T15 = typedef "DCM - FPGA - DI.lvlib/Phase Step.ctl" = enum8{"Duration", "First Peak", "End of Cmd", "Branch", "2-Phase Duration"}
  T16 = typedef "DCM - FPGA - DI.lvlib/Control.ctl" = enum8{"Closed Loop", "Fixed Period", "Fixed On Pulse", "Fixed Off Pulse", "Open Loop", "Profile"}
  T17 = typedef "DSI-Shared.lvlib/DI-Phase-Array-2D.ctl" = T13[][]
  T18 = typedef "DCM - FPGA - DI.lvlib/Capture Event.ctl" = enum8{"Unused", "Injector A1", "Injector A2", "Injector A3", "Injector A4", "Injector A5", "Injector A6", "Injector A7", "Injector A8/PumpA", "Injector B1", "Injector B2", "Injector B3", "Injector B4", "Injector B5", "Injector B6", "Injector B7", "Injector B8/PumpB", "User OS", "Diff IO 1", "Diff IO 2", "Diff IO 3", "Diff IO 4", "Diff IO 5", "Diff IO 6", "Diff IO 7", "Diff IO 8", "Aux 1", "Aux 2", "Aux 3", "Aux 4", "Aux 5", "Aux 6", "Aux 7", "Aux 8", "Aux 9", "Aux 10", "Aux 11", "Aux 12", "Aux 13", "Aux 14", "Aux 15", "Aux 16"}
  T19 = typedef "DCM - RT.lvclass/System State.ctl" = cluster{"System ADC":T20, "IO Lock":bool, "HH Mode Config Error":bool, "Fan Speed 1 [RPM]":sgl, "Fan Speed 2 [RPM]":sgl, "Firmware Major Rev":u16, "Firmware Minor Rev":u16, "Internal Fault":T21, "Fault Value":dbl}
  T20 = typedef "DCM - RT.lvclass/System ADC.ctl" = cluster{"AI 1 [V]":sgl, "AI 2 [V]":sgl, "AI 3 [V]":sgl, "AI 4 [V]":sgl, "AI 5 [V]":sgl, "AI 6 [V]":sgl, "AI 7 [V]":sgl, "AI 8 [V]":sgl, "AI 9 [V]":sgl, "AI 10 [V]":sgl, "AI 11 [V]":sgl, "AI 12 [V]":sgl, "Temp HH 1-6 [C]":sgl, "Temp HH 7-12 [C]":sgl, "Temp DI A [C]":sgl, "Temp DI Zener A [C]":sgl, "Temp DI B [C]":sgl, "Temp DI Zener B [C]":sgl, "Temp CPU [C]":sgl, "Temp Fan Intake [C]":sgl, "Temp Secondary A [C]":sgl, "Temp Primary A [C]":sgl, "Temp Boost B [C]":sgl, "Primary Range [V]":sgl, "Primary A1A2 [V]":sgl, "Primary A3A4 [V]":sgl, "Primary B3B4 [V]":sgl, "Primary B1B2 [V]":sgl, "Secondary A1A2 [V]":sgl, "Secondary A3A4 [V]":sgl, "Secondary B3B4 [V]":sgl, "Secondary B1B2 [V]":sgl, "Ext HV A [V]":sgl, "Ext HV B [V]":sgl, "FET Driver [V]":sgl, "Fan [V]":sgl, "Battery [V]":sgl, "DRVP [V]":sgl, "Key [V]":sgl, "DI Zener A [V]":sgl, "DI Zener B [V]":sgl, "Pump Zener A [V]":sgl, "Pump Zener B [V]":sgl, "MPRD [V]":sgl}
  T21 = typedef "DCM - RT.lvclass/Internal Fault.ctl" = enum32{"None", "Temp HH 1-6", "Temp HH 7-12", "Temp DI A", "Temp DI Zener A", "Temp DI B", "Temp DI Zener B", "Temp Intake", "Temp Primary A", "Temp Secondary A", "Temp Boost B", "Temp CPU", "Low Battery", "Inrush Protection", "A Run Enable", "B Run Enable"}
  T22 = typedef "DCM - FPGA.lvlib/DI - ADC Signals.ctl" = enum8{"I LS A1/A5", "I LS A2/A6", "I LS A3/A7", "I LS A4", "I LS A8/PumpA", "V PZ A1", "V PZ A2", "V PZ A3", "V PZ A4", "V S A1", "V S A2", "V S A3", "V S A4", "V S A5", "V S A6", "V S A7", "V S A8", "V Pump A", "V Secondary A1A2", "V Secondary A3A4", "V Ext HV A", "------------------------ ", "I LS B1/B5", "I LS B2/B6", "I LS B3/B7", "I LS B4", "I LS B8/PumpB", "V PZ B1", "V PZ B2", "V PZ B3", "V PZ B4", "V S B1", "V S B2", "V S B3", "V S B4", "V S B5", "V S B6", "V S B7", "V S B8", "V Pump B", "V Secondary B1B2", "V Secondary B3B4", "V Ext HV B", "-------------------------  ", "AI 1", "AI 2", "AI 3", "AI 4", "AI 5", "AI 6", "AI 7", "AI 8", "AI 9", "AI 10", "AI 11", "AI 12", "-------------------------   ", "V DRVP"}
  T23 = enum32{"Injector Phase Array Setup", "Sync Pump Phase Array Setup", "Phase Array Custom Profile", "Injector Commands Setup", "Sync Pump Commands Setup", "Status/Faults"}
  T24 = typedef "DI Command Element.ctl" = cluster{"Mode":enum8{"Off", "Direct", "Calibration", "Triggered Multi-Pulse", "Engine Position Tracking"}, "Digital Input":T9, "Default Profile Index":u8, "Cal Freq [Hz]":sgl, "Cal Duration [s]":sgl, "Cal Increment [s]":sgl, "Cal Pulses":u16, "TMP Command Sequence":cluster{"Duration [s]":sgl, "CmdLevel":bool, "Continue":bool, "Profile Select":u8}[], "EPT TDC Offset [CAD]":sgl, "EPT Window Start [DBTDC]":sgl, "EPT Window End [DBTDC]":sgl, "EPT Angles":cluster{"Enable":bool, "Timing [CAD]":sgl, "Duration [s]":sgl, "Profile Select":u8}[], "EPT Skip Fire":bool, "Skip Fire Index":u8, "EPT Precharge Duration [s]":sgl, "EPT Precharge Profile Index":u8}
  T25 = typedef "DCM - UI.lvlib/Bank A.ctl" = u8
  T26 = typedef "Pump Command Element.ctl" = cluster{"Mode":enum8{"Off", "Direct", "Calibration", "Triggered Multi-Pulse", "Engine Position Tracking"}, "Digital Input":T9, "Default Profile Index":u8, "Cal Freq [Hz]":sgl, "Cal Duration [s]":sgl, "Cal Increment [s]":sgl, "Cal Pulses":u16, "TMP Command Sequence":cluster{"Duration [s]":sgl, "CmdLevel":bool, "Continue":bool, "Profile Select":u8}[], "EPT TDC Offset [CAD]":sgl, "EPT Window Start [DBTDC]":sgl, "EPT Window End [DBTDC]":sgl, "EPT Angles":cluster{"Enable":bool, "Timing [CAD]":sgl, "Duration [s]":sgl, "Profile Select":u8}[], "EPT Skip Fire":bool, "Skip Fire Index":u8, "EPT Precharge Duration [s]":sgl, "EPT Precharge Profile Index":u8}
  T27 = cluster{"DI-A-1 Clear":bool, "DI-A-2 Clear":bool, "DI-A-3 Clear":bool, "DI-A-4 Clear":bool, "DI-A-5 Clear":bool, "DI-A-6 Clear":bool, "DI-A-7 Clear":bool, "DI-A-8 Clear":bool}
  T28 = typedef "DCM - FPGA.lvlib/DI - Faults.ctl" = cluster{"HV Fault":bool, "LV Fault":bool, "LS Fault":bool, "MUX Fault":bool, "Open Warning":bool}
  T29 = enum32{"Invalid", "Standard", "Closed", "Hidden", "Minimized", "Maximized"}
  T30 = enum8{"Enabled", "Disabled", "Disabled and Grayed Out"}
  T31 = cluster{"Configuration":T4, "Power Supply Enable":bool, "Boost Voltage [V]":sgl, "Inject Enable":bool, "Zener Enable":bool, "Zener Voltage [V]":sgl, "Pump Zener Enable":bool, "Pump Zener Voltage [V]":sgl, "Boost Clamp [V]":sgl}
  T32 = typedef "DCM - UI.lvlib/Configuration.ctl" = cluster{"Configuration":T4, "Boost Voltage [V]":sgl, "Zener Enable":bool, "Zener Voltage [V]":sgl}
  T33 = typedef "DCM - UI.lvlib/Injector Configuration.ctl" = cluster{"Resistance [Ohm]":sgl, "Inductance [Henery]":sgl, "Capacitance [Farad]":sgl}
  T34 = typedef "DCM - UI.lvlib/System Configuration.ctl" = cluster{"Battery [V]":sgl, "Engine Speed [RPM]":sgl, "Rotations":u8, "Injector Configuration":T33, "Description":string}
  T35 = cluster{"DRVP [V]":sgl, "Primary A1A2 [V]":sgl, "Primary A3A4 [V]":sgl, "Secondary A1A2 [V]":sgl, "Secondary A3A4 [V]":sgl, "Ext HV A [V]":sgl, "DI Zener A [V]":sgl, "Pump Zener A [V]":sgl, "BoostClampV":sgl}
  T36 = typedef "LVStringsAndValuesArrayTypeDef_U8.ctl" = cluster{"String":string, "Value":u8}[]
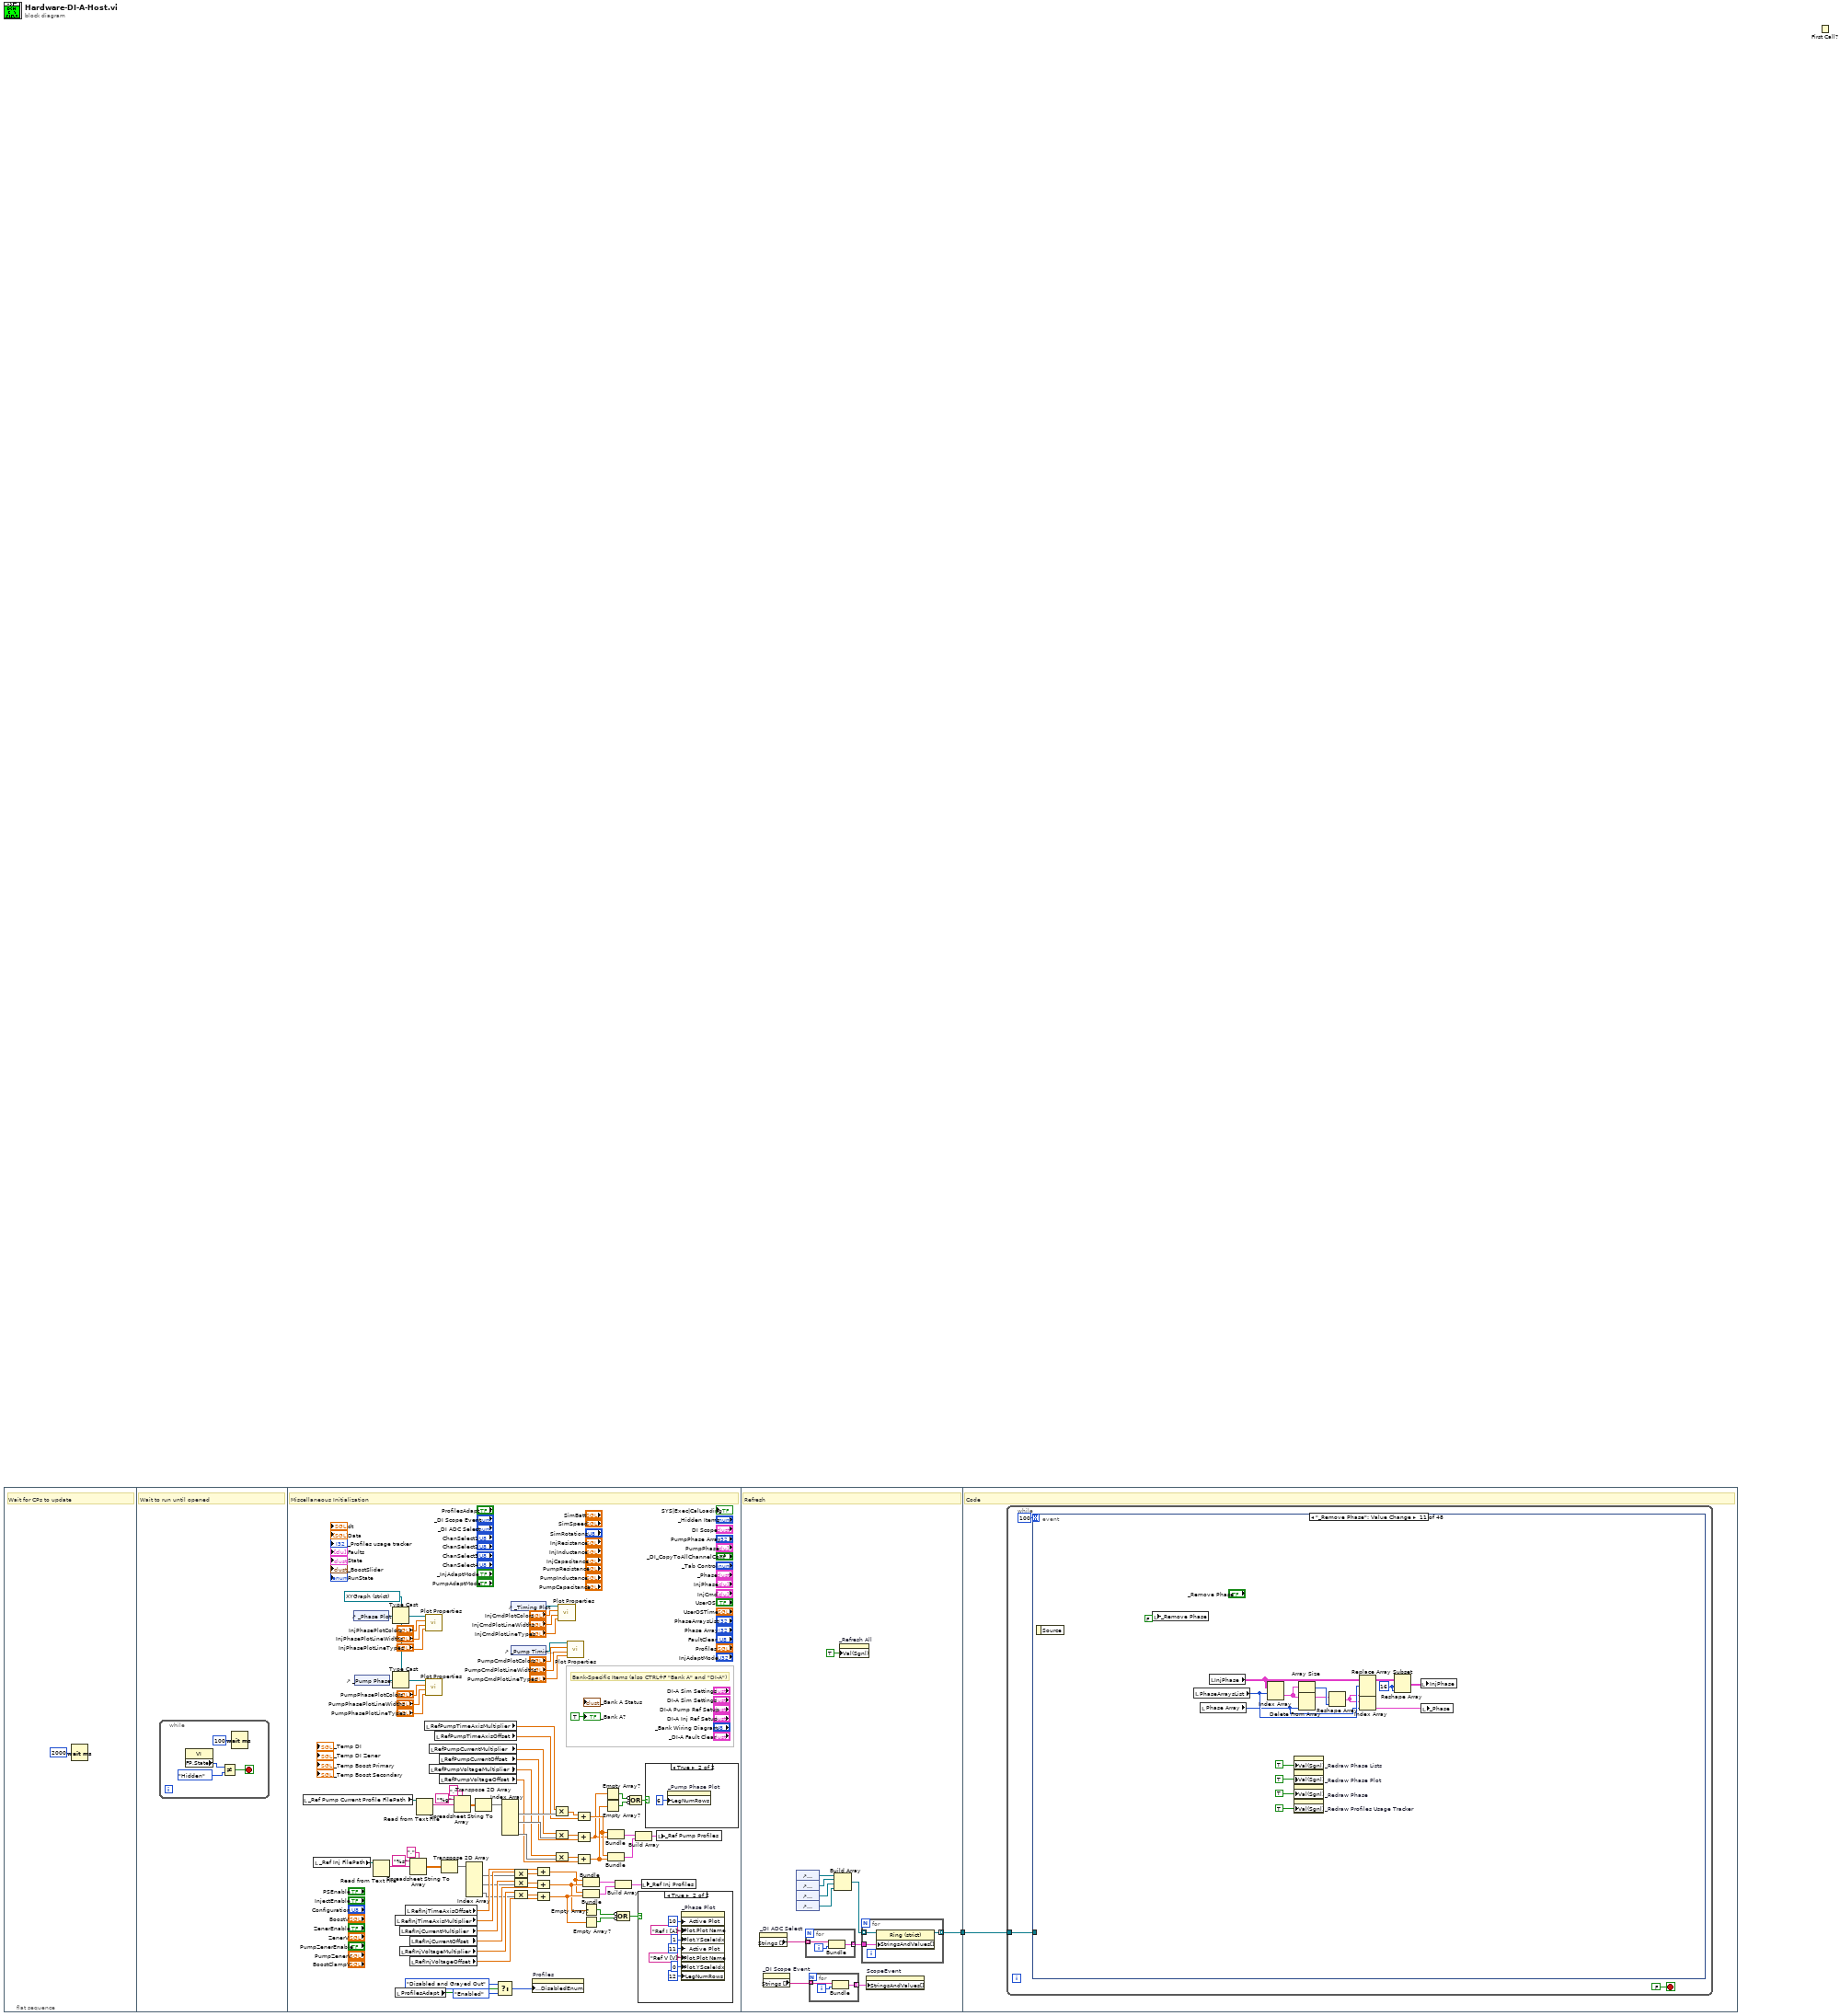
[diagram p0: block diagram]
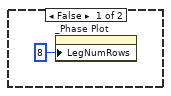
[diagram p2: hidden frame]
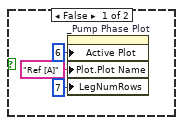
[diagram p3: hidden frame]
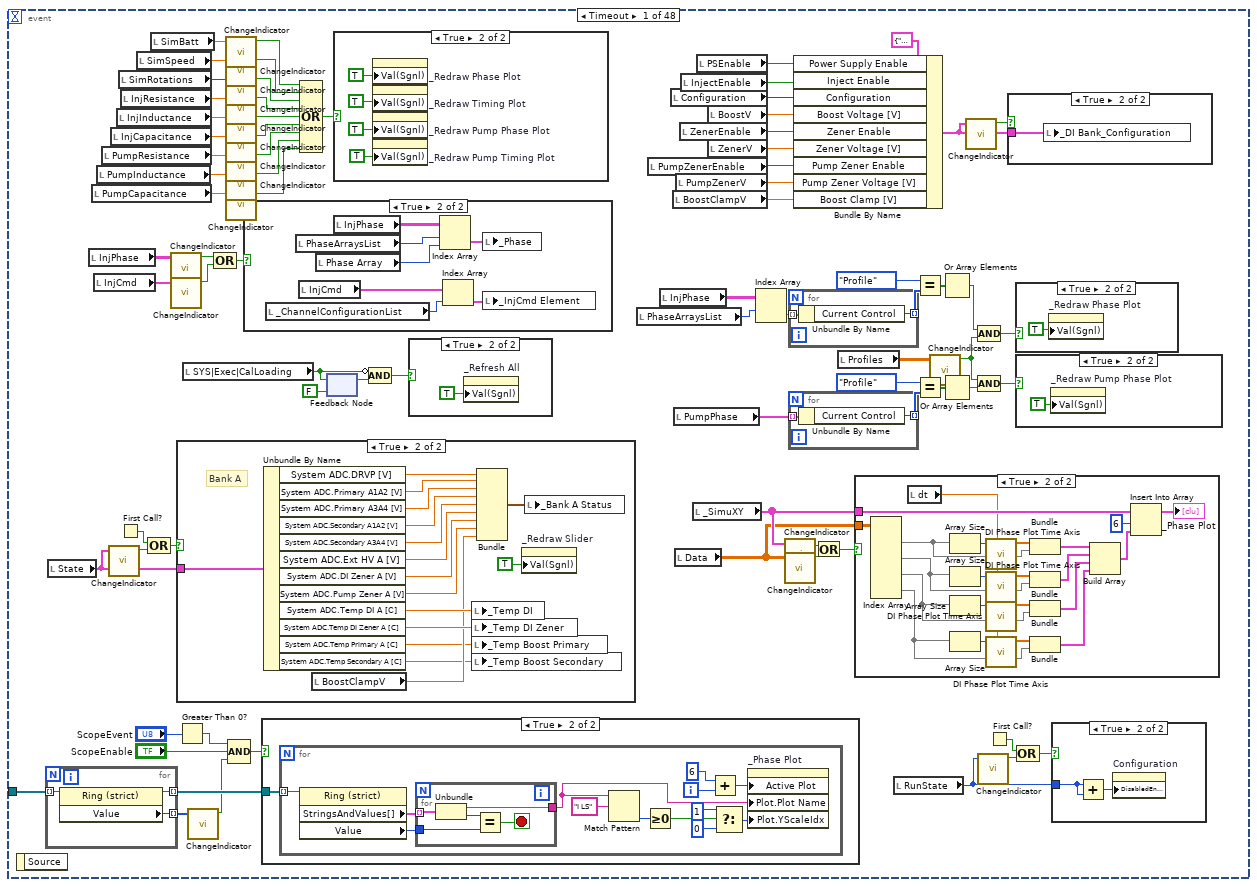
[diagram p4: hidden frame]
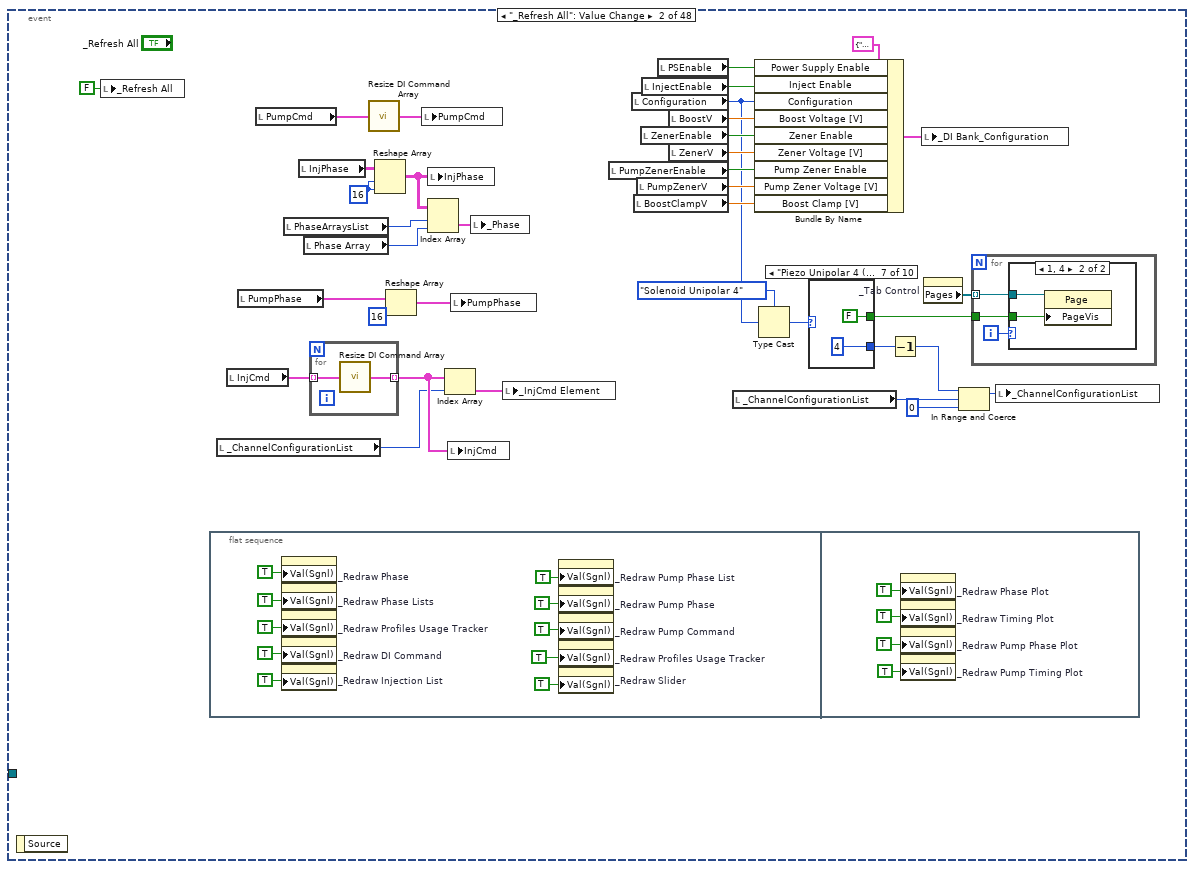
[diagram p15: hidden frame]
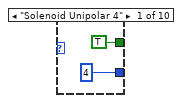
[diagram p16: hidden frame]
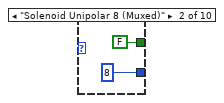
[diagram p17: hidden frame]
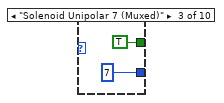
[diagram p18: hidden frame]
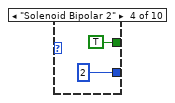
[diagram p19: hidden frame]
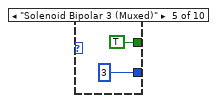
[diagram p20: hidden frame]
diagram:
  n1 = flat-sequence {
    tunnel: [w107] -> w1
    tunnel: w1 -> [w117]
    frame #0 {
      # "Wait for CPs to update"
      n2 = Wait (ms)(milliseconds to wait=u32 2000) -> ()  [unwired: 1 out]
    }
    frame #1 {
      # "Wait to run until opened"
      n3 = while {
        stop <- w4 stop-if-true
        n4 = property class="VI"() -> ("FP.State"=w5:T29)  [unwired: 2 in, 2 out]
        n5 = Not Equal?(x=w5, y=T29."Hidden" ("Front Panel Window:State")) -> (x != y?=w4:bool)
        n6 = Wait (ms)(milliseconds to wait=u32 100) -> ()  [unwired: 1 out]
      }
    }
    frame #2 {
      w13 = refnum<vi> refnum ("XYGraph in")
      # "Bank-Specific Items (also CTRL+F \"Bank A\" and \"DI-A\")"
      # "Miscellaneous Initialization"
      n7 = local read "_Ref Pump Current Profile FilePath"() -> (w53:path)
      n8 = local read "_Ref Inj FilePath"() -> (w19:path)
      n9 = control-ref of="_Phase Plot"() -> (w83:refnum<vi>)
      n10 = control-ref of="_Pump Phase Plot"() -> (w12:refnum<vi>)
      n11 = Read from Text File(file (use dialog)=w19) -> (text=w15:string)  [unwired: 3 in, 3 out]
      n12 = Type Cast(type=w13, x=w83) -> (*(type *) &x=w84:refnum<vi>)
      n13 = Type Cast(type=w13, x=w12) -> (*(type *) &x=w79:refnum<vi>)
      n14 = local read "RefInjTimeAxisMultiplier"() -> (w36:sgl)
      n15 = local read "ProfilesAdapt"() -> (w9:bool)
      n16 = local read "RefInjCurrentMultiplier"() -> (w37:sgl)
      n17 = local read "RefInjVoltageMultiplier"() -> (w39:sgl)
      n18 = local read "RefInjTimeAxisOffset"() -> (w35:sgl)
      n19 = local read "RefInjCurrentOffset"() -> (w38:sgl)
      n20 = local read "RefInjVoltageOffset"() -> (w40:sgl)
      n21 = Spreadsheet String To Array(delimiter (Tab)=",", format string="%s", spreadsheet string=w15) -> (array=w18:dbl[][])  [unwired: 1 in]
      n22 = Read from Text File(file (use dialog)=w53) -> (text=w57:string)  [unwired: 3 in, 3 out]
      n23 = local read "RefPumpTimeAxisMultiplier"() -> (w52:sgl)
      n24 = call "Plot Properties.vi"("LineTypes"="InjPhasePlotLineTypes", "LineWidths"="InjPhasePlotLineWidths", "PlotColors"="InjPhasePlotColors", "XYGraph in"=w84) -> ()  [unwired: 8 in]
      n25 = call "Plot Properties.vi"("LineTypes"="PumpPhasePlotLineTypes", "LineWidths"="PumpPhasePlotLineWidths", "PlotColors"="PumpPhasePlotColors", "XYGraph in"=w79) -> ()  [unwired: 8 in]
      n26 = local read "RefPumpCurrentMultiplier"() -> (w50:sgl)
      n27 = local read "RefPumpVoltageMultiplier"() -> (w48:sgl)
      n28 = local read "RefPumpTimeAxisOffset"() -> (w51:sgl)
      n29 = local read "RefPumpCurrentOffset"() -> (w49:sgl)
      n30 = local read "RefPumpVoltageOffset"() -> (w47:sgl)
      n31 = Transpose 2D Array(2D array=w18) -> (transposed array=w14:dbl[][])
      n32 = Spreadsheet String To Array(delimiter (Tab)=",", format string="%g", spreadsheet string=w57) -> (array=w54:dbl[][])  [unwired: 1 in]
      n33 = Index Array(array=w14) -> (element #1=w29:dbl[], element #2=w30:dbl[], element #3=w31:dbl[])  [unwired: 6 in]
      n34 = Transpose 2D Array(2D array=w54) -> (transposed array=w58:dbl[][])
      n35 = Select(t=T30."Disabled and Grayed Out" ("Disabled"), s=w9, f=T30."Enabled" ("Disabled")) -> (s? t:f=w8:T30)
      n36 = Index Array(array=w58) -> (element #1=w61:dbl[], element #2=w59:dbl[], element #3=w64:dbl[])  [unwired: 6 in]
      n37 = control-ref of="_Timing Plot"() -> (w75:refnum<vi>)
      n38 = control-ref of="_Pump Timing Plot"() -> (w68:refnum<vi>)
      n39 = Compound Arithmetic op=MULTIPLY(w36, w29) -> (w28:dbl[])
      n40 = Compound Arithmetic op=MULTIPLY(w37, w30) -> (w27:dbl[])
      n41 = Compound Arithmetic op=MULTIPLY(w39, w31) -> (w26:dbl[])
      n42 = property on="Profiles" class="Arr (strict)"("Array Element.DisabledEnum"=w8) -> ()  [unwired: 2 in, 2 out]
      n43 = Compound Arithmetic op=ADD(w35, w28) -> (w32:dbl[])
      n44 = Compound Arithmetic op=ADD(w27, w38) -> (w33:dbl[])
      n45 = Compound Arithmetic op=ADD(w26, w40) -> (w34:dbl[])
      n46 = Compound Arithmetic op=MULTIPLY(w52, w61) -> (w60:dbl[])
      n47 = Compound Arithmetic op=MULTIPLY(w50, w59) -> (w62:dbl[])
      n48 = Compound Arithmetic op=MULTIPLY(w48, w64) -> (w63:dbl[])
      n49 = call "Plot Properties.vi"("LineTypes"="InjCmdPlotLineTypes", "LineWidths"="InjCmdPlotLineWidths", "PlotColors"="InjCmdPlotColors", "XYGraph in"=w75) -> ()  [unwired: 8 in]
      n50 = call "Plot Properties.vi"("LineTypes"="PumpCmdPlotLineTypes", "LineWidths"="PumpCmdPlotLineWidths", "PlotColors"="PumpCmdPlotColors", "XYGraph in"=w68) -> ()  [unwired: 8 in]
      n51 = Compound Arithmetic op=ADD(w60, w51) -> (w65:dbl[])
      n52 = Compound Arithmetic op=ADD(w62, w49) -> (w41:dbl[])
      n53 = Compound Arithmetic op=ADD(w63, w47) -> (w42:dbl[])
      n54 = Bundle(w32, w33) -> (w20:cluster{dbl[], dbl[]})  [unwired: 1 in]
      n55 = Bundle(w32, w34) -> (w21:cluster{dbl[], dbl[]})  [unwired: 1 in]
      n56 = Empty Array?(array=w33) -> (empty?=w23:bool)
      n57 = Empty Array?(array=w34) -> (empty?=w24:bool)
      n58 = Empty Array?(array=w41) -> (empty?=w44:bool)
      n59 = Empty Array?(array=w42) -> (empty?=w45:bool)
      n60 = Bundle(w65, w41) -> (w66:cluster{dbl[], dbl[]})  [unwired: 1 in]
      n61 = Bundle(w65, w42) -> (w67:cluster{dbl[], dbl[]})  [unwired: 1 in]
      n62 = Build Array(w20, w21) -> (w22:cluster{dbl[], dbl[]}[])
      n63 = Compound Arithmetic op=OR(invert w23, invert w24) -> (w25:bool)
      n64 = Compound Arithmetic op=OR(invert w44, invert w45) -> (w43:bool)
      n65 = Build Array(w66, w67) -> (w46:cluster{dbl[], dbl[]}[])
      n66 = case shown="True" w25 {
        frame False {
          n67 = property on="_Phase Plot" class="XYGraph (strict)"("LegNumRows"=u32 8 ("Legend:Number of Rows")) -> ()  [unwired: 2 in, 2 out]
        }
        frame True {
          n68 = property on="_Phase Plot" class="XYGraph (strict)"("Active Plot"=u32 10, "Plot.Plot Name"="Ref I [A]", "Plot.YScaleIdx"=u32 1 ("Plot.Y Scale Index"), "Active Plot"=u32 11, "Plot.Plot Name"="Ref V [V]", "Plot.YScaleIdx"=u32 0 ("Plot.Y Scale Index"), "LegNumRows"=u32 12 ("Legend:Number of Rows")) -> ()  [unwired: 2 in, 2 out]
        }
      }
      n69 = local write "_Ref Inj Profiles"(w22) -> ()
      n70 = case shown="True" w43 {
        frame False {
          n71 = property on="_Pump Phase Plot" class="XYGraph (strict)"("Active Plot"=u32 6, "Plot.Plot Name"="Ref [A]", "LegNumRows"=u32 7 ("Legend:Number of Rows")) -> ()  [unwired: 2 in, 2 out]
        }
        frame True {
          n72 = property on="_Pump Phase Plot" class="XYGraph (strict)"("LegNumRows"=u32 6 ("Legend:Number of Rows")) -> ()  [unwired: 2 in, 2 out]
        }
      }
      n73 = local write "_Ref Pump Profiles"(w46) -> ()
      "_Bank A?" <- TRUE ("_Bank A?")
    }
    frame #3 {
      # "Refresh"
      n74 = property on="_DI ADC Select" class="Enum (strict)"() -> ("Strings []"=w106:string[])  [unwired: 2 in, 2 out]
      n75 = property on="_DI Scope Event" class="Enum (strict)"() -> ("Strings []"=w97:string[])  [unwired: 2 in, 2 out]
      n76 = control-ref of="ChanSelect1"() -> (w102:refnum<vi>)
      n77 = control-ref of="ChanSelect2"() -> (w103:refnum<vi>)
      n78 = control-ref of="ChanSelect3"() -> (w104:refnum<vi>)
      n79 = control-ref of="ChanSelect4"() -> (w105:refnum<vi>)
      n80 = for {
        tunnel: w106 -> [w116] mode=indexing
        tunnel: [w114] -> w100 mode=indexing
        i -> [w115]
        n81 = Bundle(w116, w115) -> (w114:cluster{string, i32})  [unwired: 1 in]
      }
      n82 = for {
        tunnel: w97 -> [w110] mode=indexing
        tunnel: [w108] -> w98 mode=indexing
        i -> [w109]
        n83 = Bundle(w110, w109) -> (w108:cluster{string, i32})  [unwired: 1 in]
      }
      n84 = Build Array(w102, w103, w104, w105) -> (w101:refnum<vi>[])
      n85 = property on="_Refresh All" class="Bool (strict)"("Val(Sgnl)"=TRUE ("Value (Signaling)")) -> ()  [unwired: 2 in, 2 out]
      n86 = for {
        tunnel: w101 -> [w113] mode=indexing
        tunnel: w100 -> [w112]
        tunnel: [w111] -> w107 mode=indexing
        n87 = property on="Property Node" class="Ring (strict)"(reference=w113, "StringsAndValues[]"=w112) -> (reference out=w111:refnum<vi>)  [unwired: 1 in, 1 out]
      }
      n88 = property on="ScopeEvent" class="Ring (strict)"("StringsAndValues[]"=w98) -> ()  [unwired: 2 in, 2 out]
    }
    frame #4 {
      # "Code"
      n89 = while {
        tunnel: w117 -> [w118]
        stop <- FALSE stop-if-true
        n90 = event shown="[10] \"_Remove Phase\": Value Change" {
          selector: _ -> [_ _ _ _ _ _ _ _ _ _ _ _ _ _ _ _ _ _ _ _ _ _ _ _ _ _ _ _ _ _ _ _ _ _ _ _ _ _ _ _ _ _ _ _ _ _ _ _]
          dyn-events: _ -> [_ _ _ _ _ _ _ _ _ _ _ _ _ _ _ _ _ _ _ _ _ _ _ _ _ _ _ _ _ _ _ _ _ _ _ _ _ _ _ _ _ _ _ _ _ _ _ _]
          timeout: 100 -> [_ _ _ _ _ _ _ _ _ _ _ _ _ _ _ _ _ _ _ _ _ _ _ _ _ _ _ _ _ _ _ _ _ _ _ _ _ _ _ _ _ _ _ _ _ _ _ _]
          tunnel: w118 -> [w171 _ _ _ _ _ _ _ _ _ _ _ _ _ _ _ _ _ _ _ _ _ _ _ _ _ _ _ _ _ _ _ _ _ _ _ _ _ _ _ _ _ _ _ _ _ _ _]
          event Timeout {
            n91 = event-data() -> ()  [unwired: 1 in, 1 out]
            n92 = for {
              tunnel: w171 -> [w231] mode=indexing
              tunnel: [w230] -> w172 mode=indexing
              tunnel: [w229] -> w170 mode=indexing
              n93 = property on="Property Node" class="Ring (strict)"(reference=w231) -> (reference out=w230:refnum<vi>, "Value"=w229:u8)  [unwired: 1 in, 1 out]
            }
            n94 = local read "State"() -> (w140:T19)
            n95 = local read "InjPhase"() -> (w135:T17)
            n96 = local read "PumpCapacitance"() -> (w151:sgl)
            n97 = local read "InjCmd"() -> (w134:T6)
            n98 = local read "PumpInductance"() -> (w158:sgl)
            n99 = local read "PumpResistance"() -> (w157:sgl)
            n100 = call "ChangeIndicator.vi"("Input"=w140) -> ("Change"=w130:bool)  [unwired: 9 in]
            n101 = local read "InjCapacitance"() -> (w156:sgl)
            n102 = First Call?() -> (First Call?: T/F=w128:bool)
            n103 = local read "InjInductance"() -> (w155:sgl)
            n104 = local read "SimRotations"() -> (w153:u8)
            n105 = local read "InjResistance"() -> (w154:sgl)
            n106 = local read "SimSpeed"() -> (w152:sgl)
            n107 = Compound Arithmetic op=OR(w128, w130) -> (w129:bool)
            n108 = local read "SimBatt"() -> (w150:sgl)
            n109 = call "ChangeIndicator.vi"("Input"=w135) -> ("Change"=w133:bool)  [unwired: 9 in]
            n110 = call "ChangeIndicator.vi"("Input"=w134) -> ("Change"=w132:bool)  [unwired: 9 in]
            n111 = case shown="True" w129 {
              tunnel: w140 -> [_ w217]
              frame False {
              }
              frame True {
                # "Bank A"
                n112 = Unbundle By Name(w217) -> ("System ADC.DRVP [V]"=w228:sgl, "System ADC.Primary A1A2 [V]"=w227:sgl, "System ADC.Primary A3A4 [V]"=w226:sgl, "System ADC.Secondary A1A2 [V]"=w225:sgl, "System ADC.Secondary A3A4 [V]"=w224:sgl, "System ADC.Ext HV A [V]"=w223:sgl, "System ADC.DI Zener A [V]"=w222:sgl, "System ADC.Pump Zener A [V]"=w221:sgl, "System ADC.Temp DI A [C]"=w219:sgl, "System ADC.Temp DI Zener A [C]"=w218:sgl, "System ADC.Temp Primary A [C]"=w213:sgl, "System ADC.Temp Secondary A [C]"=w214:sgl)
                n113 = local read "BoostClampV"() -> (w215:sgl)
                n114 = local write "_Temp DI"(w219) -> ()
                n115 = local write "_Temp DI Zener"(w218) -> ()
                n116 = local write "_Temp Boost Primary"(w213) -> ()
                n117 = local write "_Temp Boost Secondary"(w214) -> ()
                n118 = Bundle("DRVP [V]"=w228, "Primary A1A2 [V]"=w227, "Primary A3A4 [V]"=w226, "Secondary A1A2 [V]"=w225, "Secondary A3A4 [V]"=w224, "Ext HV A [V]"=w223, "DI Zener A [V]"=w222, "Pump Zener A [V]"=w221, "BoostClampV"=w215) -> (w220:T35)  [unwired: 1 in]
                n119 = property on="_Redraw Slider" class="Bool (strict)"("Val(Sgnl)"=TRUE ("Value (Signaling)")) -> ()  [unwired: 2 in, 2 out]
                n120 = local write "_Bank A Status"(w220) -> ()
              }
            }
            n121 = Greater Than 0?(x="ScopeEvent") -> (x > 0?=w196:bool)
            n122 = local read "SYS|Exec|CalLoading"() -> (w138:bool)
            n123 = call "ChangeIndicator.vi"("Input"=w170) -> ("Change"=w169:bool)  [unwired: 9 in]
            n124 = Compound Arithmetic op=OR(w133, w132) -> (w131:bool)
            n125 = call "ChangeIndicator.vi"("Input"=w150) -> ("Change"=w159:bool)  [unwired: 9 in]
            n126 = call "ChangeIndicator.vi"("Input"=w152) -> ("Change"=w160:bool)  [unwired: 9 in]
            n127 = call "ChangeIndicator.vi"("Input"=w153) -> ("Change"=w161:bool)  [unwired: 9 in]
            n128 = call "ChangeIndicator.vi"("Input"=w154) -> ("Change"=w162:bool)  [unwired: 9 in]
            n129 = call "ChangeIndicator.vi"("Input"=w155) -> ("Change"=w163:bool)  [unwired: 9 in]
            n130 = call "ChangeIndicator.vi"("Input"=w156) -> ("Change"=w164:bool)  [unwired: 9 in]
            n131 = call "ChangeIndicator.vi"("Input"=w157) -> ("Change"=w165:bool)  [unwired: 9 in]
            n132 = call "ChangeIndicator.vi"("Input"=w158) -> ("Change"=w166:bool)  [unwired: 9 in]
            n133 = call "ChangeIndicator.vi"("Input"=w151) -> ("Change"=w167:bool)  [unwired: 9 in]
            n134 = Compound Arithmetic op=AND(w196, "ScopeEnable", w169) -> (w194:bool)
            n135 = case shown="True" w131 {
              frame False {
              }
              frame True {
                n136 = local read "_ChannelConfigurationList"() -> (w205:i32)
                n137 = local read "PhaseArraysList"() -> (w201:i32)
                n138 = local read "InjCmd"() -> (w204:T6)
                n139 = local read "Phase Array"() -> (w200:i32)
                n140 = local read "InjPhase"() -> (w206:T17)
                n141 = Index Array(array=w206, index (row)=w201, index (col)=w200) -> (element=w202:T13)
                n142 = Index Array(array=w204, index=w205) -> (element=w203:T7)
                n143 = local write "_Phase"(w202) -> ()
                n144 = local write "_InjCmd Element"(w203) -> ()
              }
            }
            n145 = case shown="True" w194 {
              tunnel: w172 -> [_ w260]
              frame False {
              }
              frame True {
                n146 = for {
                  tunnel: w260 -> [w261] mode=indexing
                  i -> [w264]
                  n147 = property on="Property Node" class="Ring (strict)"(reference=w261) -> ("StringsAndValues[]"=w267:T36, "Value"=w268:u8)  [unwired: 1 in, 2 out]
                  n148 = for {
                    tunnel: w267 -> [w278] mode=indexing
                    tunnel: [w275] -> w271
                    tunnel: w268 -> [w274]
                    stop <- w276 stop-if-true
                    n149 = Unbundle(w278) -> ("String"=w275:string, "Value"=w277:u8)
                    n150 = Equal?(x=w277, y=w274) -> (x = y?=w276:bool)
                  }
                  n151 = Match Pattern(string=w271, regular expression="I LS") -> (offset past match=w270:i32)  [unwired: 1 in, 3 out]
                  n152 = Greater Or Equal To 0?(x=w270) -> (x >= 0?=w265:bool)
                  n153 = Add(x=u32 6 ("Active Plot"), y=w264) -> (x+y=w262:u32)
                  n154 = Select(t=u32 1 ("Active Y Scale"), s=w265, f=u32 0 ("Active Y Scale")) -> (s? t:f=w273:u32)
                  n155 = property on="_Phase Plot" class="XYGraph (strict)"("Active Plot"=w262, "Plot.Plot Name"=w271, "Plot.YScaleIdx"=w273) -> ()  [unwired: 2 in, 2 out]
                }
              }
            }
            n156 = Compound Arithmetic op=OR(w159, w160, w161, w162, w163, w164, w165, w166, w167) -> (w168:bool)
            n157 = feedback-in #1(w138) -> ()
            n158 = feedback #1(FALSE ("SYS|Exec|CalLoading")) -> (w139:bool)
            n159 = case shown="True" w168 {
              frame False {
              }
              frame True {
                n160 = property on="_Redraw Phase Plot" class="Bool (strict)"("Val(Sgnl)"=TRUE ("Value (Signaling)")) -> ()  [unwired: 2 in, 2 out]
                n161 = property on="_Redraw Timing Plot" class="Bool (strict)"("Val(Sgnl)"=TRUE ("Value (Signaling)")) -> ()  [unwired: 2 in, 2 out]
                n162 = property on="_Redraw Pump Phase Plot" class="Bool (strict)"("Val(Sgnl)"=TRUE ("Value (Signaling)")) -> ()  [unwired: 2 in, 2 out]
                n163 = property on="_Redraw Pump Timing Plot" class="Bool (strict)"("Val(Sgnl)"=TRUE ("Value (Signaling)")) -> ()  [unwired: 2 in, 2 out]
              }
            }
            n164 = Compound Arithmetic op=AND(invert w138, w139) -> (w136:bool)
            n165 = case shown="True" w136 {
              frame False {
              }
              frame True {
                n166 = property on="_Refresh All" class="Bool (strict)"("Val(Sgnl)"=TRUE ("Value (Signaling)")) -> ()  [unwired: 2 in, 2 out]
              }
            }
            n167 = local read "PhaseArraysList"() -> (w178:i32)
            n168 = local read "PumpZenerEnable"() -> (w126:bool)
            n169 = local read "InjPhase"() -> (w179:T17)
            n170 = local read "Configuration"() -> (w146:u8)
            n171 = local read "BoostClampV"() -> (w142:sgl)
            n172 = local read "PumpPhase"() -> (w186:T12)
            n173 = local read "Data"() -> (w192:sgl[][])
            n174 = local read "PumpZenerV"() -> (w143:sgl)
            n175 = local read "ZenerEnable"() -> (w144:bool)
            n176 = local read "InjectEnable"() -> (w147:bool)
            n177 = local read "_SimuXY"() -> (w193:cluster{"Array":dbl[], "Array":dbl[]}[])
            n178 = local read "PSEnable"() -> (w148:bool)
            n179 = local read "BoostV"() -> (w145:sgl)
            n180 = local read "ZenerV"() -> (w141:sgl)
            n181 = Index Array(array=w179, index (row)=w178) -> (element=w177:T13[])  [unwired: 1 in]
            n182 = call "ChangeIndicator.vi"("Input"=w193) -> ("Change"=w190:bool)  [unwired: 9 in]
            n183 = call "ChangeIndicator.vi"("Input"=w192) -> ("Change"=w191:bool)  [unwired: 9 in]
            n184 = for {
              tunnel: [w237] -> w175 mode=indexing
              tunnel: w177 -> [w236] mode=indexing
              n185 = Unbundle By Name(w236) -> ("Current Control"=w237:T16)
            }
            n186 = for {
              tunnel: [w234] -> w184 mode=indexing
              tunnel: w186 -> [w233] mode=indexing
              n187 = Unbundle By Name(w233) -> ("Current Control"=w234:T16)
            }
            n188 = Bundle By Name(cluster=T31 {"Configuration"=enum."Solenoid Unipolar 4", "Power Supply Enable"=FALSE, "Boost Voltage [V]"=0.0, "Inject Enable"=FALSE, "Zener Enable"=FALSE, "Zener Voltage [V]"=0.0, "Pump Zener Enable"=FALSE, "Pump Zener Voltage [V]"=0.0, "Boost Clamp [V]"=0.0} ("_DI Bank_Configuration"), "Power Supply Enable"=w148, "Inject Enable"=w147, "Configuration"=w146, "Boost Voltage [V]"=w145, "Zener Enable"=w144, "Zener Voltage [V]"=w141, "Pump Zener Enable"=w126, "Pump Zener Voltage [V]"=w143, "Boost Clamp [V]"=w142) -> (w149:T31)
            n189 = Or(x=w190, y=w191) -> (x .or. y?=w189:bool)
            n190 = local read "Profiles"() -> (w176:sgl[][])
            n191 = case shown="True" w189 {
              tunnel: w193 -> [_ w253]
              tunnel: w192 -> [_ w252]
              frame False {
              }
              frame True {
                n192 = Index Array(array=w252) -> (element #1=w239:sgl[], element #2=w251:sgl[], element #3=w245:sgl[], element #4=w242:sgl[])  [unwired: 8 in]
                n193 = local read "dt"() -> (w238:sgl)
                n194 = Array Size(array=w239) -> (size(s)=w259:i32)
                n195 = Array Size(array=w251) -> (size(s)=w250:i32)
                n196 = Array Size(array=w245) -> (size(s)=w248:i32)
                n197 = Array Size(array=w242) -> (size(s)=w244:i32)
                n198 = call "DI Phase Plot Time Axis.vi"("dt"=w238, "Array Size"=w259) -> ("Array"=w258:dbl[])  [unwired: 9 in]
                n199 = call "DI Phase Plot Time Axis.vi"("dt"=w238, "Array Size"=w250) -> ("Array"=w249:dbl[])  [unwired: 9 in]
                n200 = call "DI Phase Plot Time Axis.vi"("dt"=w238, "Array Size"=w248) -> ("Array"=w246:dbl[])  [unwired: 9 in]
                n201 = call "DI Phase Plot Time Axis.vi"("dt"=w238, "Array Size"=w244) -> ("Array"=w243:dbl[])  [unwired: 9 in]
                n202 = Bundle("Array"=w258, "Data"=w239) -> (w254:cluster{"Array":dbl[], "Data":sgl[]})  [unwired: 1 in]
                n203 = Bundle("Array"=w249, "Data"=w251) -> (w247:cluster{"Array":dbl[], "Data":sgl[]})  [unwired: 1 in]
                n204 = Bundle("Array"=w246, "Data"=w245) -> (w241:cluster{"Array":dbl[], "Data":sgl[]})  [unwired: 1 in]
                n205 = Bundle("Array"=w243, "Data"=w242) -> (w240:cluster{"Array":dbl[], "Data":sgl[]})  [unwired: 1 in]
                n206 = Build Array(w254, w247, w241, w240) -> (w256:cluster{"Array":dbl[], "Data":sgl[]}[])
                n207 = Insert Into Array(array=w253, index=6, new element=w256) -> (→"_Phase Plot":cluster{"Array":dbl[], "Array":dbl[]}[])
              }
            }
            n208 = local read "RunState"() -> (w122:T1)
            n209 = Equal?(x=Control."Profile" ("Control"), y=w175) -> (x = y?=w174:bool[])
            n210 = Equal?(x=Control."Profile" ("Control"), y=w184) -> (x = y?=w185:bool[])
            n211 = call "ChangeIndicator.vi"("Input"=w176) -> ("Change"=w188:bool)  [unwired: 9 in]
            n212 = Or Array Elements(Boolean array=w174) -> (logical OR=w173:bool)
            n213 = Or Array Elements(Boolean array=w185) -> (logical OR=w187:bool)
            n214 = call "ChangeIndicator.vi"("Input"=w149) -> ("Change"=w121:bool)  [unwired: 9 in]
            n215 = Compound Arithmetic op=AND(w173, w188) -> (w181:bool)
            n216 = Compound Arithmetic op=AND(w188, w187) -> (w182:bool)
            n217 = call "ChangeIndicator.vi"("Input"=w122) -> ("Change"=w124:bool)  [unwired: 9 in]
            n218 = First Call?() -> (First Call?: T/F=w125:bool)
            n219 = case shown="True" w121 {
              tunnel: w149 -> [_ w208]
              frame False {
              }
              frame True {
                n220 = local write "_DI Bank_Configuration"(w208) -> ()
              }
            }
            n221 = case shown="True" w181 {
              frame False {
              }
              frame True {
                n222 = property on="_Redraw Phase Plot" class="Bool (strict)"("Val(Sgnl)"=TRUE ("Value (Signaling)")) -> ()  [unwired: 2 in, 2 out]
              }
            }
            n223 = case shown="True" w182 {
              frame False {
              }
              frame True {
                n224 = property on="_Redraw Pump Phase Plot" class="Bool (strict)"("Val(Sgnl)"=TRUE ("Value (Signaling)")) -> ()  [unwired: 2 in, 2 out]
              }
            }
            n225 = Compound Arithmetic op=OR(w125, w124) -> (w123:bool)
            n226 = case shown="True" w123 {
              tunnel: w122 -> [_ w199]
              frame False {
              }
              frame True {
                n227 = Add(x=w199, y=w199) -> (x+y=w198:u8)
                n228 = property on="Configuration" class="Enum (strict)"("DisabledEnum"=w198) -> ()  [unwired: 2 in, 2 out]
              }
            }
          }
          event "_Refresh All": Value Change {
            w304 = 16 ("dimension size")
            n229 = event-data() -> ()  [unwired: 1 in, 1 out]
            n230 = local write "_Refresh All"(FALSE ("_Refresh All")) -> ()
            n231 = flat-sequence {
              frame #0 {
                n232 = property on="_Redraw Phase" class="Bool (strict)"("Val(Sgnl)"=TRUE ("Value (Signaling)")) -> ()  [unwired: 2 in, 2 out]
                n233 = property on="_Redraw Phase Lists" class="Bool (strict)"("Val(Sgnl)"=TRUE ("Value (Signaling)")) -> ()  [unwired: 2 in, 2 out]
                n234 = property on="_Redraw Profiles Usage Tracker" class="Bool (strict)"("Val(Sgnl)"=TRUE ("Value (Signaling)")) -> ()  [unwired: 2 in, 2 out]
                n235 = property on="_Redraw DI Command" class="Bool (strict)"("Val(Sgnl)"=TRUE ("Value (Signaling)")) -> ()  [unwired: 2 in, 2 out]
                n236 = property on="_Redraw Injection List" class="Bool (strict)"("Val(Sgnl)"=TRUE ("Value (Signaling)")) -> ()  [unwired: 2 in, 2 out]
                n237 = property on="_Redraw Pump Phase List" class="Bool (strict)"("Val(Sgnl)"=TRUE ("Value (Signaling)")) -> ()  [unwired: 2 in, 2 out]
                n238 = property on="_Redraw Pump Phase" class="Bool (strict)"("Val(Sgnl)"=TRUE ("Value (Signaling)")) -> ()  [unwired: 2 in, 2 out]
                n239 = property on="_Redraw Pump Command" class="Bool (strict)"("Val(Sgnl)"=TRUE ("Value (Signaling)")) -> ()  [unwired: 2 in, 2 out]
                n240 = property on="_Redraw Profiles Usage Tracker" class="Bool (strict)"("Val(Sgnl)"=TRUE ("Value (Signaling)")) -> ()  [unwired: 2 in, 2 out]
                n241 = property on="_Redraw Slider" class="Bool (strict)"("Val(Sgnl)"=TRUE ("Value (Signaling)")) -> ()  [unwired: 2 in, 2 out]
              }
              frame #1 {
                n242 = property on="_Redraw Phase Plot" class="Bool (strict)"("Val(Sgnl)"=TRUE ("Value (Signaling)")) -> ()  [unwired: 2 in, 2 out]
                n243 = property on="_Redraw Timing Plot" class="Bool (strict)"("Val(Sgnl)"=TRUE ("Value (Signaling)")) -> ()  [unwired: 2 in, 2 out]
                n244 = property on="_Redraw Pump Phase Plot" class="Bool (strict)"("Val(Sgnl)"=TRUE ("Value (Signaling)")) -> ()  [unwired: 2 in, 2 out]
                n245 = property on="_Redraw Pump Timing Plot" class="Bool (strict)"("Val(Sgnl)"=TRUE ("Value (Signaling)")) -> ()  [unwired: 2 in, 2 out]
              }
            }
            n246 = local read "_ChannelConfigurationList"() -> (w303:i32)
            n247 = local read "InjCmd"() -> (w309:T6)
            n248 = local read "PumpPhase"() -> (w311:T12)
            n249 = local read "PumpCmd"() -> (w312:T26)
            n250 = local read "PhaseArraysList"() -> (w301:i32)
            n251 = local read "InjPhase"() -> (w310:T17)
            n252 = local read "Phase Array"() -> (w300:i32)
            n253 = for {
              tunnel: [w355] -> w308 mode=indexing
              tunnel: w309 -> [w354] mode=indexing
              n254 = call "Resize DI Command Array.vi"("Command in"=w354) -> ("Command out"=w355:T7)
            }
            n255 = call "Resize DI Command Array.vi"("Command in"=w312) -> ("Command out"=w313:T7)
            n256 = Reshape Array(w310, w304, w304) -> (w299:T17)
            n257 = Reshape Array(w311, 16 ("dimension size")) -> (w305:T12)
            n258 = local write "PumpCmd"(w313) -> ()
            n259 = local write "InjPhase"(w299) -> ()
            n260 = Index Array(array=w299, index (row)=w301, index (col)=w300) -> (element=w302:T13)
            n261 = Index Array(array=w308, index=w303) -> (element=w307:T7)
            n262 = local write "InjCmd"(w308) -> ()
            n263 = local write "PumpPhase"(w305) -> ()
            n264 = local write "_Phase"(w302) -> ()
            n265 = local write "_InjCmd Element"(w307) -> ()
            n266 = local read "PumpZenerEnable"() -> (w280:bool)
            n267 = local read "Configuration"() -> (w279:u8)
            n268 = local read "BoostClampV"() -> (w283:sgl)
            n269 = local read "PumpZenerV"() -> (w284:sgl)
            n270 = local read "ZenerEnable"() -> (w285:bool)
            n271 = local read "InjectEnable"() -> (w287:bool)
            n272 = local read "PSEnable"() -> (w288:bool)
            n273 = local read "BoostV"() -> (w286:sgl)
            n274 = local read "ZenerV"() -> (w282:sgl)
            n275 = local read "_ChannelConfigurationList"() -> (w293:i32)
            n276 = Bundle By Name(cluster=T31 {"Configuration"=enum."Solenoid Unipolar 4", "Power Supply Enable"=FALSE, "Boost Voltage [V]"=0.0, "Inject Enable"=FALSE, "Zener Enable"=FALSE, "Zener Voltage [V]"=0.0, "Pump Zener Enable"=FALSE, "Pump Zener Voltage [V]"=0.0, "Boost Clamp [V]"=0.0} ("_DI Bank_Configuration"), "Power Supply Enable"=w288, "Inject Enable"=w287, "Configuration"=w279, "Boost Voltage [V]"=w286, "Zener Enable"=w285, "Zener Voltage [V]"=w282, "Pump Zener Enable"=w280, "Pump Zener Voltage [V]"=w284, "Boost Clamp [V]"=w283) -> (w289:T31)
            n277 = Type Cast(type=DI_-_Bank_Configuration."Solenoid Unipolar 4" ("Configuration"), x=w279) -> (*(type *) &x=w291:T4)
            n278 = case shown="\"Piezo Unipolar 4 (Muxed)\"" w291 {
              tunnel: [4 8 7 2 3 2 4 3 2 3] -> w296
              tunnel: [TRUE ("Value (Signaling)") FALSE ("Value (Signaling)") TRUE ("Value (Signaling)") TRUE ("Value (Signaling)") TRUE ("Value (Signaling)") TRUE ("Value (Signaling)") FALSE ("Value (Signaling)") TRUE ("Value (Signaling)") TRUE ("Value (Signaling)") TRUE ("Value (Signaling)")] -> w290
              frame "Solenoid Unipolar 4" {
              }
              frame "Solenoid Unipolar 8 (Muxed)" {
              }
              frame "Solenoid Unipolar 7 (Muxed)" {
              }
              frame "Solenoid Bipolar 2" {
              }
              frame "Solenoid Bipolar 3 (Muxed)" {
              }
              frame "Piezo Unipolar 2" {
              }
              frame "Piezo Unipolar 4 (Muxed)" {
              }
              frame "Piezo Unipolar 3 (Muxed)" {
              }
              frame "Piezo Bipolar 2" {
              }
              frame "Piezo Bipolar 3 (Muxed)" {
              }
            }
            n279 = Decrement(x=w296) -> (x-1=w294:i32)
            n280 = local write "_DI Bank_Configuration"(w289) -> ()
            n281 = property on="_Tab Control" class="TabCtl (strict)"() -> ("Pages"=w297:refnum<vi>[])  [unwired: 2 in, 2 out]
            n282 = In Range and Coerce(upper limit=w294, x=w293, lower limit=0) -> (coerced(x)=w292:i32)  [unwired: 1 out]
            n283 = for {
              tunnel: w297 -> [w337] mode=indexing
              tunnel: w290 -> [w335]
              i -> [w336]
              n284 = case shown="1, 4" w336 {
                tunnel: w337 -> [_ w339]
                tunnel: w335 -> [_ w338]
                frame 0, Default {
                }
                frame 1, 4 {
                  n285 = property class="Page"(reference=w339, "PageVis"=w338) -> ()  [unwired: 1 in, 2 out]
                }
              }
            }
            n286 = local write "_ChannelConfigurationList"(w292) -> ()
          }
          event "PhaseArraysList": Value Change {
            n287 = event-data() -> ()  [unwired: 1 in, 1 out]
            n288 = local read "PhaseArraysList"() -> (w357:i32)
            n289 = local read "Phase Array"() -> (w356:i32)
            n290 = local read "InjPhase"() -> (w358:T17)
            n291 = property on="_Redraw Phase Lists" class="Bool (strict)"("Val(Sgnl)"=TRUE ("Value (Signaling)")) -> ()  [unwired: 2 in, 2 out]
            n292 = property on="_Redraw Phase Plot" class="Bool (strict)"("Val(Sgnl)"=TRUE ("Value (Signaling)")) -> ()  [unwired: 2 in, 2 out]
            n293 = property on="_Redraw Phase" class="Bool (strict)"("Val(Sgnl)"=TRUE ("Value (Signaling)")) -> ()  [unwired: 2 in, 2 out]
            n294 = Index Array(array=w358, index (row)=w357, index (col)=w356) -> (element=w359:T13)
            n295 = local write "_Phase"(w359) -> ()
          }
          event "_MovePhaseArrayListDown": Value Change {
            n296 = event-data() -> ()  [unwired: 1 in, 6 out]
            n297 = local read "PhaseArraysList"() -> (w370:i32)
            n298 = local read "InjPhase"() -> (w373:T17)
            n299 = property on="_Redraw Phase Lists" class="Bool (strict)"("Val(Sgnl)"=TRUE ("Value (Signaling)")) -> ()  [unwired: 2 in, 2 out]
            n300 = property on="_Redraw Phase Plot" class="Bool (strict)"("Val(Sgnl)"=TRUE ("Value (Signaling)")) -> ()  [unwired: 2 in, 2 out]
            n301 = property on="_Redraw Phase" class="Bool (strict)"("Val(Sgnl)"=TRUE ("Value (Signaling)")) -> ()  [unwired: 2 in, 2 out]
            n302 = Delete From Array(array=w373, index (row)=w370) -> (deleted portion=w371:T13[], array with subset deleted=w372:T17)  [unwired: 2 in]
            n303 = Increment(x=w370) -> (x+1=w365:i32)
            n304 = local write "_MovePhaseArrayListDown"(FALSE ("_MovePhaseArrayListDown")) -> ()
            n305 = In Range and Coerce(upper limit=15, x=w365, lower limit=0) -> (coerced(x)=w364:i32)  [unwired: 1 out]
            n306 = local write "PhaseArraysList"(w364) -> ()
            n307 = local read "Phase Array"() -> (w369:i32)
            n308 = Insert Into Array(array=w372, index (row)=w364, new element=w371) -> (w363:T17)  [unwired: 1 in]
            n309 = local write "InjPhase"(w363) -> ()
            n310 = Index Array(array=w363, index (row)=w364, index (col)=w369) -> (element=w368:T13)
            n311 = local write "_Phase"(w368) -> ()
          }
          event "_MovePhaseArrayListUp": Value Change {
            n312 = event-data() -> ()  [unwired: 1 in, 6 out]
            n313 = local read "PhaseArraysList"() -> (w386:i32)
            n314 = local read "InjPhase"() -> (w389:T17)
            n315 = property on="_Redraw Phase Lists" class="Bool (strict)"("Val(Sgnl)"=TRUE ("Value (Signaling)")) -> ()  [unwired: 2 in, 2 out]
            n316 = property on="_Redraw Phase Plot" class="Bool (strict)"("Val(Sgnl)"=TRUE ("Value (Signaling)")) -> ()  [unwired: 2 in, 2 out]
            n317 = property on="_Redraw Phase" class="Bool (strict)"("Val(Sgnl)"=TRUE ("Value (Signaling)")) -> ()  [unwired: 2 in, 2 out]
            n318 = Delete From Array(array=w389, index (row)=w386) -> (deleted portion=w387:T13[], array with subset deleted=w388:T17)  [unwired: 2 in]
            n319 = Decrement(x=w386) -> (x-1=w381:i32)
            n320 = In Range and Coerce(upper limit=15, x=w381, lower limit=0) -> (coerced(x)=w380:i32)  [unwired: 1 out]
            n321 = local write "_MovePhaseArrayListUp"(FALSE ("_MovePhaseArrayListUp")) -> ()
            n322 = local write "PhaseArraysList"(w380) -> ()
            n323 = local read "Phase Array"() -> (w385:i32)
            n324 = Insert Into Array(array=w388, index (row)=w380, new element=w387) -> (w378:T17)  [unwired: 1 in]
            n325 = local write "InjPhase"(w378) -> ()
            n326 = Index Array(array=w378, index (row)=w380, index (col)=w385) -> (element=w384:T13)
            n327 = local write "_Phase"(w384) -> ()
          }
          event "Phase Array": Value Change {
            n328 = event-data() -> ()  [unwired: 1 in, 1 out]
            n329 = local read "PhaseArraysList"() -> (w394:i32)
            n330 = local read "Phase Array"() -> (w393:i32)
            n331 = local read "InjPhase"() -> (w395:T17)
            n332 = property on="_Redraw Phase" class="Bool (strict)"("Val(Sgnl)"=TRUE ("Value (Signaling)")) -> ()  [unwired: 2 in, 2 out]
            n333 = Index Array(array=w395, index (row)=w394, index (col)=w393) -> (element=w396:T13)
            n334 = local write "_Phase"(w396) -> ()
          }
          event Value Change {
            # "(Except Configuration)"
            n335 = event-data() -> ()  [unwired: 1 in, 6 out]
            n336 = local read "State"() -> (w399:T19)
            n337 = Unbundle By Name(w399) -> ("System ADC.Battery [V]"=w408:sgl, "System ADC.DRVP [V]"=w409:sgl, "System ADC.Ext HV A [V]"=w410:sgl, "System ADC.Ext HV B [V]"=w411:sgl)
            n338 = Unbundle By Name("_DI Bank_Configuration") -> ("Power Supply Enable"=w421:bool, "Inject Enable"=w420:bool, "Boost Voltage [V]"=w401:sgl, "DI Zener Enable"=w419:bool, "DI Zener Voltage [V]"=w417:sgl, "Pump Zener Enable"=w413:bool, "Pump Zener Voltage [V]"=w414:sgl, "Boost Clamp [V]"=w406:sgl)
            n339 = local read "_Bank A?"() -> (w403:bool)
            n340 = Select(t=w410, s=w403, f=w411) -> (s? t:f=w402:sgl)
            n341 = Build Array(w401, w408, w409, w402) -> (w407:sgl[])
            n342 = property on="PSEnable" class="Bool (strict)"("Val(Sgnl)"=w421) -> ()  [unwired: 2 in, 2 out]
            n343 = property on="InjectEnable" class="Bool (strict)"("Val(Sgnl)"=w420) -> ()  [unwired: 2 in, 2 out]
            n344 = property on="BoostV" class="DigNum (strict)"("Val(Sgnl)"=w401) -> ()  [unwired: 2 in, 2 out]
            n345 = property on="ZenerEnable" class="Bool (strict)"("Val(Sgnl)"=w419) -> ()  [unwired: 2 in, 2 out]
            n346 = property on="ZenerV" class="DigNum (strict)"("Val(Sgnl)"=w417) -> ()  [unwired: 2 in, 2 out]
            n347 = property on="PumpZenerEnable" class="Bool (strict)"("Val(Sgnl)"=w413) -> ()  [unwired: 2 in, 2 out]
            n348 = property on="PumpZenerV" class="DigNum (strict)"("Val(Sgnl)"=w414) -> ()  [unwired: 2 in, 2 out]
            n349 = Array Max & Min(array=w407) -> (max value=w400:sgl)  [unwired: 3 out]
            n350 = Add(x=5.0 ("y"), y=w400) -> (x+y=w404:dbl)
            n351 = Max & Min(x=w406, y=w404) -> (max(x,y)=w398:dbl)  [unwired: 1 out]
            n352 = property on="BoostClampV" class="DigNum (strict)"("Val(Sgnl)"=w398) -> ()  [unwired: 2 in, 2 out]
            n353 = property on="Boost Clamp [V]" class="DigNum (strict)"("Value"=w398) -> ()  [unwired: 2 in, 2 out]
            n354 = property on="_Redraw Slider" class="Bool (strict)"("Val(Sgnl)"=TRUE ("Value (Signaling)")) -> ()  [unwired: 2 in, 2 out]
            n355 = property on="_Redraw Phase Plot" class="Bool (strict)"("Val(Sgnl)"=TRUE ("Value (Signaling)")) -> ()  [unwired: 2 in, 2 out]
            n356 = property on="_Redraw Pump Phase Plot" class="Bool (strict)"("Val(Sgnl)"=TRUE ("Value (Signaling)")) -> ()  [unwired: 2 in, 2 out]
          }
          event Value Change {
            n357 = event-data() -> ("NewVal"=w422:T4)  [unwired: 1 in, 5 out]
            n358 = local read "_ChannelConfigurationList"() -> (w425:i32)
            n359 = case shown="\"Piezo Unipolar 3 (Muxed)\"" w422 {
              tunnel: [4 8 7 2 3 2 4 3 2 3] -> w428
              tunnel: [TRUE ("Value (Signaling)") FALSE ("Value (Signaling)") TRUE ("Value (Signaling)") TRUE ("Value (Signaling)") TRUE ("Value (Signaling)") TRUE ("Value (Signaling)") FALSE ("Value (Signaling)") TRUE ("Value (Signaling)") TRUE ("Value (Signaling)") TRUE ("Value (Signaling)")] -> w423
              frame "Solenoid Unipolar 4" {
              }
              frame "Solenoid Unipolar 8 (Muxed)" {
              }
              frame "Solenoid Unipolar 7 (Muxed)" {
              }
              frame "Solenoid Bipolar 2" {
              }
              frame "Solenoid Bipolar 3 (Muxed)" {
              }
              frame "Piezo Unipolar 2" {
              }
              frame "Piezo Unipolar 4 (Muxed)" {
              }
              frame "Piezo Unipolar 3 (Muxed)" {
              }
              frame "Piezo Bipolar 2" {
              }
              frame "Piezo Bipolar 3 (Muxed)" {
              }
            }
            n360 = local write "_Bank Wiring Diagram"(w422) -> ()
            n361 = property on="Configuration" class="DigNum (strict)"("Val(Sgnl)"=w422) -> ()  [unwired: 2 in, 2 out]
            n362 = Decrement(x=w428) -> (x-1=w426:i32)
            n363 = property on="_Tab Control" class="TabCtl (strict)"() -> ("Pages"=w429:refnum<vi>[])  [unwired: 2 in, 2 out]
            n364 = In Range and Coerce(upper limit=w426, x=w425, lower limit=0) -> (coerced(x)=w424:i32)  [unwired: 1 out]
            n365 = for {
              tunnel: w429 -> [w460] mode=indexing
              tunnel: w423 -> [w458]
              i -> [w459]
              n366 = case shown="1, 4" w459 {
                tunnel: w460 -> [_ w462]
                tunnel: w458 -> [_ w461]
                frame 0, Default {
                }
                frame 1, 4 {
                  n367 = property class="Page"(reference=w462, "PageVis"=w461) -> ()  [unwired: 1 in, 2 out]
                }
              }
            }
            n368 = local write "_ChannelConfigurationList"(w424) -> ()
            n369 = property on="_Redraw Phase Lists" class="Bool (strict)"("Val(Sgnl)"=TRUE ("Value (Signaling)")) -> ()  [unwired: 2 in, 2 out]
            n370 = property on="_Redraw Phase Plot" class="Bool (strict)"("Val(Sgnl)"=TRUE ("Value (Signaling)")) -> ()  [unwired: 2 in, 2 out]
            n371 = property on="_Redraw Phase" class="Bool (strict)"("Val(Sgnl)"=TRUE ("Value (Signaling)")) -> ()  [unwired: 2 in, 2 out]
            n372 = property on="_Redraw Injection List" class="Bool (strict)"("Val(Sgnl)"=TRUE ("Value (Signaling)")) -> ()  [unwired: 2 in, 2 out]
            n373 = property on="_Redraw Timing Plot" class="Bool (strict)"("Val(Sgnl)"=TRUE ("Value (Signaling)")) -> ()  [unwired: 2 in, 2 out]
            n374 = property on="_Redraw Pump Phase Plot" class="Bool (strict)"("Val(Sgnl)"=TRUE ("Value (Signaling)")) -> ()  [unwired: 2 in, 2 out]
            n375 = property on="_Redraw Pump Phase List" class="Bool (strict)"("Val(Sgnl)"=TRUE ("Value (Signaling)")) -> ()  [unwired: 2 in, 2 out]
            n376 = property on="_Redraw Pump Phase" class="Bool (strict)"("Val(Sgnl)"=TRUE ("Value (Signaling)")) -> ()  [unwired: 2 in, 2 out]
          }
          event "SimInjDuration": Value Change {
            n377 = event-data() -> ()  [unwired: 1 in, 1 out]
            n378 = property on="_Redraw Phase Plot" class="Bool (strict)"("Val(Sgnl)"=TRUE ("Value (Signaling)")) -> ()  [unwired: 2 in, 2 out]
          }
          event Value Change {
            n379 = event-data() -> ()  [unwired: 1 in, 1 out]
            n380 = property on="_Redraw Phase Lists" class="Bool (strict)"("Val(Sgnl)"=TRUE ("Value (Signaling)")) -> ()  [unwired: 2 in, 2 out]
            n381 = property on="_Redraw Phase Plot" class="Bool (strict)"("Val(Sgnl)"=TRUE ("Value (Signaling)")) -> ()  [unwired: 2 in, 2 out]
            n382 = property on="_Redraw Phase" class="Bool (strict)"("Val(Sgnl)"=TRUE ("Value (Signaling)")) -> ()  [unwired: 2 in, 2 out]
            n383 = property on="_Redraw Profiles Usage Tracker" class="Bool (strict)"("Val(Sgnl)"=TRUE ("Value (Signaling)")) -> ()  [unwired: 2 in, 2 out]
            n384 = local read "PhaseArraysList"() -> (w471:i32)
            n385 = local read "Phase Array"() -> (w470:i32)
            n386 = local read "InjPhase"() -> (w472:T17)
            n387 = local read "_Phase"() -> (w469:T13)
            n388 = Replace Array Subset(array=w472, new element=w469, index (row)=w471, index (col)=w470) -> (w464:T17)
            n389 = local write "InjPhase"(w464) -> ()
          }
          event "_Remove Phase": Value Change {
            w475 = 16 ("dimension size")
            n390 = event-data() -> ()  [unwired: 1 in, 1 out]
            n391 = local write "_Remove Phase"(FALSE ("Remove Phase")) -> ()
            n392 = local read "PhaseArraysList"() -> (w485:i32)
            n393 = local read "Phase Array"() -> (w478:i32)
            n394 = local read "InjPhase"() -> (w484:T17)
            n395 = Index Array(array=w484, index (row)=w485) -> (element=w486:T13[])  [unwired: 1 in]
            n396 = property on="_Redraw Phase Lists" class="Bool (strict)"("Val(Sgnl)"=TRUE ("Value (Signaling)")) -> ()  [unwired: 2 in, 2 out]
            n397 = property on="_Redraw Phase Plot" class="Bool (strict)"("Val(Sgnl)"=TRUE ("Value (Signaling)")) -> ()  [unwired: 2 in, 2 out]
            n398 = property on="_Redraw Phase" class="Bool (strict)"("Val(Sgnl)"=TRUE ("Value (Signaling)")) -> ()  [unwired: 2 in, 2 out]
            n399 = property on="_Redraw Profiles Usage Tracker" class="Bool (strict)"("Val(Sgnl)"=TRUE ("Value (Signaling)")) -> ()  [unwired: 2 in, 2 out]
            n400 = Array Size(array=w486) -> (size(s)=w488:i32)
            n401 = Delete From Array(array=w486, index=w478) -> (array with subset deleted=w487:T13[])  [unwired: 1 in, 1 out]
            n402 = Reshape Array(w487, w488) -> (w479:T13[])
            n403 = Replace Array Subset(array=w484, new element=w479, index (row)=w485) -> (w474:T17)  [unwired: 1 in]
            n404 = Index Array(array=w479, index=w478) -> (element=w477:T13)
            n405 = Reshape Array(w474, w475, w475) -> (w473:T17)
            n406 = local write "InjPhase"(w473) -> ()
            n407 = local write "_Phase"(w477) -> ()
          }
          event "_Insert Phase": Value Change {
            w491 = 16 ("dimension size")
            n408 = event-data() -> ()  [unwired: 1 in, 1 out]
            n409 = local write "_Insert Phase"(FALSE ("Remove Phase")) -> ()
            n410 = local read "PhaseArraysList"() -> (w503:i32)
            n411 = local read "Phase Array"() -> (w494:i32)
            n412 = local read "InjPhase"() -> (w502:T17)
            n413 = Index Array(array=w502, index (row)=w503) -> (element=w496:T13[])  [unwired: 1 in]
            n414 = property on="_Redraw Phase Lists" class="Bool (strict)"("Val(Sgnl)"=TRUE ("Value (Signaling)")) -> ()  [unwired: 2 in, 2 out]
            n415 = property on="_Redraw Phase Plot" class="Bool (strict)"("Val(Sgnl)"=TRUE ("Value (Signaling)")) -> ()  [unwired: 2 in, 2 out]
            n416 = property on="_Redraw Phase" class="Bool (strict)"("Val(Sgnl)"=TRUE ("Value (Signaling)")) -> ()  [unwired: 2 in, 2 out]
            n417 = property on="_Redraw Profiles Usage Tracker" class="Bool (strict)"("Val(Sgnl)"=TRUE ("Value (Signaling)")) -> ()  [unwired: 2 in, 2 out]
            n418 = Array Size(array=w496) -> (size(s)=w504:i32)
            n419 = Index Array(array=w496, index=w494) -> (element=w495:T13)
            n420 = Insert Into Array(array=w496, index=w494, new element=w495) -> (w493:T13[])
            n421 = Reshape Array(w493, w504) -> (w497:T13[])
            n422 = Replace Array Subset(array=w502, new element=w497, index (row)=w503) -> (w490:T17)  [unwired: 1 in]
            n423 = Reshape Array(w490, w491, w491) -> (w489:T17)
            n424 = local write "InjPhase"(w489) -> ()
          }
          event "_Redraw Phase Lists": Value Change {
            n425 = event-data() -> ()  [unwired: 1 in, 1 out]
            n426 = local write "_Redraw Phase Lists"(FALSE ("Redraw Phase Lists")) -> ()
            n427 = local read "PhaseArraysList"() -> (w515:i32)
            n428 = local read "Phase Array"() -> (w510:i32)
            n429 = property on="Configuration" class="Enum (strict)"() -> ("Value"=w505:T4)  [unwired: 2 in, 2 out]
            n430 = Bundle By Name(cluster=T32 {"Configuration"=enum."Solenoid Unipolar 4", "Boost Voltage [V]"=0.0, "Zener Enable"=FALSE, "Zener Voltage [V]"=0.0} ("Configuration"), "Configuration"=w505) -> (w508:T32)
            n431 = local read "InjPhase"() -> (w506:T17)
            n432 = control-ref of="PhaseArraysList"() -> (w521:refnum<vi>)
            n433 = control-ref of="Phase Array"() -> (w520:refnum<vi>)
            n434 = In Range and Coerce(upper limit=15, x=w515, lower limit=0) -> (coerced(x)=w516:i32, In Range?=w517:bool)
            n435 = In Range and Coerce(upper limit=15, x=w510, lower limit=0) -> (coerced(x)=w509:i32, In Range?=w518:bool)
            n436 = case shown="False" w517 {
              tunnel: w516 -> [w523 _]
              frame False {
                n437 = property on="PhaseArraysList" class="LstBox (strict)"("Val(Sgnl)"=w523) -> ()  [unwired: 2 in, 2 out]
              }
              frame True {
              }
            }
            n438 = case shown="False" w518 {
              tunnel: w509 -> [w522 _]
              frame False {
                n439 = property on="Phase Array" class="LstBox (strict)"("Val(Sgnl)"=w522) -> ()  [unwired: 2 in, 2 out]
              }
              frame True {
              }
            }
            n440 = property on="InjPhase" class="Arr (strict)"("Val(Sgnl)"=w506) -> ()  [unwired: 2 in, 2 out]
            n441 = call <vilib>:"Phase Listbox.vi"(8:"Phase Arrays"=w506, "Configuration"=w508, "Phase Array"=w520, 11:"Phase Arrays"=w521) -> ()  [unwired: 7 in, 1 out]
          }
          event "_Redraw Phase Plot": Value Change {
            n442 = event-data() -> ()  [unwired: 1 in, 1 out]
            n443 = local read "_DI Bank_Configuration"() -> (w554:T3)
            n444 = local read "InjCapacitance"() -> (w524:sgl)
            n445 = local read "InjInductance"() -> (w525:sgl)
            n446 = local read "InjResistance"() -> (w526:sgl)
            n447 = Bundle By Name(cluster=T33 {"Resistance [Ohm]"=1.0, "Inductance [Henery]"=0.001, "Capacitance [Farad]"=5e-06} ("Injector Configuration"), "Resistance [Ohm]"=w526, "Inductance [Henery]"=w525, "Capacitance [Farad]"=w524) -> (w528:T33)
            n448 = local read "SimBatt"() -> (w527:sgl)
            n449 = Unbundle By Name(w554) -> ("Configuration"=w553:T4, "Boost Voltage [V]"=w552:sgl, "DI Zener Enable"=w551:bool, "DI Zener Voltage [V]"=w550:sgl)
            n450 = local read "_Ref Inj Profiles"() -> (w541:cluster{"Array":dbl[], "Array":dbl[]}[])
            n451 = local read "PhaseArraysList"() -> (w560:i32)
            n452 = local read "InjPhase"() -> (w561:T17)
            n453 = Bundle By Name(cluster=T34 {"Battery [V]"=13.7, "Engine Speed [RPM]"=0.0, "Rotations"=0, "Injector Configuration"={"Resistance [Ohm]"=1.0, "Inductance [Henery]"=0.001, "Capacitance [Farad]"=5e-06}, "Description"=""} ("System"), "Battery [V]"=w527, "Injector Configuration"=w528) -> (w557:T34)
            n454 = local read "Profiles"() -> (w530:sgl[][])
            n455 = Bundle By Name(cluster=T32 {"Configuration"=enum."Solenoid Unipolar 4", "Boost Voltage [V]"=0.0, "Zener Enable"=FALSE, "Zener Voltage [V]"=0.0} ("Configuration"), "Configuration"=w553, "Boost Voltage [V]"=w552, "Zener Enable"=w551, "Zener Voltage [V]"=w550) -> (w555:T32)
            n456 = Index Array(array=w541) -> (element #1=w540:cluster{"Array":dbl[], "Array":dbl[]}, element #2=w539:cluster{"Array":dbl[], "Array":dbl[]})  [unwired: 2 in]
            n457 = Unbundle(w540) -> ("Array"=w549:dbl[], "Array"=w548:dbl[])
            n458 = Unbundle(w539) -> ("Array"=w538:dbl[], "Array"=w532:dbl[])
            n459 = Index Array(array=w561, index (row)=w560) -> (element=w562:T13[])  [unwired: 1 in]
            n460 = local write "_Redraw Phase Plot"(FALSE ("Redraw Phase Plot")) -> ()
            n461 = call <vilib>:"Phase Plot.vi"("Phase Arrays"=w562, "Profiles - Pulse Width [s]"=w530, "System"=w557, "Configuration"=w555, "Duration (1m) [s]"="SimInjDuration") -> ("Plot"=w543:cluster{"Array":sgl[], "Array":sgl[]}[])  [unwired: 13 in, 1 out]
            n462 = for {
              tunnel: w549 -> [w568] mode=indexing
              tunnel: [w568] -> w547 mode=indexing if=w566
              tunnel: [w567] -> w546 mode=indexing if=w566
              tunnel: w548 -> [w567] mode=indexing
              n463 = Greater Or Equal To 0?(x=w568) -> (x >= 0?=w566:bool)
            }
            n464 = for {
              tunnel: w538 -> [w565] mode=indexing
              tunnel: [w565] -> w537 mode=indexing if=w563
              tunnel: [w564] -> w536 mode=indexing if=w563
              tunnel: w532 -> [w564] mode=indexing
              n465 = Greater Or Equal To 0?(x=w565) -> (x >= 0?=w563:bool)
            }
            n466 = Empty Array?(array=w548) -> (empty?=w535:bool)
            n467 = Empty Array?(array=w532) -> (empty?=w534:bool)
            n468 = Compound Arithmetic op=OR(invert w535, invert w534) -> (w533:bool)
            n469 = Bundle(w547, w546) -> (w545:cluster{dbl[], dbl[]})  [unwired: 1 in]
            n470 = Bundle(w537, w536) -> (w531:cluster{dbl[], dbl[]})  [unwired: 1 in]
            n471 = case shown="True" w533 {
              tunnel: w543 -> [w570 w581]
              tunnel: [w570 w580] -> w542
              tunnel: w545 -> [_ w579]
              tunnel: w531 -> [_ w578]
              frame False {
                n472 = property on="_Phase Plot" class="XYGraph (strict)"("LegNumRows"=u32 10 ("Legend:Number of Rows")) -> ()  [unwired: 2 in, 2 out]
              }
              frame True {
                n473 = Build Array (concatenate)(w581, w579, w578) -> (w580:cluster{"Array":dbl[], "Array":dbl[]}[])
                n474 = property on="_Phase Plot" class="XYGraph (strict)"("Active Plot"=u32 10, "Plot.Plot Name"="Ref I [A]", "Plot.YScaleIdx"=u32 1 ("Plot.Y Scale Index"), "Active Plot"=u32 11, "Plot.Plot Name"="Ref V [V]", "Plot.YScaleIdx"=u32 0 ("Plot.Y Scale Index"), "LegNumRows"=u32 12 ("Legend:Number of Rows")) -> ()  [unwired: 2 in, 2 out]
              }
            }
            "_SimuXY" <- w542
          }
          event "_Redraw Phase": Value Change {
            n475 = event-data() -> ()  [unwired: 1 in, 1 out]
            n476 = local write "_Redraw Phase"(FALSE ("Redraw Phase")) -> ()
            n477 = property on="Configuration" class="Enum (strict)"() -> ("Value"=w582:T4)  [unwired: 2 in, 2 out]
            n478 = Bundle By Name(cluster=T32 {"Configuration"=enum."Solenoid Unipolar 4", "Boost Voltage [V]"=0.0, "Zener Enable"=FALSE, "Zener Voltage [V]"=0.0} ("Configuration"), "Configuration"=w582) -> (w585:T32)
            n479 = control-ref of="_Phase"() -> (w583:refnum<vi>)
            n480 = call <vilib>:"Disable Phase Array.vi"("Configuration"=w585, "Phase Ref"=w583) -> ()  [unwired: 10 in]
          }
          event "ProfilesAdapt": Value Change {
            n481 = event-data() -> ("NewVal"=w589:bool)  [unwired: 1 in]
            n482 = Select(t=T30."Disabled and Grayed Out" ("Disabled"), s=w589, f=T30."Enabled" ("Disabled")) -> (s? t:f=w587:T30)
            n483 = property on="Profiles" class="Arr (strict)"("Array Element.DisabledEnum"=w587) -> ()  [unwired: 2 in, 2 out]
          }
          event "_Redraw Profiles Usage Tracker": Value Change {
            n484 = event-data() -> ()  [unwired: 1 in, 6 out]
            n485 = local write "_Redraw Profiles Usage Tracker"(FALSE ("_Redraw Profiles Usage Tracker")) -> ()
            n486 = local read "InjPhase"() -> (w591:T17)
            n487 = control-ref of="_Profiles usage tracker"() -> (w593:refnum<vi>)
            n488 = call "Format Phase Profiles Tracker.vi"("InjPhase"=w591, "Listbox Ref"=w593) -> ()  [unwired: 10 in]
          }
          event "_Ref Inj FilePath": Value Change {
            n489 = event-data() -> ()  [unwired: 1 in, 6 out]
            n490 = Read from Text File(file (use dialog)="_Ref Inj FilePath") -> (text=w615:string)  [unwired: 3 in, 3 out]
            n491 = Spreadsheet String To Array(delimiter (Tab)=",", format string="%s", spreadsheet string=w615) -> (array=w618:dbl[][])  [unwired: 1 in]
            n492 = Transpose 2D Array(2D array=w618) -> (transposed array=w612:dbl[][])
            n493 = Index Array(array=w612) -> (element #1=w605:dbl[], element #2=w601:dbl[], element #3=w598:dbl[])  [unwired: 6 in]
            n494 = property on="_Redraw Phase Plot" class="Bool (strict)"("Val(Sgnl)"=TRUE ("Value (Signaling)")) -> ()  [unwired: 2 in, 2 out]
            n495 = Compound Arithmetic op=MULTIPLY("RefInjTimeAxisMultiplier", w605) -> (w608:dbl[])
            n496 = Compound Arithmetic op=MULTIPLY("RefInjCurrentMultiplier", w601) -> (w607:dbl[])
            n497 = Compound Arithmetic op=MULTIPLY("RefInjVoltageMultiplier", w598) -> (w606:dbl[])
            n498 = Compound Arithmetic op=ADD("RefInjTimeAxisOffset", w608) -> (w596:dbl[])
            n499 = Compound Arithmetic op=ADD(w607, "RefInjCurrentOffset") -> (w595:dbl[])
            n500 = Compound Arithmetic op=ADD(w606, "RefInjVoltageOffset") -> (w594:dbl[])
            n501 = Bundle(w596, w595) -> (w611:cluster{dbl[], dbl[]})  [unwired: 1 in]
            n502 = Bundle(w596, w594) -> (w609:cluster{dbl[], dbl[]})  [unwired: 1 in]
            n503 = Build Array(w611, w609) -> (→"_Ref Inj Profiles":cluster{dbl[], dbl[]}[])
          }
          event "_Save Profile": Value Change {
            n504 = event-data() -> ()  [unwired: 1 in, 1 out]
            n505 = local read "PhaseArraysList"() -> (w621:i32)
            n506 = local read "InjPhase"() -> (w620:T17)
            n507 = Index Array(array=w620, index (row)=w621) -> (element=w619:T13[])  [unwired: 1 in]
            n508 = call <vilib>:"Save Phase Array.vi"("Phase Array"=w619) -> ()  [unwired: 11 in]
          }
          event "_Apply Profile": Value Change {
            n509 = event-data() -> ()  [unwired: 1 in, 6 out]
            n510 = local read "PhaseArraysList"() -> (w624:i32)
            n511 = local read "InjPhase"() -> (w625:T17)
            n512 = call <vilib>:"Load Phase Array.vi"() -> ("error out"=w622:errorcluster, "Phase Array"=w623:T13[])  [unwired: 10 in]
            n513 = case shown="No Error" w622 {
              selector: w622 -> [_ w634]
              tunnel: w623 -> [w633 _]
              tunnel: w625 -> [w632 _]
              tunnel: w624 -> [w631 _]
              frame No Error {
                n514 = Replace Array Subset(array=w632, new element=w633, index (row)=w631) -> (w626:T17)  [unwired: 1 in]
                n515 = property on="_Redraw Phase Lists" class="Bool (strict)"("Val(Sgnl)"=TRUE ("Value (Signaling)")) -> ()  [unwired: 2 in, 2 out]
                n516 = property on="_Redraw Phase Plot" class="Bool (strict)"("Val(Sgnl)"=TRUE ("Value (Signaling)")) -> ()  [unwired: 2 in, 2 out]
                n517 = property on="_Redraw Phase" class="Bool (strict)"("Val(Sgnl)"=TRUE ("Value (Signaling)")) -> ()  [unwired: 2 in, 2 out]
                n518 = property on="_Redraw Profiles Usage Tracker" class="Bool (strict)"("Val(Sgnl)"=TRUE ("Value (Signaling)")) -> ()  [unwired: 2 in, 2 out]
                n519 = local write "InjPhase"(w626) -> ()
              }
              frame Error {
                n520 = call <vilib>:"Simple Error Handler.vi"("error in (no error)"=w634) -> ()  [unwired: 4 in, 5 out]
              }
            }
          }
          event "_ChannelConfigurationList": Value Change {
            n521 = event-data() -> ()  [unwired: 1 in, 1 out]
            n522 = local read "InjCmd"() -> (w645:T6)
            n523 = local read "InjAdaptMode"() -> (w642:u32)
            n524 = Number To Boolean Array(number=w642) -> (Boolean array=w641:bool[])
            n525 = Index Array(array=w645, index="_ChannelConfigurationList") -> (element=w644:T7)
            n526 = Index Array(array=w641, index="_ChannelConfigurationList") -> (element=w637:bool)
            n527 = property on="_Redraw Timing Plot" class="Bool (strict)"("Val(Sgnl)"=TRUE ("Value (Signaling)")) -> ()  [unwired: 2 in, 2 out]
            n528 = property on="_Redraw DI Command" class="Bool (strict)"("Val(Sgnl)"=TRUE ("Value (Signaling)")) -> ()  [unwired: 2 in, 2 out]
            n529 = local write "_InjCmd Element"(w644) -> ()
            n530 = Select(t=T30."Disabled and Grayed Out" ("Disabled"), s=w637, f=T30."Enabled" ("Disabled")) -> (s? t:f=w638:T30)
            n531 = local write "_InjAdaptMode"(w637) -> ()
            n532 = property on="_InjCmd Element" class="Clust (strict)"("DisabledEnum"=w638) -> ()  [unwired: 2 in, 2 out]
          }
          event Value Change {
            n533 = event-data() -> ()  [unwired: 1 in, 1 out]
            n534 = property on="_Redraw Injection List" class="Bool (strict)"("Val(Sgnl)"=TRUE ("Value (Signaling)")) -> ()  [unwired: 2 in, 2 out]
            n535 = property on="_Redraw Timing Plot" class="Bool (strict)"("Val(Sgnl)"=TRUE ("Value (Signaling)")) -> ()  [unwired: 2 in, 2 out]
            n536 = property on="_Redraw DI Command" class="Bool (strict)"("Val(Sgnl)"=TRUE ("Value (Signaling)")) -> ()  [unwired: 2 in, 2 out]
            n537 = local read "_ChannelConfigurationList"() -> (w652:i32)
            n538 = local read "InjCmd"() -> (w653:T6)
            n539 = call "Resize DI Command Array.vi"("Command in"="_InjCmd Element") -> ("Command out"=w647:T7)
            n540 = Replace Array Subset(array=w653, new element=w647, index=w652) -> (w646:T6)
            n541 = local write "InjCmd"(w646) -> ()
          }
          event "_InjAdaptMode": Value Change {
            n542 = event-data() -> ("NewVal"=w655:bool)  [unwired: 1 in]
            n543 = local read "_ChannelConfigurationList"() -> (w660:i32)
            n544 = local read "InjAdaptMode"() -> (w661:u32)
            n545 = Number To Boolean Array(number=w661) -> (Boolean array=w662:bool[])
            n546 = Replace Array Subset(array=w662, new element=w655, index=w660) -> (w663:bool[])
            n547 = case shown="False" w655 {
              frame False {
                n548 = property on="_Redraw DI Command" class="Bool (strict)"("Val(Sgnl)"=TRUE ("Value (Signaling)")) -> ()  [unwired: 2 in, 2 out]
              }
              frame True {
              }
            }
            n549 = property on="_Redraw Injection List" class="Bool (strict)"("Val(Sgnl)"=TRUE ("Value (Signaling)")) -> ()  [unwired: 2 in, 2 out]
            n550 = Boolean Array To Number(Boolean array=w663) -> (number=w659:u32)
            n551 = property on="InjAdaptMode" class="DigNum (strict)"("Val(Sgnl)"=w659) -> ()  [unwired: 2 in, 2 out]
            n552 = Select(t=T30."Disabled and Grayed Out" ("Disabled"), s=w655, f=T30."Enabled" ("Disabled")) -> (s? t:f=w656:T30)
            n553 = property on="_InjCmd Element" class="Clust (strict)"("DisabledEnum"=w656) -> ()  [unwired: 2 in, 2 out]
          }
          event "_DI_CopyToAllChannelConf": Value Change {
            # "Copy selected cmd channel to active cmd channels; coerce all non-active channels to OFF command state"
            n554 = event-data() -> ()  [unwired: 1 in, 1 out]
            n555 = local read "_DI Bank_Configuration"() -> (w672:T3)
            n556 = local write "_DI_CopyToAllChannelConf"(FALSE ("_Copy To All")) -> ()
            n557 = property on="_Redraw Injection List" class="Bool (strict)"("Val(Sgnl)"=TRUE ("Value (Signaling)")) -> ()  [unwired: 2 in, 2 out]
            n558 = Unbundle By Name(w672) -> ("Configuration"=w673:T4)
            n559 = local read "_ChannelConfigurationList"() -> (w667:i32)
            n560 = case shown="\"Piezo Unipolar 2\"" w673 {
              tunnel: [bool[] [TRUE, TRUE, TRUE, TRUE, FALSE, FALSE, FALSE, FALSE] bool[] [TRUE, TRUE, TRUE, TRUE, TRUE, TRUE, TRUE, FALSE] bool[] [TRUE, TRUE, TRUE, TRUE, TRUE, TRUE, TRUE, TRUE] bool[] [FALSE, TRUE, FALSE, TRUE, FALSE, FALSE, FALSE, FALSE] bool[] [FALSE, TRUE, TRUE, TRUE, FALSE, FALSE, FALSE, FALSE] bool[] [FALSE, TRUE, FALSE, TRUE, FALSE, FALSE, FALSE, FALSE] bool[] [FALSE, TRUE, TRUE, TRUE, FALSE, FALSE, FALSE, FALSE] bool[] [TRUE, TRUE, TRUE, TRUE, FALSE, FALSE, FALSE, FALSE] bool[] [FALSE, TRUE, FALSE, TRUE, FALSE, FALSE, FALSE, FALSE] bool[] [FALSE, TRUE, TRUE, TRUE, FALSE, FALSE, FALSE, FALSE]] -> w669
              frame "Solenoid Unipolar 4", Default {
              }
              frame "Solenoid Unipolar 7 (Muxed)" {
              }
              frame "Solenoid Unipolar 8 (Muxed)" {
              }
              frame "Solenoid Bipolar 2" {
              }
              frame "Solenoid Bipolar 3 (Muxed)" {
              }
              frame "Piezo Unipolar 2" {
              }
              frame "Piezo Unipolar 3 (Muxed)" {
              }
              frame "Piezo Unipolar 4 (Muxed)" {
              }
              frame "Piezo Bipolar 2" {
              }
              frame "Piezo Bipolar 3 (Muxed)" {
              }
            }
            n561 = local read "InjCmd"() -> (w668:T6)
            n562 = Index Array(array=w668, index=w667) -> (element=w670:T7)
            n563 = for {
              N: 8 -> [_]
              shift-right: [w675] -> w665
              shift-left: w668 -> [w679]
              tunnel: w670 -> [w677]
              tunnel: w669 -> [w676] mode=indexing
              i -> [w678]
              n564 = in-place {
                in-place-border: w677 -> [w682]
                in-place-border: w676 -> [w683]
                n565 = in-place-array #2(w679, w678) -> (w680:T7)
                n566 = case shown="False" w683 {
                  tunnel: w682 -> [_ w685]
                  tunnel: [w684 w685] -> w681
                  tunnel: w680 -> [w684 _]
                  frame False {
                  }
                  frame True {
                  }
                }
                n567 = in-place-array #2(w681) -> (w675:T6)  [unwired: 1 out]
              }
            }
            n568 = local write "InjCmd"(w665) -> ()
          }
          event "_Plot Selector (T=TMP, F=EPT)": Value Change {
            n569 = event-data() -> ()  [unwired: 1 in, 6 out]
            n570 = property on="_Redraw Timing Plot" class="Bool (strict)"("Val(Sgnl)"=TRUE ("Value (Signaling)")) -> ()  [unwired: 2 in, 2 out]
          }
          event "_Redraw Timing Plot": Value Change {
            n571 = event-data() -> ()  [unwired: 1 in, 6 out]
            n572 = local write "_Redraw Timing Plot"(FALSE ("_Redraw Timing Plot")) -> ()
            n573 = local read "SimRotations"() -> (w701:u8)
            n574 = local read "SimSpeed"() -> (w702:sgl)
            n575 = local read "_ChannelConfigurationList"() -> (w712:i32)
            n576 = local read "SimBatt"() -> (w703:sgl)
            n577 = local read "InjCmd"() -> (w713:T6)
            n578 = Bundle By Name(cluster=T34 {"Battery [V]"=13.7, "Engine Speed [RPM]"=1000.0, "Rotations"=2, "Injector Configuration"={"Resistance [Ohm]"=1.0, "Inductance [Henery]"=0.001, "Capacitance [Farad]"=5e-06}, "Description"=""} ("System Configuration"), "Battery [V]"=w703, "Engine Speed [RPM]"=w702, "Rotations"=w701) -> (w697:T34)
            n579 = Index Array(array=w713, index=w712) -> (element=w698:T7)
            n580 = Select(t="Time after Trigger [sec]" ("X Scale.Name Label.Text 2"), s="_Plot Selector (T=TMP, F=EPT)", f="Timing [DBTDC]" ("X Scale.Name Label.Text 2")) -> (s? t:f=w708:string)
            n581 = Select(t="Trigger" ("Plot.Plot Name 2"), s="_Plot Selector (T=TMP, F=EPT)", f="Window" ("Plot.Plot Name 2")) -> (s? t:f=w711:string)
            n582 = case shown="False" "_Plot Selector (T=TMP, F=EPT)" {
              tunnel: [w716 w719] -> w699
              tunnel: w698 -> [w717 w718]
              tunnel: w697 -> [w715 _]
              frame False {
                n583 = call "Injection Command Plot - EPT.vi"("System"=w715, "Injection Command"=w717) -> ("Plot"=w716:cluster{"Array":sgl[], "Array":sgl[]}[])  [unwired: 9 in]
              }
              frame True {
                n584 = call "Injection Command Plot - TMP.vi"("Injection Command"=w718) -> ("Plot"=w719:cluster{"Array":sgl[], "Array":sgl[]}[])  [unwired: 10 in]
              }
            }
            "_Timing Plot" <- w699
            n585 = property on="_Timing Plot" class="XYGraph (strict)"("XScale.NameLbl.Text"=w708, "Active Plot"=u32 0, "Plot.Plot Name"=w711) -> ()  [unwired: 2 in, 2 out]
          }
          event "_Redraw DI Command": Value Change {
            n586 = event-data() -> ()  [unwired: 1 in, 6 out]
            n587 = local write "_Redraw DI Command"(FALSE ("_Redraw DI Command")) -> ()
            n588 = control-ref of="_InjCmd Element"() -> (w720:refnum<vi>)
            n589 = call "Disable DI Command.vi"("Phase Ref"=w720) -> ()  [unwired: 11 in]
          }
          event "_Redraw Injection List": Value Change {
            n590 = event-data() -> ()  [unwired: 1 in, 1 out]
            n591 = local read "_DI Bank_Configuration"() -> (w727:T3)
            n592 = local read "InjCmd"() -> (w724:T6)
            n593 = local read "InjAdaptMode"() -> (w725:u32)
            n594 = local read "_Bank A?"() -> (w722:bool)
            n595 = control-ref of="_ChannelConfigurationList"() -> (w726:refnum<vi>)
            n596 = local write "_Redraw Injection List"(FALSE ("_Redraw Injection List")) -> ()
            n597 = call "Injection Configuration Listbox Setup.vi"("Bank A? (T)"=w722, "Inj Adapt Mode"=w725, "Command Cluster Array"=w724, "DI Bank Configuration"=w727, "Injection Configurations"=w726) -> ("Command Cluster Array"=w723:T7[])  [unwired: 6 in]
            n598 = property on="InjCmd" class="Arr (strict)"("Val(Sgnl)"=w723) -> ()  [unwired: 2 in, 2 out]
          }
          event "_DI-A Fault Clear": Value Change {
            n599 = event-data() -> ("NewVal"=w729:T27)  [unwired: 1 in]
            n600 = Cluster To Array(cluster=w729) -> (array=w731:bool[])
            n601 = Boolean Array To Number(Boolean array=w731) -> (number=w730:u8)
            n602 = property on="FaultClear" class="DigNum (strict)"("Val(Sgnl)"=w730) -> ()  [unwired: 2 in, 2 out]
          }
          event "PumpPhase Array": Value Change {
            n603 = event-data() -> ()  [unwired: 1 in, 6 out]
            n604 = local read "PumpPhase Array"() -> (w734:i32)
            n605 = local read "PumpPhase"() -> (w733:T12)
            n606 = property on="_Redraw Pump Phase" class="Bool (strict)"("Val(Sgnl)"=TRUE ("Value (Signaling)")) -> ()  [unwired: 2 in, 2 out]
            n607 = Index Array(array=w733, index=w734) -> (element=w735:T13)
            n608 = local write "_Pump Phase"(w735) -> ()
          }
          event "_Insert Pump Phase": Value Change {
            n609 = event-data() -> ()  [unwired: 1 in, 6 out]
            n610 = local read "PumpPhase Array"() -> (w742:i32)
            n611 = local read "PumpPhase"() -> (w743:T12)
            n612 = local write "_Insert Pump Phase"(FALSE ("_Insert Pump Phase 2")) -> ()
            n613 = Index Array(array=w743, index=w742) -> (element=w741:T13)
            n614 = property on="_Redraw Pump Phase" class="Bool (strict)"("Val(Sgnl)"=TRUE ("Value (Signaling)")) -> ()  [unwired: 2 in, 2 out]
            n615 = property on="_Redraw Pump Phase Plot" class="Bool (strict)"("Val(Sgnl)"=TRUE ("Value (Signaling)")) -> ()  [unwired: 2 in, 2 out]
            n616 = property on="_Redraw Pump Phase List" class="Bool (strict)"("Val(Sgnl)"=TRUE ("Value (Signaling)")) -> ()  [unwired: 2 in, 2 out]
            n617 = Insert Into Array(array=w743, index=w742, new element=w741) -> (w737:T12)
            n618 = Reshape Array(w737, 16 ("dimension size")) -> (w736:T12)
            n619 = local write "PumpPhase"(w736) -> ()
          }
          event "_Remove Pump Phase": Value Change {
            n620 = event-data() -> ()  [unwired: 1 in, 6 out]
            n621 = local read "PumpPhase Array"() -> (w752:i32)
            n622 = local read "PumpPhase"() -> (w750:T12)
            n623 = local write "_Remove Pump Phase"(FALSE ("_Remove Pump Phase")) -> ()
            n624 = property on="_Redraw Pump Phase" class="Bool (strict)"("Val(Sgnl)"=TRUE ("Value (Signaling)")) -> ()  [unwired: 2 in, 2 out]
            n625 = property on="_Redraw Pump Phase Plot" class="Bool (strict)"("Val(Sgnl)"=TRUE ("Value (Signaling)")) -> ()  [unwired: 2 in, 2 out]
            n626 = property on="_Redraw Pump Phase List" class="Bool (strict)"("Val(Sgnl)"=TRUE ("Value (Signaling)")) -> ()  [unwired: 2 in, 2 out]
            n627 = Delete From Array(array=w750, index=w752) -> (array with subset deleted=w751:T12)  [unwired: 1 in, 1 out]
            n628 = Index Array(array=w751, index=w752) -> (element=w753:T13)
            n629 = Reshape Array(w751, 16 ("dimension size")) -> (w747:T12)
            n630 = local write "PumpPhase"(w747) -> ()
            n631 = local write "_Pump Phase"(w753) -> ()
          }
          event Value Change {
            n632 = event-data() -> ()  [unwired: 1 in, 6 out]
            n633 = local read "PumpPhase Array"() -> (w761:i32)
            n634 = local read "PumpPhase"() -> (w760:T12)
            n635 = Replace Array Subset(array=w760, new element="_Pump Phase", index=w761) -> (w756:T12)
            n636 = property on="_Redraw Pump Phase List" class="Bool (strict)"("Val(Sgnl)"=TRUE ("Value (Signaling)")) -> ()  [unwired: 2 in, 2 out]
            n637 = property on="_Redraw Pump Phase" class="Bool (strict)"("Val(Sgnl)"=TRUE ("Value (Signaling)")) -> ()  [unwired: 2 in, 2 out]
            n638 = property on="_Redraw Pump Phase Plot" class="Bool (strict)"("Val(Sgnl)"=TRUE ("Value (Signaling)")) -> ()  [unwired: 2 in, 2 out]
            n639 = local write "PumpPhase"(w756) -> ()
          }
          event "SimPumpDuration": Value Change {
            n640 = event-data() -> ()  [unwired: 1 in, 6 out]
            n641 = property on="_Redraw Pump Phase Plot" class="Bool (strict)"("Val(Sgnl)"=TRUE ("Value (Signaling)")) -> ()  [unwired: 2 in, 2 out]
          }
          event "_Redraw Pump Phase Plot": Value Change {
            n642 = event-data() -> ()  [unwired: 1 in, 6 out]
            n643 = local read "_DI Bank_Configuration"() -> (w796:T3)
            n644 = local read "PumpCapacitance"() -> (w771:sgl)
            n645 = local read "PumpInductance"() -> (w772:sgl)
            n646 = local read "PumpResistance"() -> (w773:sgl)
            n647 = Bundle By Name(cluster=T33 {"Resistance [Ohm]"=1.0, "Inductance [Henery]"=0.001, "Capacitance [Farad]"=5e-06} ("Injector Configuration"), "Resistance [Ohm]"=w773, "Inductance [Henery]"=w772, "Capacitance [Farad]"=w771) -> (w769:T33)
            n648 = Unbundle By Name(w796) -> ("Boost Voltage [V]"=w795:sgl, "Pump Zener Enable"=w764:bool, "Pump Zener Voltage [V]"=w765:sgl)
            n649 = local read "SimBatt"() -> (w770:sgl)
            n650 = local read "_Ref Pump Profiles"() -> (w787:cluster{"Array":dbl[], "Array":dbl[]}[])
            n651 = Bundle By Name(cluster=T34 {"Battery [V]"=13.7, "Engine Speed [RPM]"=0.0, "Rotations"=0, "Injector Configuration"={"Resistance [Ohm]"=1.0, "Inductance [Henery]"=0.001, "Capacitance [Farad]"=5e-06}, "Description"=""} ("System"), "Battery [V]"=w770, "Injector Configuration"=w769) -> (w794:T34)
            n652 = Bundle By Name(cluster=T32 {"Configuration"=enum."Solenoid Unipolar 4", "Boost Voltage [V]"=0.0, "Zener Enable"=FALSE, "Zener Voltage [V]"=0.0} ("Configuration"), "Configuration"=DI_-_Bank_Configuration."Solenoid Unipolar 4", "Boost Voltage [V]"=w795, "Zener Enable"=w764, "Zener Voltage [V]"=w765) -> (w793:T32)
            n653 = local read "PumpPhase"() -> (w792:T12)
            n654 = Index Array(array=w787) -> (element #1=w786:cluster{"Array":dbl[], "Array":dbl[]}, element #2=w784:cluster{"Array":dbl[], "Array":dbl[]})  [unwired: 2 in]
            n655 = Unbundle(w786) -> ("Array"=w783:dbl[], "Array"=w785:dbl[])
            n656 = Unbundle(w784) -> ("Array"=w782:dbl[], "Array"=w776:dbl[])
            n657 = call <vilib>:"Phase Plot.vi"("Phase Arrays"=w792, "System"=w794, "Configuration"=w793, "Duration (1m) [s]"="SimPumpDuration") -> ("Plot"=w789:cluster{"Array":sgl[], "Array":sgl[]}[])  [unwired: 14 in, 1 out]
            n658 = for {
              tunnel: w783 -> [w803] mode=indexing
              tunnel: [w803] -> w791 mode=indexing if=w804
              tunnel: [w805] -> w790 mode=indexing if=w804
              tunnel: w785 -> [w805] mode=indexing
              n659 = Greater Or Equal To 0?(x=w803) -> (x >= 0?=w804:bool)
            }
            n660 = for {
              tunnel: w782 -> [w800] mode=indexing
              tunnel: [w800] -> w781 mode=indexing if=w801
              tunnel: [w802] -> w780 mode=indexing if=w801
              tunnel: w776 -> [w802] mode=indexing
              n661 = Greater Or Equal To 0?(x=w800) -> (x >= 0?=w801:bool)
            }
            n662 = Empty Array?(array=w785) -> (empty?=w777:bool)
            n663 = Empty Array?(array=w776) -> (empty?=w775:bool)
            n664 = local write "_Redraw Pump Phase Plot"(FALSE ("_Redraw Pump Phase Plot")) -> ()
            n665 = Compound Arithmetic op=OR(invert w777, invert w775) -> (w778:bool)
            n666 = Bundle(w791, w790) -> (w788:cluster{dbl[], dbl[]})  [unwired: 1 in]
            n667 = Bundle(w781, w780) -> (w779:cluster{dbl[], dbl[]})  [unwired: 1 in]
            n668 = case shown="True" w778 {
              tunnel: w789 -> [w807 w814]
              tunnel: [w807 w813] -> w768
              tunnel: w788 -> [_ w809]
              tunnel: w779 -> [_ w808]
              frame False {
                n669 = property on="_Pump Phase Plot" class="XYGraph (strict)"("LegNumRows"=u32 6 ("Legend:Number of Rows")) -> ()  [unwired: 2 in, 2 out]
              }
              frame True {
                n670 = Build Array (concatenate)(w814, w809, w808) -> (w813:cluster{"Array":dbl[], "Array":dbl[]}[])
                n671 = property on="_Pump Phase Plot" class="XYGraph (strict)"("Active Plot"=u32 6, "Plot.Plot Name"="Ref [A]", "LegNumRows"=u32 7 ("Legend:Number of Rows")) -> ()  [unwired: 2 in, 2 out]
              }
            }
            "_Pump Phase Plot" <- w768
          }
          event "_Redraw Pump Phase List": Value Change {
            n672 = event-data() -> ()  [unwired: 1 in, 6 out]
            n673 = local read "PumpPhase"() -> (w815:T12)
            n674 = local read "PumpPhase Array"() -> (w819:i32)
            n675 = control-ref of="PumpPhase Array"() -> (w822:refnum<vi>)
            n676 = Build Array(w815) -> (w821:T13[][])
            n677 = property on="PumpPhase" class="Arr (strict)"("Val(Sgnl)"=w815) -> ()  [unwired: 2 in, 2 out]
            n678 = call <vilib>:"Phase Listbox.vi"("Phase Arrays"=w821, "Phase Array"=w822) -> ()  [unwired: 9 in, 1 out]
            n679 = In Range and Coerce(upper limit=15, x=w819, lower limit=0) -> (coerced(x)=w820:i32, In Range?=w816:bool)
            n680 = case shown="False" w816 {
              tunnel: w820 -> [w824 _]
              frame False {
                n681 = property on="PumpPhase Array" class="LstBox (strict)"("Val(Sgnl)"=w824) -> ()  [unwired: 2 in, 2 out]
              }
              frame True {
              }
            }
            n682 = local write "_Redraw Pump Phase List"(FALSE ("_Redraw Pump Phase List")) -> ()
          }
          event "_Redraw Pump Phase": Value Change {
            n683 = event-data() -> ()  [unwired: 1 in, 1 out]
            n684 = local read "_DI Bank_Configuration"() -> (w833:T3)
            n685 = local write "_Redraw Pump Phase"(FALSE ("Redraw Phase")) -> ()
            n686 = Unbundle By Name(w833) -> ("Configuration"=w832:T4, "Boost Voltage [V]"=w831:sgl, "DI Zener Enable"=w830:bool, "DI Zener Voltage [V]"=w829:sgl)
            n687 = Bundle By Name(cluster=T32 {"Configuration"=enum."Solenoid Unipolar 4", "Boost Voltage [V]"=0.0, "Zener Enable"=FALSE, "Zener Voltage [V]"=0.0} ("Configuration"), "Configuration"=w832, "Boost Voltage [V]"=w831, "Zener Enable"=w830, "Zener Voltage [V]"=w829) -> (w827:T32)
            n688 = control-ref of="_Pump Phase"() -> (w826:refnum<vi>)
            n689 = call <vilib>:"Disable Phase Array.vi"("Pump (F)"=TRUE, "Configuration"=w827, "Phase Ref"=w826) -> ()  [unwired: 9 in]
          }
          event "_Ref Pump Current Profile FilePath": Value Change {
            n690 = event-data() -> ()  [unwired: 1 in, 6 out]
            n691 = Read from Text File(file (use dialog)="_Ref Pump Current Profile FilePath") -> (text=w855:string)  [unwired: 3 in, 3 out]
            n692 = Spreadsheet String To Array(delimiter (Tab)=",", format string="%g", spreadsheet string=w855) -> (array=w858:dbl[][])  [unwired: 1 in]
            n693 = Transpose 2D Array(2D array=w858) -> (transposed array=w854:dbl[][])
            n694 = Index Array(array=w854) -> (element #1=w849:dbl[], element #2=w851:dbl[], element #3=w842:dbl[])  [unwired: 6 in]
            n695 = Compound Arithmetic op=MULTIPLY("RefPumpTimeAxisMultiplier", w849) -> (w850:dbl[])
            n696 = Compound Arithmetic op=MULTIPLY("RefPumpCurrentMultiplier", w851) -> (w844:dbl[])
            n697 = Compound Arithmetic op=MULTIPLY("RefPumpVoltageMultiplier", w842) -> (w843:dbl[])
            n698 = Compound Arithmetic op=ADD(w850, "RefPumpTimeAxisOffset") -> (w838:dbl[])
            n699 = Compound Arithmetic op=ADD(w844, "RefPumpCurrentOffset") -> (w852:dbl[])
            n700 = Compound Arithmetic op=ADD(w843, "RefPumpVoltageOffset") -> (w839:dbl[])
            n701 = property on="_Redraw Pump Phase Plot" class="Bool (strict)"("Val(Sgnl)"=TRUE ("Value (Signaling)")) -> ()  [unwired: 2 in, 2 out]
            n702 = Bundle(w838, w852) -> (w837:cluster{dbl[], dbl[]})  [unwired: 1 in]
            n703 = Bundle(w838, w839) -> (w835:cluster{dbl[], dbl[]})  [unwired: 1 in]
            n704 = Build Array(w837, w835) -> (→"_Ref Pump Profiles":cluster{dbl[], dbl[]}[])
          }
          event "_Pump A Plot Selector (T=TMP, F=EPT)": Value Change {
            n705 = event-data() -> ()  [unwired: 1 in, 6 out]
            n706 = property on="_Redraw Pump Timing Plot" class="Bool (strict)"("Val(Sgnl)"=TRUE ("Value (Signaling)")) -> ()  [unwired: 2 in, 2 out]
          }
          event Value Change {
            n707 = event-data() -> ()  [unwired: 1 in, 6 out]
            n708 = property on="_Redraw Pump Timing Plot" class="Bool (strict)"("Val(Sgnl)"=TRUE ("Value (Signaling)")) -> ()  [unwired: 2 in, 2 out]
            n709 = property on="_Redraw Pump Command" class="Bool (strict)"("Val(Sgnl)"=TRUE ("Value (Signaling)")) -> ()  [unwired: 2 in, 2 out]
            n710 = call "Resize DI Command Array.vi"("Command in"="PumpCmd") -> ("Command out"=w861:T7)
            n711 = local write "PumpCmd"(w861) -> ()
          }
          event "_Redraw Pump Timing Plot": Value Change {
            n712 = event-data() -> ()  [unwired: 1 in, 6 out]
            n713 = local read "SimRotations"() -> (w869:u8)
            n714 = local read "SimSpeed"() -> (w870:sgl)
            n715 = local read "SimBatt"() -> (w871:sgl)
            n716 = Bundle By Name(cluster=T34 {"Battery [V]"=13.7, "Engine Speed [RPM]"=1000.0, "Rotations"=2, "Injector Configuration"={"Resistance [Ohm]"=1.0, "Inductance [Henery]"=0.001, "Capacitance [Farad]"=5e-06}, "Description"=""} ("System Configuration"), "Battery [V]"=w871, "Engine Speed [RPM]"=w870, "Rotations"=w869) -> (w866:T34)
            n717 = local read "PumpCmd"() -> (w867:T26)
            n718 = case shown="False" "_Pump A Plot Selector (T=TMP, F=EPT)" {
              tunnel: [w882 w885] -> w868
              tunnel: w867 -> [w883 w884]
              tunnel: w866 -> [w881 _]
              frame False {
                n719 = call "Injection Command Plot - EPT.vi"("System"=w881, "Injection Command"=w883) -> ("Plot"=w882:cluster{"Array":sgl[], "Array":sgl[]}[])  [unwired: 9 in]
              }
              frame True {
                n720 = call "Injection Command Plot - TMP.vi"("Injection Command"=w884) -> ("Plot"=w885:cluster{"Array":sgl[], "Array":sgl[]}[])  [unwired: 10 in]
              }
            }
            "_Pump Timing Plot" <- w868
            n721 = Select(t="Time after Trigger [sec]" ("X Scale.Name Label.Text 2"), s="_Pump A Plot Selector (T=TMP, F=EPT)", f="Timing [DBTDC]" ("X Scale.Name Label.Text 2")) -> (s? t:f=w875:string)
            n722 = Select(t="Trigger" ("Plot.Plot Name 2"), s="_Pump A Plot Selector (T=TMP, F=EPT)", f="Window" ("Plot.Plot Name 2")) -> (s? t:f=w878:string)
            n723 = property on="_Pump Timing Plot" class="XYGraph (strict)"("XScale.NameLbl.Text"=w875, "Active Plot"=u32 0, "Plot.Plot Name"=w878) -> ()  [unwired: 2 in, 2 out]
            n724 = local write "_Redraw Pump Timing Plot"(FALSE ("_Redraw Pump Timing Plot")) -> ()
          }
          event "_Redraw Pump Command": Value Change {
            n725 = event-data() -> ()  [unwired: 1 in, 6 out]
            n726 = local write "_Redraw Pump Command"(FALSE ("_Redraw Pump Command")) -> ()
            n727 = control-ref of="PumpCmd"() -> (w886:refnum<vi>)
            n728 = call "Disable DI Command.vi"("Pump Channel? (F)"=TRUE, "Phase Ref"=w886) -> ()  [unwired: 10 in]
          }
          event "PumpAdaptMode": Value Change {
            n729 = event-data() -> ("NewVal"=w889:bool)  [unwired: 1 in]
            n730 = case shown="False" w889 {
              frame False {
                n731 = property on="_Redraw Pump Command" class="Bool (strict)"("Val(Sgnl)"=TRUE ("Value (Signaling)")) -> ()  [unwired: 2 in, 2 out]
              }
              frame True {
              }
            }
            n732 = Select(t=T30."Disabled and Grayed Out" ("Disabled"), s=w889, f=T30."Enabled" ("Disabled")) -> (s? t:f=w890:T30)
            n733 = property on="PumpCmd" class="Clust (strict)"("DisabledEnum"=w890) -> ()  [unwired: 2 in, 2 out]
          }
          event "_Phase Plot": Plot Attribute Change {
            n734 = event-data() -> ()  [unwired: 1 in, 8 out]
            n735 = property on="_Phase Plot" class="XYGraph (strict)"() -> ("LegNumRows"=w897:u32)  [unwired: 2 in, 2 out]
            n736 = for {
              N: w897 -> [_]
              tunnel: [w900] -> w895 mode=indexing
              tunnel: [w899] -> w896 mode=indexing
              tunnel: [w898] -> w894 mode=indexing
              i -> [w901]
              n737 = property on="_Phase Plot" class="XYGraph (strict)"("Active Plot"=w901) -> ("Plot.Plot Color"=w900:u32, "Plot.Line Width"=w899:u8, "Plot.Line Style"=w898:u8)  [unwired: 2 in, 2 out]
            }
            n738 = property on="PumpPhasePlotColors" class="Arr (strict)"("Val(Sgnl)"=w895) -> ()  [unwired: 2 in, 2 out]
            n739 = property on="InjPhasePlotLineWidths" class="Arr (strict)"("Val(Sgnl)"=w896) -> ()  [unwired: 2 in, 2 out]
            n740 = property on="InjPhasePlotLineTypes" class="Arr (strict)"("Val(Sgnl)"=w894) -> ()  [unwired: 2 in, 2 out]
          }
          event "_Pump Phase Plot": Plot Attribute Change {
            n741 = event-data() -> ()  [unwired: 1 in, 8 out]
            n742 = property on="_Pump Phase Plot" class="XYGraph (strict)"() -> ("LegNumRows"=w905:u32)  [unwired: 2 in, 2 out]
            n743 = for {
              N: w905 -> [_]
              tunnel: [w908] -> w904 mode=indexing
              tunnel: [w907] -> w903 mode=indexing
              tunnel: [w906] -> w902 mode=indexing
              i -> [w909]
              n744 = property on="_Pump Phase Plot" class="XYGraph (strict)"("Active Plot"=w909) -> ("Plot.Plot Color"=w908:u32, "Plot.Line Width"=w907:u8, "Plot.Line Style"=w906:u8)  [unwired: 2 in, 2 out]
            }
            n745 = property on="PumpPhasePlotLineTypes" class="Arr (strict)"("Val(Sgnl)"=w902) -> ()  [unwired: 2 in, 2 out]
            n746 = property on="InjPhasePlotColors" class="Arr (strict)"("Val(Sgnl)"=w904) -> ()  [unwired: 2 in, 2 out]
            n747 = property on="PumpPhasePlotLineWidths" class="Arr (strict)"("Val(Sgnl)"=w903) -> ()  [unwired: 2 in, 2 out]
          }
          event "_Timing Plot": Plot Attribute Change {
            n748 = event-data() -> ()  [unwired: 1 in, 8 out]
            n749 = property on="_Timing Plot" class="XYGraph (strict)"() -> ("LegNumRows"=w913:u32)  [unwired: 2 in, 2 out]
            n750 = for {
              N: w913 -> [_]
              tunnel: [w916] -> w912 mode=indexing
              tunnel: [w915] -> w911 mode=indexing
              tunnel: [w914] -> w910 mode=indexing
              i -> [w917]
              n751 = property on="_Timing Plot" class="XYGraph (strict)"("ActXScl"=w917) -> ("Plot.Plot Color"=w916:u32, "Plot.Line Width"=w915:u8, "Plot.Line Style"=w914:u8)  [unwired: 2 in, 2 out]
            }
            n752 = property on="InjCmdPlotColors" class="Arr (strict)"("Val(Sgnl)"=w912) -> ()  [unwired: 2 in, 2 out]
            n753 = property on="InjCmdPlotLineWidths" class="Arr (strict)"("Val(Sgnl)"=w911) -> ()  [unwired: 2 in, 2 out]
            n754 = property on="InjCmdPlotLineTypes" class="Arr (strict)"("Val(Sgnl)"=w910) -> ()  [unwired: 2 in, 2 out]
          }
          event "_Pump Timing Plot": Plot Attribute Change {
            n755 = event-data() -> ()  [unwired: 1 in, 8 out]
            n756 = property on="_Pump Timing Plot" class="XYGraph (strict)"() -> ("LegNumRows"=w921:u32)  [unwired: 2 in, 2 out]
            n757 = for {
              N: w921 -> [_]
              tunnel: [w924] -> w920 mode=indexing
              tunnel: [w923] -> w919 mode=indexing
              tunnel: [w922] -> w918 mode=indexing
              i -> [w925]
              n758 = property on="_Pump Timing Plot" class="XYGraph (strict)"("ActXScl"=w925) -> ("Plot.Plot Color"=w924:u32, "Plot.Line Width"=w923:u8, "Plot.Line Style"=w922:u8)  [unwired: 2 in, 2 out]
            }
            n759 = property on="PumpCmdPlotColors" class="Arr (strict)"("Val(Sgnl)"=w920) -> ()  [unwired: 2 in, 2 out]
            n760 = property on="PumpCmdPlotLineWidths" class="Arr (strict)"("Val(Sgnl)"=w919) -> ()  [unwired: 2 in, 2 out]
            n761 = property on="PumpCmdPlotLineTypes" class="Arr (strict)"("Val(Sgnl)"=w918) -> ()  [unwired: 2 in, 2 out]
          }
          event "_Redraw Slider": Value Change {
            n762 = event-data() -> ()  [unwired: 1 in, 6 out]
            n763 = local write "_Redraw Slider"(FALSE ("_Redraw Slider")) -> ()
            n764 = local read "_DI Bank_Configuration"() -> (w927:T3)
            n765 = local read "_Bank A?"() -> (w926:bool)
            n766 = local read "State"() -> (w928:T19)
            n767 = call "DI Redraw Boost Slider.vi"("Bank A? (T)"=w926, "DCM System State"=w928, "DI Bank Configuration"=w927) -> ("Levels Slider"=w929:cluster{dbl, dbl, dbl, dbl})  [unwired: 8 in]
            n768 = local write "_BoostSlider"(w929) -> ()
          }
        }
      }
    }
  }
  n769 = First Call?() -> ()  [unwired: 1 out]
